vi "main_control_YJtoy_V2.vi"() -> ()   [LabVIEW 2021]
uses:
  Addons/DAQ_Pulse_Gen/DAQ_Control_2.ctl
  Addons/DAQ_Pulse_Gen/DAQ_Control_1.ctl
  Ver_2/Config_File_Paths_v2.ctl
  Ver_2/ZI_Data_v2.ctl
  Addons/DAQ_Pulse_Gen/DAQ_Control_3 .ctl
  <vilib>/Utility/file.llb/Write Delimited Spreadsheet (DBL).vi
  <vilib>/gmath/NumericalOptimization/Nonlinear Curve Fit LM formula string.vi
  <vilib>/Utility/error.llb/Error Cluster From Error Code.vi
  <vilib>/ErrorRing/Error Ring.xnode
  <vilib>/Utility/Data Type/NI_Data Type.lvlib
  <vilib>/Analysis/NI_AALPro.lvlib
  <vilib>/gmath/NI_Gmath.lvlib
panel:
  out "Initial State Numbers":i32
  out "Process name":string
  out "Initial_state_name":string
  out "tomography rotation memory (priv) 2":cluster{"Time":dbl[], dbl[]}[](array[cluster])
  out "MaxTime":dbl
  out "Process Array":cluster{"Timing 0":dbl[]}[](array[cluster])
  out "tomography rotation memory (priv)":cluster{"Time":dbl[], dbl[]}[](array[cluster])
  in  "pulses type (priv)":string[](array[string])=["None", "Y pi/2", "X pi/2"]
  in  "stop":bool
  in  "Tab Control":T1(tab)=enum."Design QPT"
  out "Config folder":string
  out "Chennel names\nare correct (?)":bool
  out "Channel map":map{string, i32}(c390)
  out "Pulses map [us]":map{string, dbl}(c390)
  out "Sampling data":T2={"Sample Numbers"=20000000, "Sample  Frequency (Hz)"=20000000}
  out "Resource Address":T3={"ZI Address"="DEV714", "VISA Keithley"="KEITHLEY"}
  in  "Save multi-process":bool
  in  "Period number":u32
  in  "Period [us]":dbl
  in  "Name of state (initial_state_)":string
  in  "Name of initial_state":u16(ring) items=["initial_state_01", "initial_state_02", "initial_state_03", "initial_state_04", "initial_state_05", "initial_state_06", "initial_state_07", "initial_state_08", "initial_state_09", "initial_state_10"]
  in  "Run tomography":bool
  in  "Run single FID":bool
  in  "Save for tomography":bool
  in  "Save single sequence":bool
  out "Pulses chart":cluster{dbl[], dbl[]}[](graph)
  in  "Reset sequence":bool
  in  "Channel":u16(ring) items=["LD pump", "LD repump", "LD probe", "pulse X", "pulse Y", "pulse Z", "Keithley ARM", "Keithley TRIG", "Accqusition TRIG", "Nonlinear coil", "None", "Tensor light shift", "pulse ZG"]
  in  "Add pulse advanced":bool
  in  "Physical channels":string[](array[string])
  in  "Add pulse":bool
  in  "Time [us]":dbl
  in  "Z pi/2":bool
  in  "Z pi":bool
  in  "Y pi/2":bool
  in  "Y pi":bool
  in  "X pi/2":bool
  in  "X pi":bool
  in  "Add pumping":bool
  in  "Pumping":T4(ring)
  in  "AOC":bool
  in  "X pi/4":bool
  in  "Save initial state":bool
  in  "Save  process":bool
  in  "Name of process (process_)":string
  in  "Name of process":u16(ring) items=["process_01", "process_02", "process_03", "process_04", "process_05", "process_06", "process_07", "process_08", "process_09", "process_10"]
  in  "Y pi/4":bool
  in  "Z pi/4":bool
  in  "Save multi Sequence":bool
  in  "Clear All processes":bool
  in  "Show Process_List":bool
  in  "Delete the Process":bool
  in  "Run QPT":bool
  in  "initial_state_show":u16(ring) items=["initial_state_01.ini", "initial_state_02.ini", "initial_state_03.ini", "initial_state_04.ini", "initial_state_05.ini", "initial_state_06.ini", "initial_state_07.ini", "initial_state_08.ini", "initial_state_09.ini", "initial_state_10.ini", "initial_state_11.ini"]
  in  "Choose init states":bool
  in  "State_update":bool
  out "State_List":string[](array[string]) caption="The Choosen States"
  in  "Delete init states":bool
  in  "Show init state":bool
  in  "Process_update":bool
  in  "Process_show":u16(ring) caption="initial_state_show" items=["process_01.ini", "process_02.ini", "process_03.ini"]
  out "Pulses chart 2":cluster{dbl[], dbl[]}[](graph)
  out "Pulses chart 3":cluster{dbl[], dbl[]}[](graph)
  in  "Save QPT":bool
  in  "Clear All states":bool
  out "Process_List":string[](array[string]) caption="The Choosen Process"
  in  "Choose the Process":bool
  in  "Multi-FID":bool
  in  "save":bool
  out "Rotation signal 3":cluster{"Time":dbl[], "Array":dbl[]}[](graph)
  out "w":dbl format="%#_3f"
  out "q":dbl format="%#_3f"
  out "g2":dbl format="%#_3f"
  out "g1":dbl format="%#_3f"
  out "C":dbl format="%#_3f"
  out "B":dbl format="%#_3f"
  out "A":dbl format="%#_3f"
  in  "Enum":T5(ring)
  in  "Fit model":bool
  out "Rotation signal":cluster{"Time":dbl[], dbl[]}(graph)
  out "Rotation spectrum":waveform(dbl)[](graph)
  out "Differential signal":cluster{"Time":dbl[], "X":dbl[]}[](graph)
  out "Intensity signal":cluster{"Time":dbl[], dbl[]}(graph)
  out "Polarimeter":dbl(knob) scale=-10.0..10.0
  in  "Run single FID 2":bool
  out "Progress":dbl(slide) scale=0.0..100.0
  in  "Number of repetition":u32=1 min=1 step=1
  in  "Signal in X or Y (?)":bool
  in  "Plot type":u16(ring) items=["None + [ None ]", "None + [ Y pi ]", "None + [ Z(pi/2)+Y(pi) ]", "Y pi/2 + [ None ]", "Y pi/2 + [ Y pi ]", "Y pi/2 + [ Z(pi/2)+Y(pi) ]", "X pi/2 + [ None ]", "X pi/2 + [ Y pi ]", "X pi/2 + [ Z(pi/2)+Y(pi) ]"]
  in  "Save raw data (?)":bool
  in  "Save CYCLOPS data (?)":bool
  out "Rotation signal":cluster{"Time":dbl[], dbl[]}(graph)
  in  "Run tomography 2":bool
  in  "Averaging":u8=1 min=1 step=1
  out "Differential signal":cluster{"Time":dbl[], "X":dbl[]}[](graph)
  out "Intensity signal":cluster{"Time":dbl[], dbl[]}(graph)
  out "Progress":dbl(slide) scale=0.0..100.0
  out "Rotation spectrum":waveform(dbl)[](graph)
  out "Rotation":cluster{"Time":dbl[], dbl[]}(graph)
  in  "Save raw data (?) 2":bool
  in  "Save CYCLOPS data (?) 2":bool
  out "Rotation spectrum 2":waveform(dbl)[](graph)
  out "Rotation signal 2":cluster{"Time":dbl[], dbl[]}(graph)
  out "Differential signal 2":cluster{"Time":dbl[], "X":dbl[]}[](graph)
  out "Intensity signal 2":cluster{"Time":dbl[], dbl[]}(graph)
  out "Single Tomography Progress":dbl(slide) scale=0.0..100.0
  out "Rotation 2":cluster{"Time":dbl[], dbl[]}(graph)
  in  "Averaging 2":u8=1 min=1 step=1
  in  "Run QPT 2":bool
  out "Current_QPT_order":i32
  out "QPT Progress":dbl(slide) scale=0.0..100.0
  # "To change that tab you need to go to block diagram"
  # "Probing will be added during saving"
  # "X"
  # "Y"
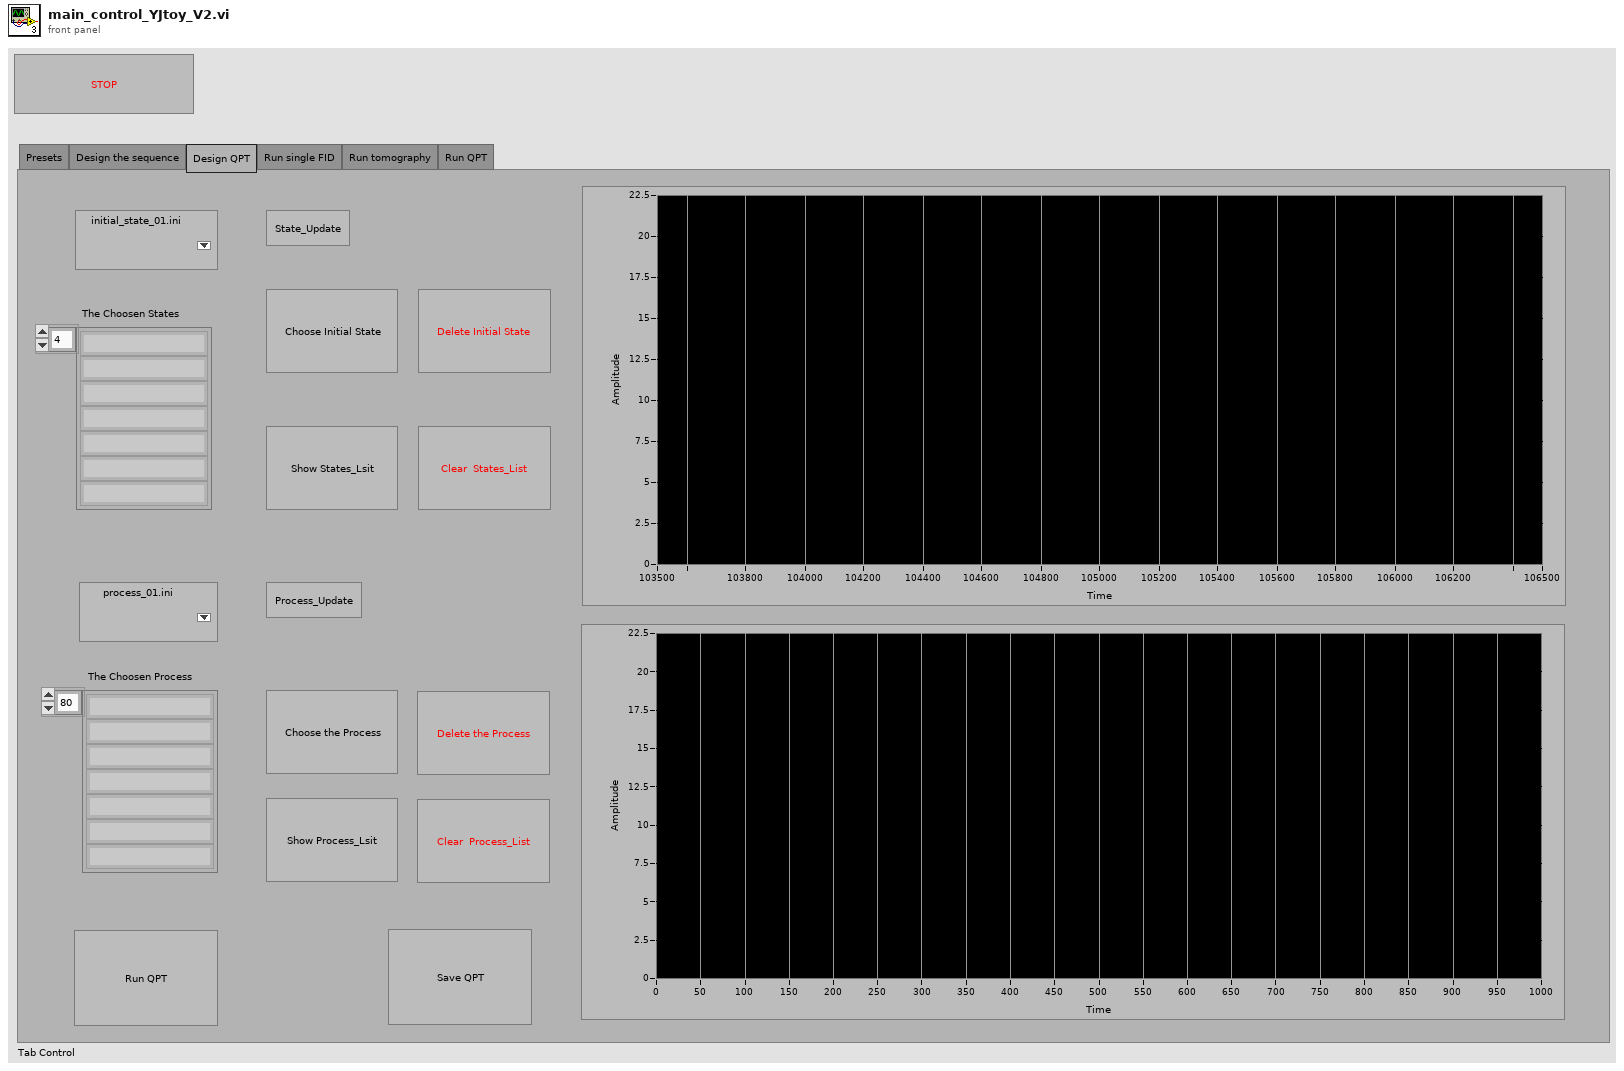
[diagram p1: front panel]
types:
  T1 = enum32{"Presets", "Design the sequence", "Design QPT", "Run single FID", "Run tomography", "Run QPT"}
  T2 = typedef "DAQ_Control_2.ctl" = cluster{"Sample Numbers":u32, "Sample  Frequency (Hz)":u32}
  T3 = cluster{"ZI Address":string, "VISA Keithley":refnum<visa-resource-name>}
  T4 = enum16{"Circular along X", "Linear in Y", "Linear in Z"}
  T5 = enum16{"Full", "A*Sin(w*t+q)*Exp(-g1*t)+C", "B*Exp(-q2*t)+C"}
  T6 = typedef "DAQ_Control_1.ctl" = cluster{"Port 2/line 6":cluster{"Timing 22":dbl[]}, "Port 2/line 5":cluster{"Timing 21":dbl[]}, "Port 2/line 4":cluster{"Timing 20":dbl[]}, "Port 2/line 3":cluster{"Timing 19":dbl[]}, "Port 2/line 2":cluster{"Timing 18":dbl[]}, "Port 2/line 1":cluster{"Timing 17":dbl[]}, "Port 2/line 0":cluster{"Timing 16":dbl[]}, "Port 1/line 7":cluster{"Timing 15":dbl[]}, "Port 1/line 6":cluster{"Timing 14":dbl[]}, "Port 1/line 5":cluster{"Timing 13":dbl[]}, "Port 1/line 4":cluster{"Timing 12":dbl[]}, "Port 1/line 3":cluster{"Timing 11":dbl[]}, "Port 1/line 2":cluster{"Timing 10":dbl[]}, "Port 1/line 1":cluster{"Timing 9":dbl[]}, "Port 1/line 0":cluster{"Timing 8":dbl[]}, "Port 0/line 7":cluster{"Timing 7\n":dbl[]}, "Port 0/line 6":cluster{"Timing 6\n":dbl[]}, "Port 0/line 5":cluster{"Timing 5\n":dbl[]}, "Port 0/line 4":cluster{"Timing 4\n":dbl[]}, "Port 0/line 3":cluster{"Timing 3\n":dbl[]}, "Port 0/line 2":cluster{"Timing 2":dbl[]}, "Port 0/line 1":cluster{"Timing 1\n":dbl[]}, "Port 0/line 0":cluster{"Timing 0":dbl[]}}
  T7 = typedef "Config_File_Paths_v2.ctl" = cluster{"ZI config file (.ini)":string, "Keithley config file (.ini)":string, "DAQ config file (.ini)":string}
  T8 = enum32{"Presets", "Design the sequence", "Design QPT", "Run single FID"}
  T9 = enum8{"Enabled", "Disabled", "Disabled and Grayed Out"}
  T10 = enum32{"Presets", "Design the sequence", "Design QPT", "Run single FID", "Run tomography"}
  T11 = cluster{"model":string, "Parameters":string[], "x":string}
  T12 = typedef "DAQ_Control_3 .ctl" = cluster{"Time Unit":enum16{"NanoSecond", "MicroSecond", "MilliSecond"}}
  T13 = typedef "ZI_Data_v2.ctl" = cluster{"R":dbl[], "Theta":dbl[], "X":dbl[], "Y":dbl[], "AuxIn0":dbl[], "AuxIn1":dbl[], "Frequency":dbl[], "DIO":dbl[], "Time":dbl[]}
  T14 = typedef "Resources_v2.ctl" = cluster{"ZI Handle":T15, "ZI ModHandle":T16, "VISA Keithley":refnum<visa-resource-name>}
  T15 = typedef "Zurich Instruments LabOne.lvlib/ziTypeHandle.ctl" = cluster{"handleValid":bool, "Conn":u64, "Path Prefix":string, "Handle":u64, "Connected":bool, "Clockbase(s)":dbl}
  T16 = typedef "Zurich Instruments LabOne.lvlib/ziTypeModHandle.ctl" = cluster{"handleValid":bool, "Conn":u64, "ModHandle":u64, "moduleID":string, "Path Prefix":string}
  T17 = typedef "Cutted_Data_v2.ctl" = cluster{"X":dbl[], "Y":dbl[], "Time":dbl[]}
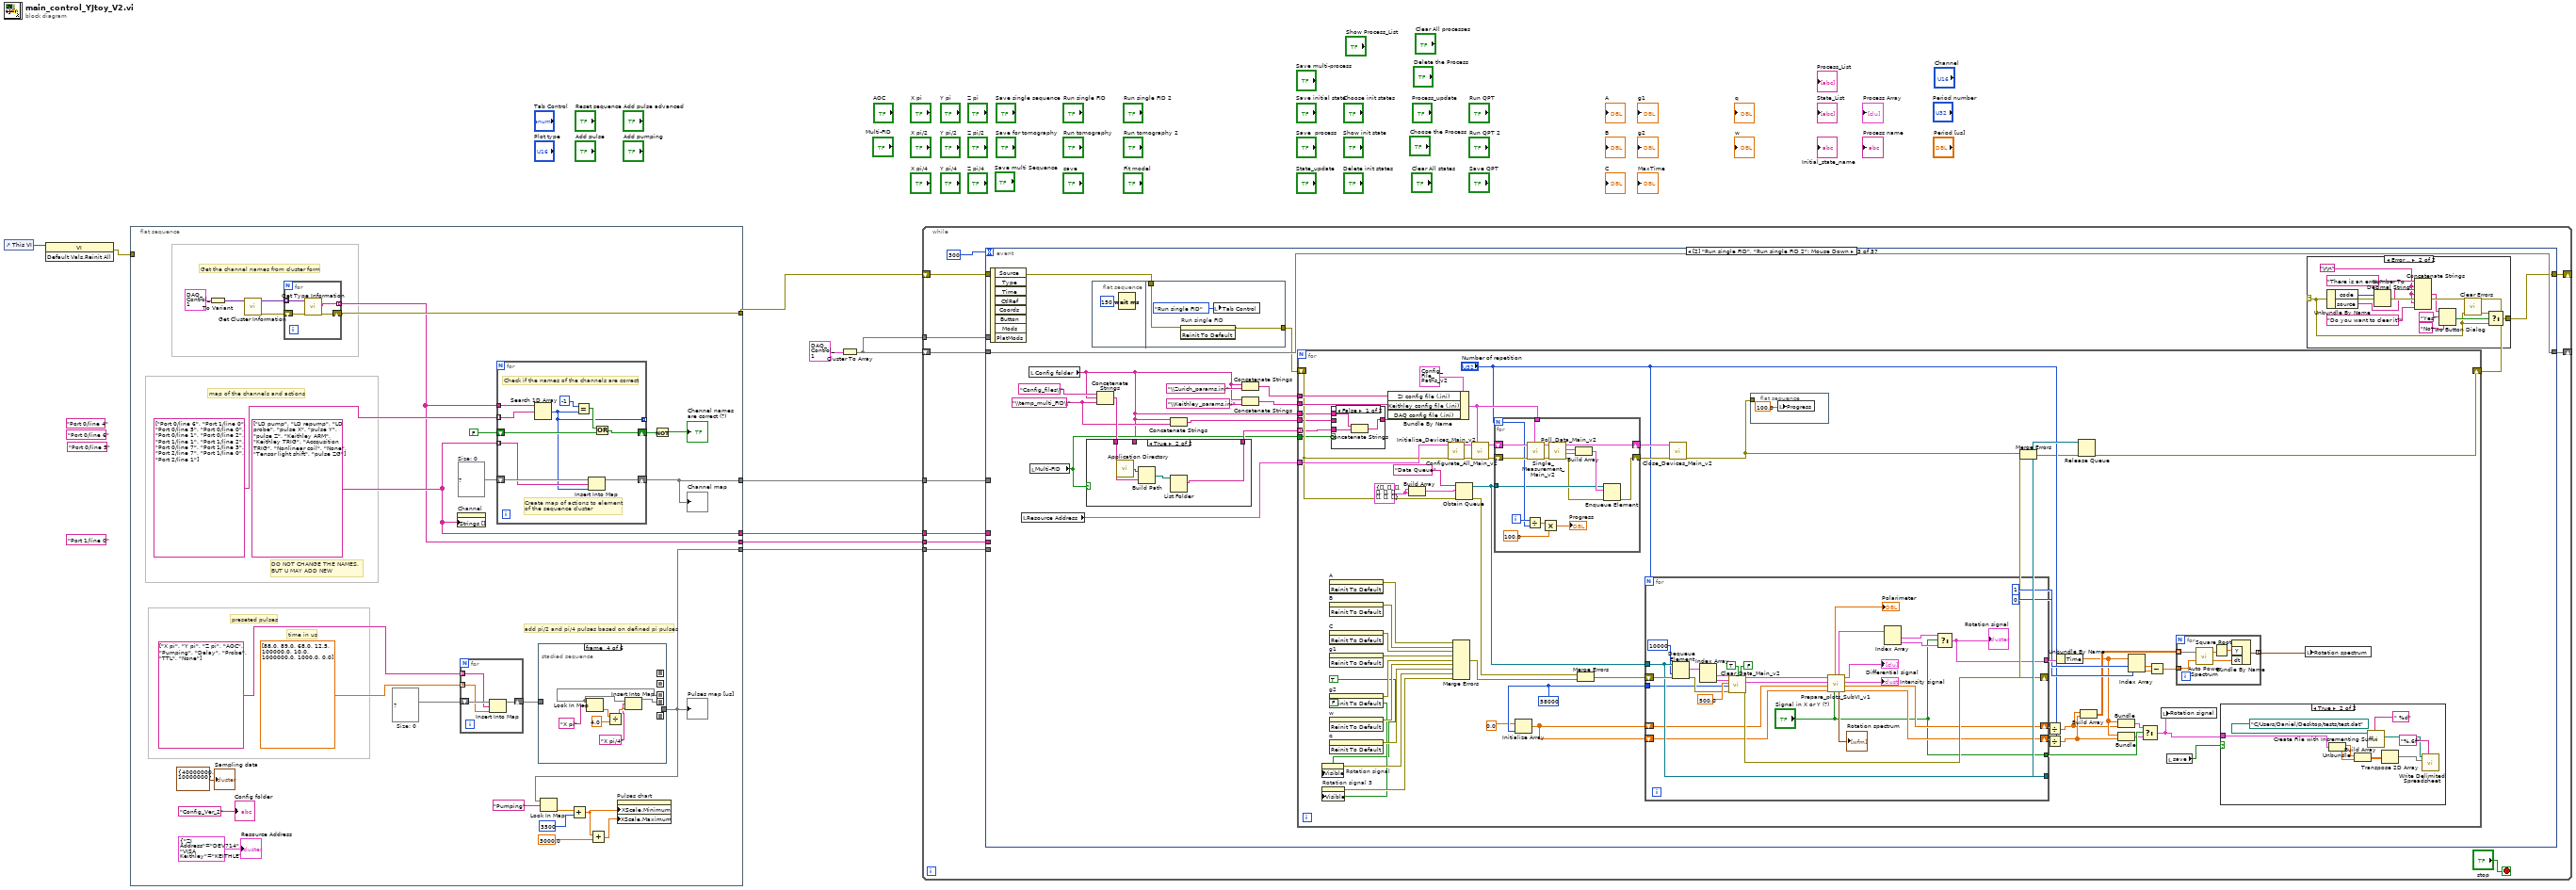
[diagram p0: block diagram]
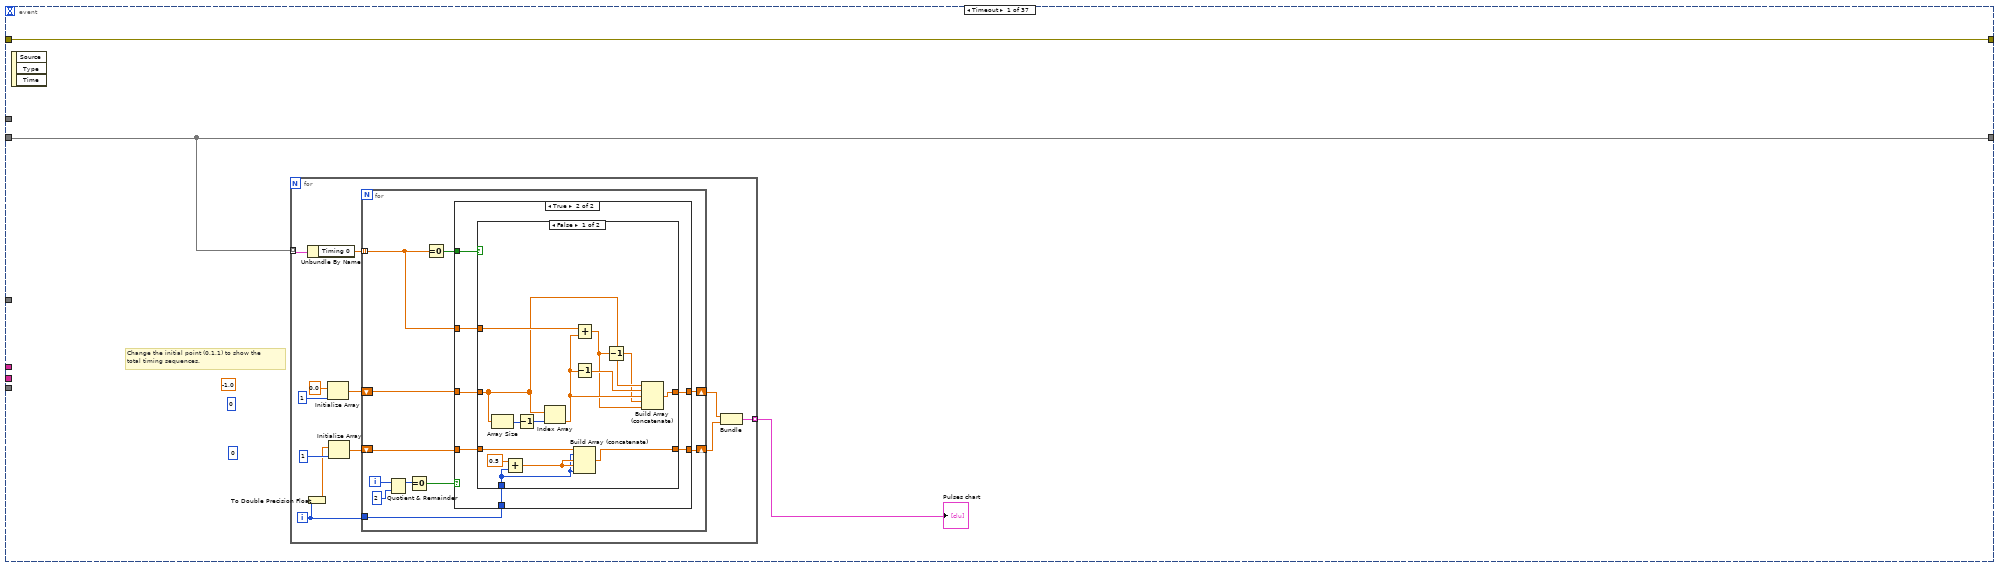
[diagram p2: hidden frame]
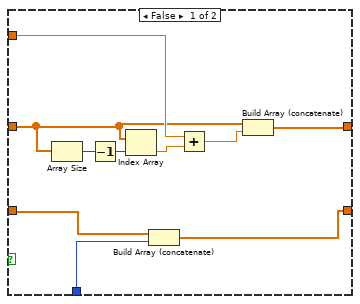
[diagram p3: hidden frame]
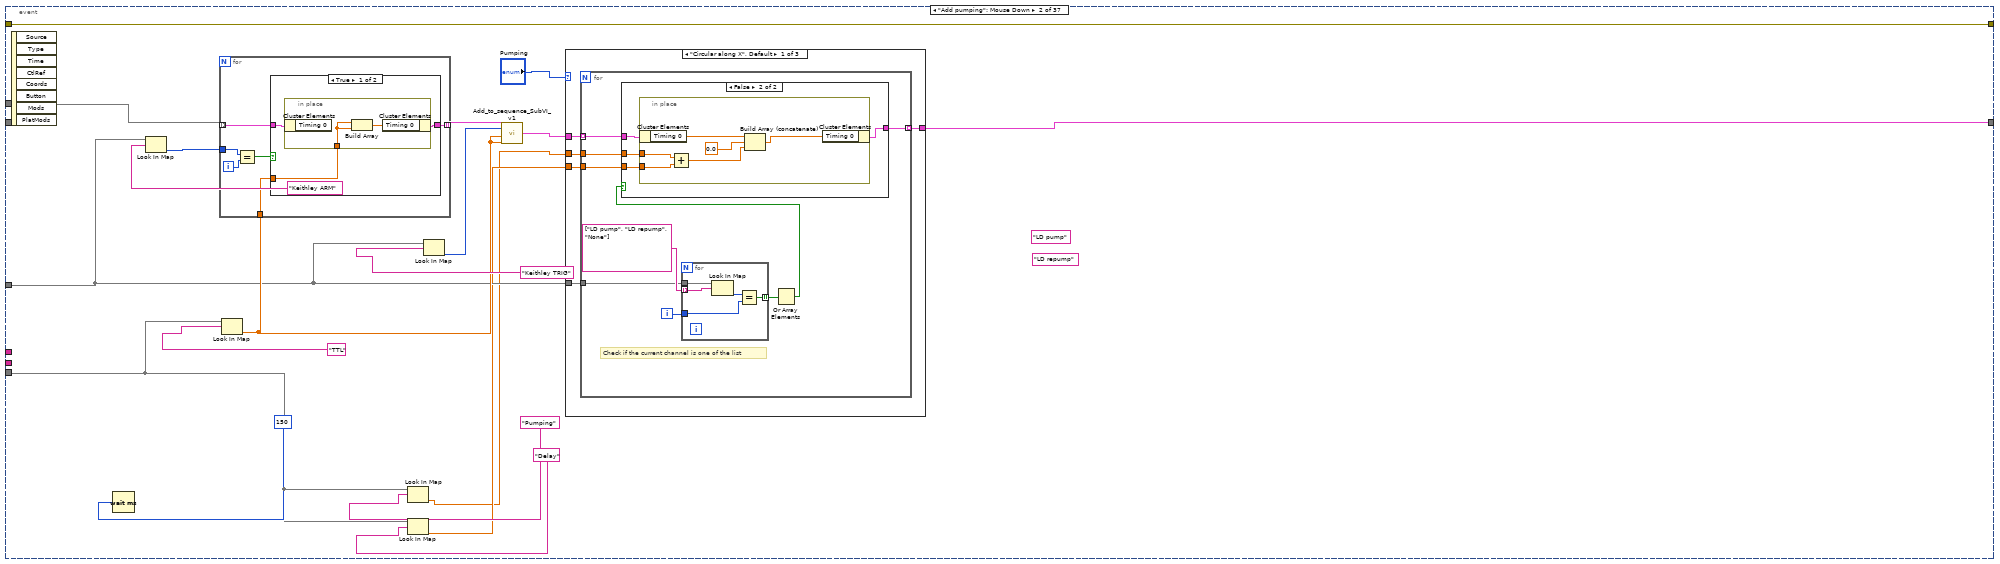
[diagram p5: hidden frame]
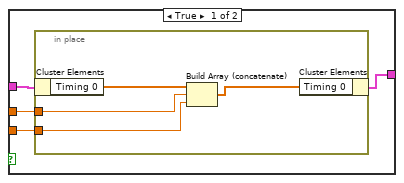
[diagram p6: hidden frame]
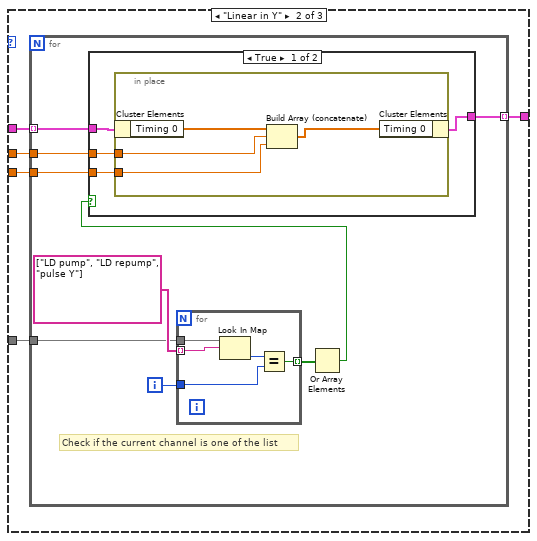
[diagram p7: hidden frame]
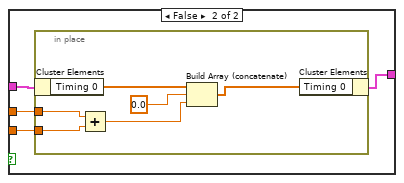
[diagram p8: hidden frame]
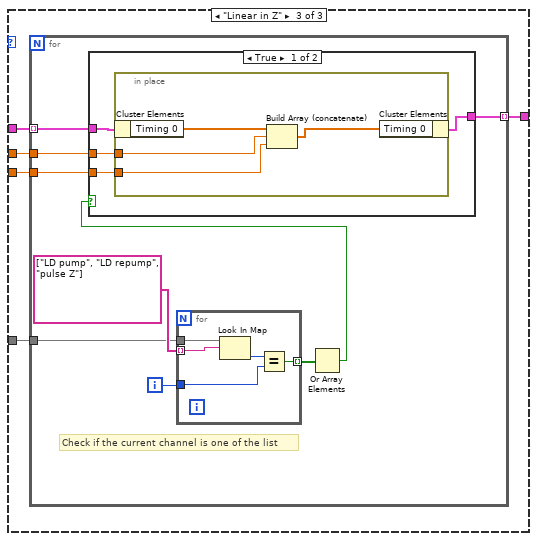
[diagram p9: hidden frame]
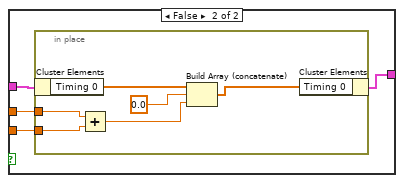
[diagram p10: hidden frame]
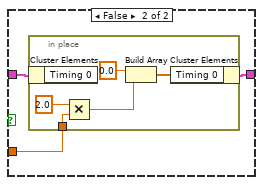
[diagram p11: hidden frame]
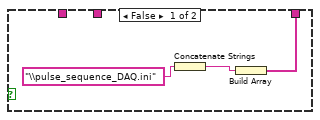
[diagram p12: hidden frame]
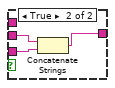
[diagram p13: hidden frame]
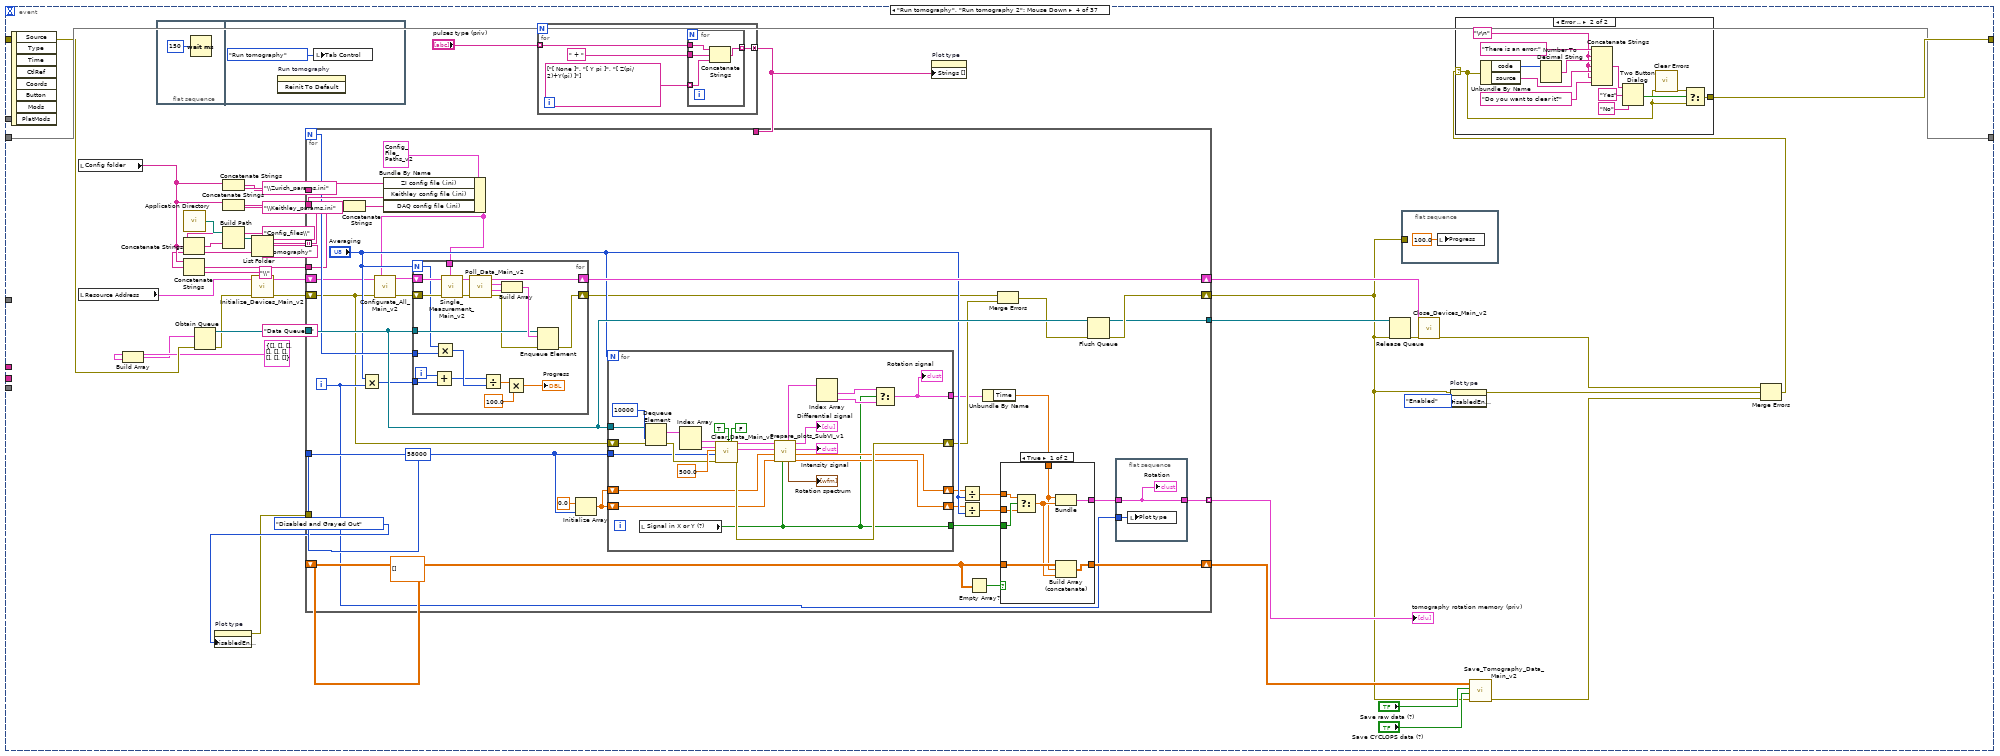
[diagram p16: hidden frame]
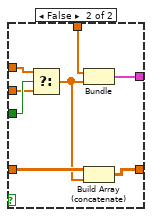
[diagram p17: hidden frame]
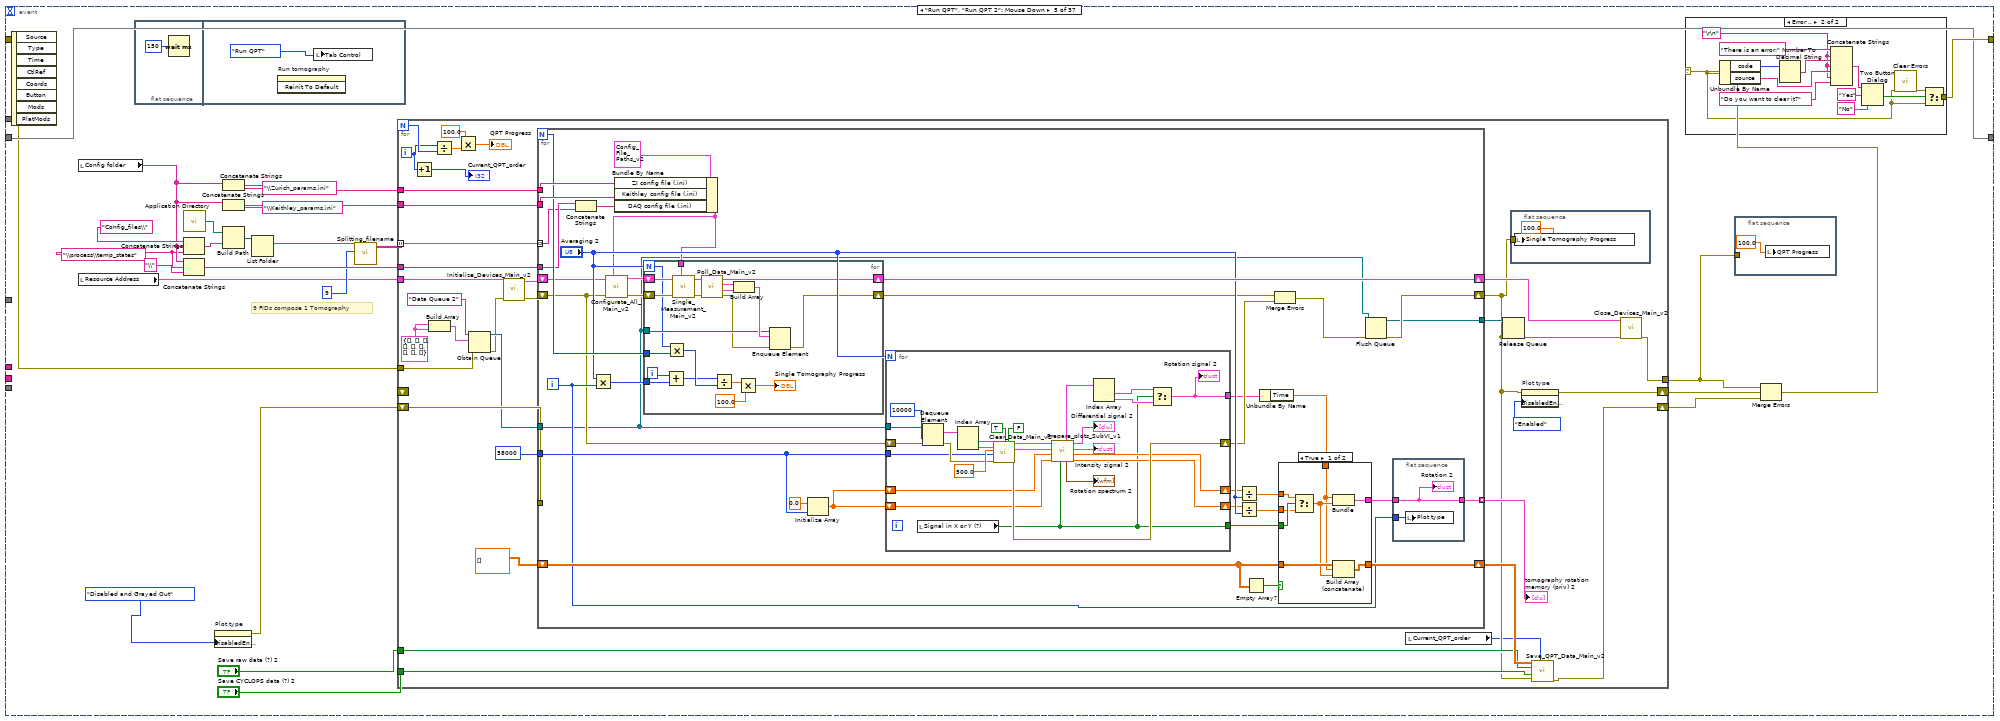
[diagram p19: hidden frame]
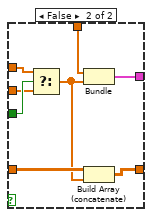
[diagram p20: hidden frame]
diagram:
  (unwired) "Port 0/line 5"
  (unwired) "Port 0/line 4"
  (unwired) "Port 1/line 0"
  (unwired) "Port 0/line 6"
  n1 = control-ref of="This VI"() -> (w2:refnum<vi>)
  n2 = invoke class="VI" method="Default Vals.Reinit All"(reference=w2) -> (error out=w1:errorcluster)  [unwired: 2 in, 2 out]
  n3 = flat-sequence {
    tunnel: [w23] -> w8
    tunnel: [w17] -> w7
    tunnel: [w22] -> w6
    tunnel: [w21] -> w5
    tunnel: [w20] -> w4
    tunnel: w1 -> [_]
    frame #0 {
      w27 = map{string, dbl} {}  # Size: 0
      w29 = map{string, i32} {}  # Size: 0
      w21 = string[] ["LD pump", "LD repump", "LD probe", "pulse X", "pulse Y", "pulse Z", "Keithley ARM", "Keithley TRIG", "Accqusition TRIG", "Nonlinear coil", "None", "Tensor light shift", "pulse ZG"]
      # "DO NOT CHANGE THE NAMES,\nBUT U MAY ADD NEW"
      # "add pi/2 and pi/4 pulses based on defined pi pulses"
      # "preseted pulses"
      # "time in us"
      # "map of the channels and actions"
      # "Get the channel names from cluster form"
      n4 = To Variant(anything=T6 {"Port 2/line 6"={"Timing 22"=[]}, "Port 2/line 5"={"Timing 21"=[]}, "Port 2/line 4"={"Timing 20"=[]}, "Port 2/line 3"={"Timing 19"=[]}, "Port 2/line 2"={"Timing 18"=[]}, "Port 2/line 1"={"Timing 17"=[]}, "Port 2/line 0"={"Timing 16"=[]}, "Port 1/line 7"={"Timing 15"=[]}, "Port 1/line 6"={"Timing 14"=[]}, "Port 1/line 5"={"Timing 13"=[]}, "Port 1/line 4"={"Timing 12"=[]}, "Port 1/line 3"={"Timing 11"=[]}, "Port 1/line 2"={"Timing 10"=[]}, "Port 1/line 1"={"Timing 9"=[]}, "Port 1/line 0"={"Timing 8"=[]}, "Port 0/line 7"={"Timing 7\n"=[]}, "Port 0/line 6"={"Timing 6\n"=[]}, "Port 0/line 5"={"Timing 5\n"=[]}, "Port 0/line 4"={"Timing 4\n"=[]}, "Port 0/line 3"={"Timing 3\n"=[]}, "Port 0/line 2"={"Timing 2"=[]}, "Port 0/line 1"={"Timing 1\n"=[]}, "Port 0/line 0"={"Timing 0"=[]}} ("Sequence")) -> (Variant=w35:variant)
      n5 = call <vilib>:"Get Cluster Information.vi"("variant"=w35) -> ("error out"=w34:errorcluster, "cluster elements"=w33:variant[])  [unwired: 9 in]
      n6 = for {
        tunnel: w33 -> [w96] mode=indexing
        shift-right: [w94] -> w22
        shift-left: w34 -> [w95]
        tunnel: [w93] -> w20 mode=indexing
        n7 = call <vilib>:"Get Type Information.vi"("error in (no error)"=w95, "variant"=w96) -> ("error out"=w94:errorcluster, "name"=w93:string)  [unwired: 5 in, 3 out]
      }
      n8 = property on="Channel" class="Ring (strict)"("Strings []"=w21) -> ()  [unwired: 2 in, 2 out]
      n9 = for {
        shift-right: [w79] -> w24
        shift-left: w27 -> [w82]
        tunnel: string[] ["X pi", "Y pi", "Z pi", "AOC", "Pumping", "Delay", "Probe", "TTL", "None"] -> [w81] mode=indexing
        tunnel: dbl[] [88.0, 89.0, 68.0, 12.5, 100000.0, 10.0, 1000000.0, 1000.0, 0.0] -> [w80] mode=indexing
        n10 = Insert Into Map(map in=w82, key=w81, value=w80) -> (map out=w79:map{string, dbl})  [unwired: 2 out]
      }
      n11 = for {
        tunnel: w20 -> [w92]
        tunnel: string[] ["Port 0/line 6", "Port 1/line 0", "Port 0/line 5", "Port 0/line 0", "Port 0/line 1", "Port 0/line 2", "Port 1/line 1", "Port 1/line 2", "Port 0/line 7", "Port 1/line 3", "Port 2/line 7", "Port 1/line 0", "Port 2/line 1"] -> [w83] mode=indexing
        shift-right: [w88] -> w31
        shift-left: FALSE -> [w89]
        tunnel: [w85] -> _ mode=indexing
        shift-right: [w84] -> w23
        shift-left: w29 -> [w87]
        tunnel: w21 -> [w86] mode=indexing
        # "Create map of actions to element\nof the sequence cluster"
        # "Check if the names of the channels are correct"
        n12 = Search 1D Array(1D array=w92, element=w83) -> (index of element=w85:i32)  [unwired: 1 in]
        n13 = Equal?(x=-1, y=w85) -> (x = y?=w90:bool)
        n14 = Insert Into Map(map in=w87, key=w86, value=w85) -> (map out=w84:map{string, i32})  [unwired: 2 out]
        n15 = Or(x=w90, y=w89) -> (x .or. y?=w88:bool)
      }
      "Channel map" <- w23
      n16 = stacked-sequence {
        seq-local: [w37 _ _ _ _ _] -> [_ w44 _ _ _ _]
        seq-local: [_ w45 _ _ _ _] -> [_ _ w52 _ _ _]
        seq-local: [_ _ w51 _ _ _] -> [_ _ _ w63 _ _]
        seq-local: [_ _ _ w59 _ _] -> [_ _ _ _ w71 _]
        seq-local: [_ _ _ _ w70 _] -> [_ _ _ _ _ w78]
        tunnel: w24 -> [w41 _ _ _ _ _]
        tunnel: [_ _ _ _ _ w77] -> w17
        frame #0 {
          n17 = Look In Map(map=w41, key="X pi") -> (value=w39:dbl)  [unwired: 1 in, 1 out]
          n18 = Divide(x=w39, y=2.0) -> (x/y=w40:dbl)
          n19 = Insert Into Map(map in=w41, key="X pi/2", value=w40) -> (map out=w37:map{string, dbl})  [unwired: 2 out]
        }
        frame #1 {
          n20 = Look In Map(map=w44, key="Y pi") -> (value=w50:dbl)  [unwired: 1 in, 1 out]
          n21 = Divide(x=w50, y=2.0) -> (x/y=w49:dbl)
          n22 = Insert Into Map(map in=w44, key="Y pi/2", value=w49) -> (map out=w45:map{string, dbl})  [unwired: 2 out]
        }
        frame #2 {
          n23 = Look In Map(map=w52, key="Z pi") -> (value=w54:dbl)  [unwired: 1 in, 1 out]
          n24 = Divide(x=w54, y=2.0) -> (x/y=w55:dbl)
          n25 = Insert Into Map(map in=w52, key="Z pi/2", value=w55) -> (map out=w51:map{string, dbl})  [unwired: 2 out]
        }
        frame #3 {
          n26 = Look In Map(map=w63, key="X pi") -> (value=w62:dbl)  [unwired: 1 in, 1 out]
          n27 = Divide(x=w62, y=4.0) -> (x/y=w60:dbl)
          n28 = Insert Into Map(map in=w63, key="X pi/4", value=w60) -> (map out=w59:map{string, dbl})  [unwired: 2 out]
        }
        frame #4 {
          n29 = Look In Map(map=w71, key="Y pi") -> (value=w68:dbl)  [unwired: 1 in, 1 out]
          n30 = Divide(x=w68, y=4.0) -> (x/y=w66:dbl)
          n31 = Insert Into Map(map in=w71, key="Y pi/4", value=w66) -> (map out=w70:map{string, dbl})  [unwired: 2 out]
        }
        frame #5 {
          n32 = Look In Map(map=w78, key="Z pi") -> (value=w75:dbl)  [unwired: 1 in, 1 out]
          n33 = Divide(x=w75, y=4.0) -> (x/y=w73:dbl)
          n34 = Insert Into Map(map in=w78, key="Z pi/4", value=w73) -> (map out=w77:map{string, dbl})  [unwired: 2 out]
        }
      }
      "Pulses map [us]" <- w17
      n35 = Look In Map(map=w17, key="Pumping") -> (value=w19:dbl)  [unwired: 1 in, 1 out]
      n36 = Add(x=w19, y=3500) -> (x+y=w16:dbl)
      n37 = Add(x=w16, y=3000.0) -> (x+y=w14:dbl)
      n38 = property on="Pulses chart" class="XYGraph (strict)"("XScale.Minimum"=w16, "XScale.Maximum"=w14) -> ()  [unwired: 2 in, 2 out]
      n39 = Not(x=w31) -> (.not. x?=→"Chennel names\nare correct (?)":bool)
      "Sampling data" <- T2 {"Sample Numbers"=40000000, "Sample  Frequency (Hz)"=10000000} ("Sampling data")
      "Config folder" <- "Config_Ver_2" ("Filename (ini)")
      "Resource Address" <- T3 {"ZI Address"="DEV714", "VISA Keithley"="KEITHLEY"} ("Resource Address")
    }
  }
  n40 = Cluster To Array(cluster=T6 {"Port 2/line 6"={"Timing 22"=[]}, "Port 2/line 5"={"Timing 21"=[]}, "Port 2/line 4"={"Timing 20"=[]}, "Port 2/line 3"={"Timing 19"=[]}, "Port 2/line 2"={"Timing 18"=[]}, "Port 2/line 1"={"Timing 17"=[]}, "Port 2/line 0"={"Timing 16"=[]}, "Port 1/line 7"={"Timing 15"=[]}, "Port 1/line 6"={"Timing 14"=[]}, "Port 1/line 5"={"Timing 13"=[]}, "Port 1/line 4"={"Timing 12"=[]}, "Port 1/line 3"={"Timing 11"=[]}, "Port 1/line 2"={"Timing 10"=[]}, "Port 1/line 1"={"Timing 9"=[]}, "Port 1/line 0"={"Timing 8"=[]}, "Port 0/line 7"={"Timing 7\n"=[]}, "Port 0/line 6"={"Timing 6\n"=[]}, "Port 0/line 5"={"Timing 5\n"=[]}, "Port 0/line 4"={"Timing 4\n"=[]}, "Port 0/line 3"={"Timing 3\n"=[]}, "Port 0/line 2"={"Timing 2"=[]}, "Port 0/line 1"={"Timing 1\n"=[]}, "Port 0/line 0"={"Timing 0"=[]}} ("Sequence")) -> (array=w3:cluster{"Timing 0":dbl[]}[])
  n41 = while {
    shift-right: [w98] -> _
    shift-left: w3 -> [w107]
    tunnel: w8 -> [w106]
    tunnel: w7 -> [w97]
    shift-right: [w102] -> _
    shift-left: w6 -> [w103]
    tunnel: w5 -> [w101]
    tunnel: w4 -> [w100]
    tunnel: w3 -> [w99]
    stop <- "stop" stop-if-true
    n42 = event shown="[2] \"Run single FID\", \"Run single FID 2\": Mouse Down" {
      selector: _ -> [_ _ _ _ _ _ _ _ _ _ _ _ _ _ _ _ _ _ _ _ _ _ _ _ _ _ _ _ _ _ _ _ _ _ _ _ _]
      dyn-events: _ -> [_ _ _ _ _ _ _ _ _ _ _ _ _ _ _ _ _ _ _ _ _ _ _ _ _ _ _ _ _ _ _ _ _ _ _ _ _]
      timeout: 300 -> [_ _ _ _ _ _ _ _ _ _ _ _ _ _ _ _ _ _ _ _ _ _ _ _ _ _ _ _ _ _ _ _ _ _ _ _ _]
      tunnel: w107 -> [w110 _ w327 w520 w675 w838 _ w1001 w1006 w1018 w1029 w1041 w1053 w1065 w1077 w1089 w1101 w1118 w1146 w1185 w1266 w1397 w1451 w1593 w1640 _ _ _ _ _ _ _ _ _ _ _ _]
      tunnel: w106 -> [_ w172 _ _ _ _ _ w985 w1013 w1025 w1036 w1048 w1060 w1072 w1084 w1096 w1108 w1123 _ w1198 w1268 w1399 w1456 _ _ w1713 _ _ _ _ _ _ _ _ _ _ _]
      tunnel: w97 -> [_ w171 _ _ _ _ _ w983 w1007 w1019 w1034 w1042 w1054 w1066 w1078 w1090 w1102 w1119 w1138 w1195 w1267 w1398 w1455 _ _ w1712 _ _ _ _ _ _ _ _ _ _ _]
      tunnel: [w110 w169 w327 w520 w675 w838 _ w978 w1005 w1017 w1028 w1040 w1052 w1064 w1076 w1088 w1100 w1117 w1135 w1185 _ _ w1451 w1593 w1640 _ _ _ _ _ _ _ _ _ _ _ w2166] -> w98
      tunnel: w103 -> [w109 w185 w326 w514 w657 w839 w881 w989 w1009 w1021 _ w1044 w1056 w1068 w1080 w1092 w1104 w1121 w1142 w1180 w1258 w1389 w1449 w1594 w1641 w1696 w1828 w1923 w2021 w2044 w2059 w2080 w2101 w2129 w2157 w2163 w2167]
      tunnel: [w109 w185 w324 w524 w678 w839 _ w989 w1009 w1021 _ w1044 w1056 w1068 w1080 w1092 w1104 w1121 w1142 w1179 w1265 w1396 w1448 w1595 w1642 w1719 w1827 w1916 w2016 w2039 w2066 w2087 w2098 w2126 w2156 w2162 w2167] -> w102
      tunnel: w101 -> [_ _ _ _ _ _ _ _ _ _ _ _ _ _ _ _ _ w1114 _ _ _ _ _ _ _ _ _ _ _ _ _ _ _ _ _ _ _]
      tunnel: w100 -> [_ _ _ _ _ _ _ _ _ _ _ _ _ _ _ _ _ _ w1144 _ _ _ _ _ _ _ _ _ _ _ _ _ _ _ _ _ _]
      tunnel: w99 -> [_ w168 _ _ _ _ _ _ _ _ _ _ _ _ _ _ _ _ _ _ _ _ _ _ _ _ _ _ _ _ _ _ _ _ _ _ w2166]
      event Timeout {
        (unwired) 0 ("dimension size")
        (unwired) 0 ("dimension size")
        (unwired) -1.0 ("element")
        # "Change the initial point (0,1,1) to show the \ntotal timing sequences."
        n43 = event-data() -> ()  [unwired: 1 in, 3 out]
        n44 = for {
          tunnel: w110 -> [w122] mode=indexing
          tunnel: [w111] -> w108 mode=indexing
          i -> [w114]
          n45 = To Double Precision Float(number=w114) -> (double precision float=w118:dbl)
          n46 = Unbundle By Name(w122) -> ("Timing 0"=w121:dbl[])
          n47 = Initialize Array(0.0 ("element"), 1 ("dimension size")) -> (w115:dbl[])
          n48 = Initialize Array(w118, 1 ("dimension size")) -> (w119:dbl[])
          n49 = for {
            tunnel: w121 -> [w124] mode=indexing
            shift-right: [w126] -> w112
            shift-left: w119 -> [w125]
            shift-right: [w128] -> w113
            shift-left: w115 -> [w127]
            tunnel: w114 -> [w123]
            i -> [w133]
            n50 = Quotient & Remainder(x=w133, y=2) -> (x-y*floor(x/y)=w131:i32)  [unwired: 1 out]
            n51 = Equal To 0?(x=w131) -> (x = 0?=w130:bool)
            n52 = Equal To 0?(x=w124) -> (x = 0?=w129:bool)
            n53 = case shown="True" w130 {
              tunnel: w129 -> [_ w150]
              tunnel: [w134 w149] -> w128
              tunnel: w127 -> [w136 w148]
              tunnel: [w141 w147] -> w126
              tunnel: w125 -> [w142 w146]
              tunnel: w124 -> [w137 w145]
              tunnel: w123 -> [w143 w144]
              frame False {
                n54 = Array Size(array=w136) -> (size(s)=w140:i32)
                n55 = Decrement(x=w140) -> (x-1=w139:i32)
                n56 = Index Array(array=w136, index=w139) -> (element=w138:dbl)
                n57 = Build Array (concatenate)(w142, w143) -> (w141:dbl[])
                n58 = Add(x=w137, y=w138) -> (x+y=w135:dbl)
                n59 = Build Array (concatenate)(w136, w135) -> (w134:dbl[])
              }
              frame True {
                n60 = case shown="False" w150 {
                  tunnel: [w161 w166] -> w149
                  tunnel: w148 -> [w155 w166]
                  tunnel: [w157 w165] -> w147
                  tunnel: w146 -> [w164 w165]
                  tunnel: w145 -> [w162 _]
                  tunnel: w144 -> [w158 _]
                  frame False {
                    n61 = Array Size(array=w155) -> (size(s)=w163:i32)
                    n62 = Add(x=0.5, y=w158) -> (x+y=w159:dbl)
                    n63 = Decrement(x=w163) -> (x-1=w156:i32)
                    n64 = Index Array(array=w155, index=w156) -> (element=w153:dbl)
                    n65 = Add(x=w162, y=w153) -> (x+y=w152:dbl)
                    n66 = Decrement(x=w153) -> (x-1=w154:dbl)
                    n67 = Build Array (concatenate)(w164, w158, w159, w159, w158) -> (w157:dbl[])
                    n68 = Decrement(x=w152) -> (x-1=w151:dbl)
                    n69 = Build Array (concatenate)(w155, w154, w153, w151, w152) -> (w161:dbl[])
                  }
                  frame True {
                  }
                }
              }
            }
          }
          n70 = Bundle(w113, w112) -> (w111:cluster{dbl[], dbl[]})  [unwired: 1 in]
        }
        "Pulses chart" <- w108
      }
      event "Add pumping": Mouse Down {
        (unwired) "LD pump" ("key")
        (unwired) "LD repump" ("key")
        n71 = event-data() -> ()  [unwired: 1 in, 8 out]
        n72 = Wait (ms)(milliseconds to wait=u32 150) -> ()  [unwired: 1 out]
        n73 = Look In Map(map=w172, key="Keithley ARM") -> (value=w182:i32)  [unwired: 1 in, 1 out]
        n74 = Look In Map(map=w171, key="TTL") -> (value=w177:dbl)  [unwired: 1 in, 1 out]
        n75 = for {
          tunnel: w168 -> [w299] mode=indexing
          tunnel: w182 -> [w301]
          tunnel: w177 -> [w298]
          tunnel: [w297] -> w180 mode=indexing
          i -> [w302]
          n76 = Equal?(x=w301, y=w302) -> (x = y?=w300:bool)
          n77 = case shown="True" w300 {
            tunnel: w299 -> [w305 w310]
            tunnel: w298 -> [w304 w309]
            tunnel: [w303 w308] -> w297
            frame True {
              n78 = in-place {
                in-place-border: w304 -> [w307]
                n79 = in-place-cluster #1(w305) -> ()  [unwired: 1 out]
                n80 = Build Array(w307, w307) -> (w306:dbl[])
                n81 = in-place-cluster #1("Timing 0"=w306) -> (w303:cluster{"Timing 0":dbl[]})
              }
            }
            frame False {
              n82 = in-place {
                in-place-border: w309 -> [w313]
                n83 = in-place-cluster #2(w310) -> ()  [unwired: 1 out]
                n84 = Multiply(x=2.0, y=w313) -> (x*y=w311:dbl)
                n85 = Build Array(0.0 ("element"), w311) -> (w315:dbl[])
                n86 = in-place-cluster #2("Timing 0"=w315) -> (w308:cluster{"Timing 0":dbl[]})
              }
            }
          }
        }
        n87 = Look In Map(map=w171, key="Pumping") -> (value=w167:dbl)  [unwired: 1 in, 1 out]
        n88 = Look In Map(map=w171, key="Delay") -> (value=w170:dbl)  [unwired: 1 in, 1 out]
        n89 = Look In Map(map=w172, key="Keithley TRIG") -> (value=w178:i32)  [unwired: 1 in, 1 out]
        n90 = call "Add_to_sequence_SubVI_v1.vi"("Delay [us]"=w177, "Pulse length [us]"=w177, "Channel number"=w178, "Array sequence in"=w180) -> ("Array sequence out"=w175:cluster{"Timing 0":dbl[]}[])
        n91 = case shown="\"Circular along X\", Default" "Pumping" {
          tunnel: w175 -> [w190 w227 w264]
          tunnel: w172 -> [w189 w226 w263]
          tunnel: w167 -> [w188 w225 w262]
          tunnel: w170 -> [w187 w224 w261]
          tunnel: [w186 w223 w260] -> w169
          frame "Circular along X", Default {
            n92 = for {
              tunnel: w190 -> [w194] mode=indexing
              tunnel: w189 -> [w196]
              tunnel: w188 -> [w193]
              tunnel: w187 -> [w192]
              tunnel: [w191] -> w186 mode=indexing
              i -> [w197]
              # "Check if the current channel is one of the list"
              n93 = for {
                tunnel: w196 -> [w221]
                tunnel: w197 -> [w220]
                tunnel: [w219] -> w199 mode=indexing
                tunnel: string[] ["LD pump", "LD repump", "None"] -> [w218] mode=indexing
                n94 = Look In Map(map=w221, key=w218) -> (value=w222:i32)  [unwired: 1 in, 1 out]
                n95 = Equal?(x=w222, y=w220) -> (x = y?=w219:bool)
              }
              n96 = Or Array Elements(Boolean array=w199) -> (logical OR=w195:bool)
              n97 = case shown="False" w195 {
                tunnel: w194 -> [w203 w211]
                tunnel: w193 -> [w202 w210]
                tunnel: w192 -> [w201 w209]
                tunnel: [w200 w208] -> w191
                frame True {
                  n98 = in-place {
                    in-place-border: w202 -> [w206]
                    in-place-border: w201 -> [w205]
                    n99 = in-place-cluster #3(w203) -> ("Timing 0"=w207:dbl[])
                    n100 = Build Array (concatenate)(w207, w206, w205) -> (w204:dbl[])
                    n101 = in-place-cluster #3("Timing 0"=w204) -> (w200:cluster{"Timing 0":dbl[]})
                  }
                }
                frame False {
                  n102 = in-place {
                    in-place-border: w210 -> [w215]
                    in-place-border: w209 -> [w214]
                    n103 = in-place-cluster #4(w211) -> ("Timing 0"=w217:dbl[])
                    n104 = Add(x=w215, y=w214) -> (x+y=w213:dbl)
                    n105 = Build Array (concatenate)(w217, 0.0 ("element"), w213) -> (w216:dbl[])
                    n106 = in-place-cluster #4("Timing 0"=w216) -> (w208:cluster{"Timing 0":dbl[]})
                  }
                }
              }
            }
          }
          frame "Linear in Y" {
            n107 = for {
              tunnel: w227 -> [w231] mode=indexing
              tunnel: w226 -> [w233]
              tunnel: w225 -> [w230]
              tunnel: w224 -> [w229]
              tunnel: [w228] -> w223 mode=indexing
              i -> [w234]
              # "Check if the current channel is one of the list"
              n108 = for {
                tunnel: w233 -> [w258]
                tunnel: w234 -> [w257]
                tunnel: [w256] -> w236 mode=indexing
                tunnel: string[] ["LD pump", "LD repump", "pulse Y"] -> [w255] mode=indexing
                n109 = Look In Map(map=w258, key=w255) -> (value=w259:i32)  [unwired: 1 in, 1 out]
                n110 = Equal?(x=w259, y=w257) -> (x = y?=w256:bool)
              }
              n111 = Or Array Elements(Boolean array=w236) -> (logical OR=w232:bool)
              n112 = case shown="True" w232 {
                tunnel: w231 -> [w240 w248]
                tunnel: w230 -> [w239 w247]
                tunnel: w229 -> [w238 w246]
                tunnel: [w237 w245] -> w228
                frame True {
                  n113 = in-place {
                    in-place-border: w239 -> [w243]
                    in-place-border: w238 -> [w242]
                    n114 = in-place-cluster #5(w240) -> ("Timing 0"=w244:dbl[])
                    n115 = Build Array (concatenate)(w244, w243, w242) -> (w241:dbl[])
                    n116 = in-place-cluster #5("Timing 0"=w241) -> (w237:cluster{"Timing 0":dbl[]})
                  }
                }
                frame False {
                  n117 = in-place {
                    in-place-border: w247 -> [w252]
                    in-place-border: w246 -> [w251]
                    n118 = in-place-cluster #6(w248) -> ("Timing 0"=w254:dbl[])
                    n119 = Add(x=w252, y=w251) -> (x+y=w250:dbl)
                    n120 = Build Array (concatenate)(w254, 0.0 ("element"), w250) -> (w253:dbl[])
                    n121 = in-place-cluster #6("Timing 0"=w253) -> (w245:cluster{"Timing 0":dbl[]})
                  }
                }
              }
            }
          }
          frame "Linear in Z" {
            n122 = for {
              tunnel: w264 -> [w268] mode=indexing
              tunnel: w263 -> [w270]
              tunnel: w262 -> [w267]
              tunnel: w261 -> [w266]
              tunnel: [w265] -> w260 mode=indexing
              i -> [w271]
              # "Check if the current channel is one of the list"
              n123 = for {
                tunnel: w270 -> [w295]
                tunnel: w271 -> [w294]
                tunnel: [w293] -> w273 mode=indexing
                tunnel: string[] ["LD pump", "LD repump", "pulse Z"] -> [w292] mode=indexing
                n124 = Look In Map(map=w295, key=w292) -> (value=w296:i32)  [unwired: 1 in, 1 out]
                n125 = Equal?(x=w296, y=w294) -> (x = y?=w293:bool)
              }
              n126 = Or Array Elements(Boolean array=w273) -> (logical OR=w269:bool)
              n127 = case shown="True" w269 {
                tunnel: w268 -> [w277 w285]
                tunnel: w267 -> [w276 w284]
                tunnel: w266 -> [w275 w283]
                tunnel: [w274 w282] -> w265
                frame True {
                  n128 = in-place {
                    in-place-border: w276 -> [w280]
                    in-place-border: w275 -> [w279]
                    n129 = in-place-cluster #7(w277) -> ("Timing 0"=w281:dbl[])
                    n130 = Build Array (concatenate)(w281, w280, w279) -> (w278:dbl[])
                    n131 = in-place-cluster #7("Timing 0"=w278) -> (w274:cluster{"Timing 0":dbl[]})
                  }
                }
                frame False {
                  n132 = in-place {
                    in-place-border: w284 -> [w289]
                    in-place-border: w283 -> [w288]
                    n133 = in-place-cluster #8(w285) -> ("Timing 0"=w291:dbl[])
                    n134 = Add(x=w289, y=w288) -> (x+y=w287:dbl)
                    n135 = Build Array (concatenate)(w291, 0.0 ("element"), w287) -> (w290:dbl[])
                    n136 = in-place-cluster #8("Timing 0"=w290) -> (w282:cluster{"Timing 0":dbl[]})
                  }
                }
              }
            }
          }
        }
      }
      event "Run single FID", "Run single FID 2": Mouse Down {
        w319 = "\\temp_multi_FID\\" ("string")
        n137 = event-data() -> ()  [unwired: 1 in, 8 out]
        n138 = local read "Resource Address"() -> (w332:T3)
        n139 = local read "Config folder"() -> (w316:string)
        n140 = local read "Multi-FID"() -> (w317:bool)
        n141 = flat-sequence {
          tunnel: w326 -> [w484]
          tunnel: [w483] -> w325
          frame #0 {
            n142 = Wait (ms)(milliseconds to wait=u32 150) -> ()  [unwired: 1 out]
          }
          frame #1 {
            n143 = invoke on="Run single FID" class="Bool (strict)" method="Reinit To Default"(error in=w484) -> (error out=w483:errorcluster)  [unwired: 2 in, 2 out]
            n144 = local write "Tab Control"(T8."Run single FID" ("Tab Control")) -> ()
          }
        }
        n145 = Concatenate Strings("Config_files\\" ("string"), w316, w319) -> (w320:string)
        n146 = case shown="True" w317 {
          tunnel: w320 -> [_ w337]
          tunnel: [w333 w336] -> w322
          tunnel: w316 -> [_ _]
          frame False {
            n147 = Concatenate Strings("\\pulse_sequence_DAQ.ini" ("string")) -> (w334:string)
            n148 = Build Array(w334) -> (w333:string[])
          }
          frame True {
            n149 = call <vilib>:"Application Directory.vi"() -> ("Application Directory"=w338:path)
            n150 = Build Path(base path=w338, name or relative path=w337) -> (appended path=w339:path)
            n151 = List Folder(path=w339) -> (filenames=w336:string[])  [unwired: 3 in, 3 out]
          }
        }
        n152 = Concatenate Strings(w316, w319) -> (w318:string)
        n153 = Concatenate Strings(w316, "\\Zurich_params.ini" ("string")) -> (w328:string)
        n154 = Concatenate Strings(w316, "\\Keithley_params.ini" ("string")) -> (w329:string)
        n155 = for {
          tunnel: w332 -> [w401]
          tunnel: w329 -> [w397]
          tunnel: w328 -> [w396]
          shift-right: [w359] -> w323
          shift-left: w325 -> [w389]
          tunnel: w322 -> [w344] mode=indexing
          tunnel: w318 -> [w342]
          tunnel: w317 -> [w341]
          tunnel: w316 -> [w340]
          w363 = T13 {"R"=[], "Theta"=[], "X"=[], "Y"=[], "AuxIn0"=[], "AuxIn1"=[], "Frequency"=[], "DIO"=[], "Time"=[]} ("ZI Data")
          w386 = u16 58000 ("Fixed Number Of Points")
          n156 = property on="Rotation signal" class="XYGraph (strict)"("Visible"=TRUE) -> (error out=w355:errorcluster)  [unwired: 2 in, 1 out]
          n157 = property on="Rotation signal 3" class="XYGraph (strict)"("Visible"=FALSE) -> (error out=w356:errorcluster)  [unwired: 2 in, 1 out]
          n158 = invoke on="A" class="DigNum (strict)" method="Reinit To Default"() -> (error out=w351:errorcluster)  [unwired: 3 in, 2 out]
          n159 = invoke on="B" class="DigNum (strict)" method="Reinit To Default"() -> (error out=w350:errorcluster)  [unwired: 3 in, 2 out]
          n160 = invoke on="C" class="DigNum (strict)" method="Reinit To Default"() -> (error out=w349:errorcluster)  [unwired: 3 in, 2 out]
          n161 = invoke on="g1" class="DigNum (strict)" method="Reinit To Default"() -> (error out=w348:errorcluster)  [unwired: 3 in, 2 out]
          n162 = invoke on="g2" class="DigNum (strict)" method="Reinit To Default"() -> (error out=w352:errorcluster)  [unwired: 3 in, 2 out]
          n163 = invoke on="w" class="DigNum (strict)" method="Reinit To Default"() -> (error out=w353:errorcluster)  [unwired: 3 in, 2 out]
          n164 = invoke on="q" class="DigNum (strict)" method="Reinit To Default"() -> (error out=w354:errorcluster)  [unwired: 3 in, 2 out]
          n165 = case shown="False" w341 {
            tunnel: w344 -> [w404 w407]
            tunnel: [w402 w406] -> w343
            tunnel: w342 -> [_ w405]
            tunnel: w340 -> [w403 _]
            frame False {
              n166 = Concatenate Strings(w403, w404) -> (w402:string)
            }
            frame True {
              n167 = Concatenate Strings(w405, w407) -> (w406:string)
            }
          }
          n168 = Bundle By Name(cluster=T7 {"ZI config file (.ini)"="Config_Ver_2\\Zurich_params.ini", "Keithley config file (.ini)"="Config_Ver_2\\Keithley_params.ini", "DAQ config file (.ini)"="Config_Ver_2\\pulse_sequence_DAQ.ini"} ("Config files paths"), "ZI config file (.ini)"=w396, "Keithley config file (.ini)"=w397, "DAQ config file (.ini)"=w343) -> (w393:T7)
          n169 = Build Array(w363, w363) -> (w362:T13[])
          n170 = call "Initialize_Devices_Main_v2.vi"("error in"=w389, "Resource Address"=w401) -> ("error out"=w399:errorcluster, "Resources"=w400:T14)  [unwired: 8 in]
          n171 = Merge Errors(w351, w350, w349, w348, w352, w353, w354, w355, w356) -> (w345:errorcluster)
          n172 = Obtain Queue(name (unnamed)="Data Queue", element data type=w362, error in (no error)=w389) -> (queue out=w388:refnum<queue>, error out=w365:errorcluster)  [unwired: 2 in, 1 out]
          n173 = call "Configurate_All_Main_v2.vi"("Resources in"=w400, "Config files paths"=w393, "error in"=w399) -> ("Resources out"=w395:T14, "error out"=w394:errorcluster)  [unwired: 6 in, 5 out]
          n174 = for {
            N: "Number of repetition" -> [w460]
            tunnel: w393 -> [w465]
            shift-right: [w464] -> w392
            shift-left: w395 -> [w467]
            shift-right: [w452] -> w391
            shift-left: w394 -> [w466]
            tunnel: w388 -> [w455]
            i -> [w461]
            n175 = Divide(x=w461, y=w460) -> (x/y=w458:dbl)
            n176 = call "Single_Measurement_Main_v2.vi"("Config files paths"=w465, "error in"=w466, "Resources in"=w467) -> ("error out"=w462:errorcluster, "Resources out"=w463:T14)  [unwired: 6 in, 1 out]
            n177 = Multiply(x=w458, y=100.0) -> (x*y=→"Progress":dbl)
            n178 = call "Poll_Data_Main_v2.vi"("error in"=w462, "Resources in"=w463) -> ("error out"=w453:errorcluster, "ZI Data 3"=w454:T13, "ZI Data 0"=w451:T13, "Resources out"=w464:T14)  [unwired: 6 in]
            n179 = Build Array(w451, w454) -> (w456:T13[])
            n180 = Enqueue Element(queue=w455, element=w456, error in (no error)=w453) -> (error out=w452:errorcluster)  [unwired: 1 in, 2 out]
          }
          n181 = Initialize Array(0.0 ("element"), w386) -> (w384:dbl[])
          n182 = Merge Errors(w365, w345) -> (w364:errorcluster)
          n183 = for {
            N: "Number of repetition" -> [_]
            tunnel: w388 -> [w444]
            shift-right: [w441] -> w361
            shift-left: w364 -> [w446]
            tunnel: [w444] -> w387
            shift-right: [w434] -> w369
            shift-left: w384 -> [w437]
            tunnel: w386 -> [w440]
            shift-right: [w435] -> w370
            shift-left: w384 -> [w436]
            tunnel: [w423] -> w383
            tunnel: ["Signal in X or Y (?)"] -> w382
            n184 = Dequeue Element(queue=w444, timeout in ms (-1)=10000, error in (no error)=w446) -> (element=w445:T13[], error out=w442:errorcluster)  [unwired: 2 out]
            n185 = Index Array(array=w445) -> (element #1=w425:T13, element #2=w443:T13)  [unwired: 2 in]
            n186 = call "Clear_Data_Main_v2.vi"("ZI Data 0"=w425, "ZI Data 3"=w443, "Time Of Collected Data (ms)"=500.0, 3:"Fixed Number Of Points"=w440, "error in"=w442, 10:"Fixed Number Of Points"=TRUE ("Fixed Number Of Points"), "Check Phase Mismatch"=FALSE) -> ("Cutted Data 0"=w439:T17, "Cutted Data 3"=w438:T17, "error out"=w441:errorcluster)  [unwired: 7 in, 3 out]
            n187 = call "Prepare_plots_SubVI_v1.vi"("Signal in X or Y (?)"="Signal in X or Y (?)", "Y rot avg in"=w436, "X rot avg in"=w437, "Cutted Data 3"=w438, "Cutted Data 0"=w439) -> ("Y rot avg out"=w435:dbl[], "X rot avg out"=w434:dbl[], "Monitor"=→"Intensity signal":cluster{"Time":dbl[], dbl[]}, "RF out"=→"Differential signal":cluster{"Time":dbl[], "Y":dbl[]}[], "Rotation spectrum"=→"Rotation spectrum":waveform(dbl)[], "Rotation"=w430:cluster{"Time":dbl[], dbl[]}[], "Polarimeter"=→"Polarimeter":dbl)
            n188 = Index Array(array=w430) -> (element #1=w429:cluster{"Time":dbl[], dbl[]}, element #2=w428:cluster{"Time":dbl[], dbl[]})  [unwired: 2 in]
            n189 = Select(t=w429, s="Signal in X or Y (?)", f=w428) -> (s? t:f=w423:cluster{"Time":dbl[], dbl[]})
            "Rotation signal" <- w423
          }
          n190 = call "Close_Devices_Main_v2.vi"("error in"=w391, "Resources"=w392) -> ("error out"=w371:errorcluster)  [unwired: 9 in]
          n191 = flat-sequence {
            tunnel: w371 -> [_]
            frame #0 {
              n192 = local write "Progress"(100.0 ("Progress")) -> ()
            }
          }
          n193 = Merge Errors(w371, w361) -> (w360:errorcluster)
          n194 = Divide(x=w369, y="Number of repetition") -> (x/y=w367:dbl[])
          n195 = Divide(x=w370, y="Number of repetition") -> (x/y=w368:dbl[])
          n196 = Unbundle By Name(w383) -> ("Time"=w374:dbl[])
          n197 = Release Queue(queue=w387, error in (no error)=w360) -> (error out=w359:errorcluster)  [unwired: 1 in, 2 out]
          n198 = Build Array(w367, w368) -> (w375:dbl[][])
          n199 = Bundle("Time"=w374, w367) -> (w380:cluster{"Time":dbl[], dbl[]})  [unwired: 1 in]
          n200 = Bundle("Time"=w374, w368) -> (w381:cluster{"Time":dbl[], dbl[]})  [unwired: 1 in]
          n201 = Index Array(array=w374, index #1=1 ("index"), index #2=0 ("index")) -> (element #1=w378:dbl, element #2=w379:dbl)
          n202 = Select(t=w380, s=w382, f=w381) -> (s? t:f=w357:cluster{"Time":dbl[], dbl[]})
          n203 = Subtract(x=w378, y=w379) -> (x-y=w373:dbl)
          n204 = local write "Rotation signal"(w357) -> ()
          n205 = local read "save"() -> (w358:bool)
          n206 = for {
            tunnel: w375 -> [w422] mode=indexing
            tunnel: [w420] -> w372 mode=indexing
            tunnel: w373 -> [w417]
            n207 = call <vilib>:"Auto Power Spectrum.vi"("dt"=w417, "Signal (V)"=w422) -> ("df"=w421:dbl, "Power Spectrum (V^2 rms)"=w419:dbl[])
            n208 = Square Root(x=w419) -> (sqrt(x)=w418:dbl[])
            n209 = Bundle By Name("Y"=w418, "dt"=w421) -> (w420:waveform(dbl))  [unwired: 1 in]
          }
          n210 = case shown="True" w358 {
            tunnel: w357 -> [_ w416]
            frame False {
            }
            frame True {
              n211 = Unbundle(w416) -> ("Time"=w415:dbl[], w414:dbl[])
              n212 = Build Array(w415, w414) -> (w413:dbl[][])
              n213 = call <vilib>:"Create File with Incrementing Suffix.vi"("format string (\" (%d)\")"=" %d" ("format string (\" (%d)\")"), "file path"=path "C:/Users/Daniel/Desktop/tests/test.dat") -> ("actual path"=w410:path)  [unwired: 7 in, 2 out]
              n214 = Transpose 2D Array(2D array=w413) -> (transposed array=w412:dbl[][])
              n215 = call-poly <vilib>:"Write Delimited Spreadsheet.vi"("file path (dialog if empty)"=w410, "format (%.3f)"="%.6f", "2D data"=w412) -> ()  [unwired: 11 in, 2 out]
            }
          }
          n216 = local write "Rotation spectrum"(w372) -> ()
        }
        n217 = case shown="Error .." w323 {
          selector: w323 -> [w468 w469]
          tunnel: [w468 w472] -> w324
          frame No Error {
          }
          frame Error {
            w477 = "\r\n"
            n218 = Unbundle By Name(w469) -> ("code"=w480:i32, "source"=w478:string)
            n219 = Number To Decimal String(number=w480) -> (decimal integer string=w479:string)  [unwired: 1 in]
            n220 = Concatenate Strings("There is an error:" ("string"), w477, w479, w477, w478, w477, "Do you want to clear it?" ("string")) -> (w473:string)
            n221 = Two Button Dialog(message=w473, 1:"No" ("F button name (\"Cancel\")"), 2:"Yes" ("T button name (\"OK\")")) -> (T button?=w471:bool)
            n222 = call <vilib>:"Clear Errors.vi"("error in (no error)"=w469) -> ("error out"=w470:errorcluster)  [unwired: 5 in, 1 out]
            n223 = Select(t=w470, s=w471, f=w469) -> (s? t:f=w472:errorcluster)
          }
        }
      }
      event "Run tomography", "Run tomography 2": Mouse Down {
        w494 = T13 {"R"=[], "Theta"=[], "X"=[], "Y"=[], "AuxIn0"=[], "AuxIn1"=[], "Frequency"=[], "DIO"=[], "Time"=[]} ("ZI Data")
        w489 = "\\tomography" ("string")
        n224 = event-data() -> ()  [unwired: 1 in, 8 out]
        n225 = local read "Config folder"() -> (w490:string)
        n226 = local read "Resource Address"() -> (w519:T3)
        n227 = Build Array(w494, w494) -> (w493:T13[])
        n228 = flat-sequence {
          frame #0 {
            n229 = Wait (ms)(milliseconds to wait=u32 150) -> ()  [unwired: 1 out]
          }
          frame #1 {
            n230 = invoke on="Run tomography" class="Bool (strict)" method="Reinit To Default"() -> ()  [unwired: 3 in, 3 out]
            n231 = local write "Tab Control"(T10."Run tomography" ("Tab Control")) -> ()
          }
        }
        n232 = Concatenate Strings("Config_files\\" ("string"), w490, w489) -> (w492:string)
        n233 = Concatenate Strings(w490, w489, "\\" ("string")) -> (w488:string)
        n234 = call <vilib>:"Application Directory.vi"() -> ("Application Directory"=w522:path)
        n235 = Obtain Queue(name (unnamed)="Data Queue 2", element data type=w493, error in (no error)=w514) -> (queue out=w516:refnum<queue>, error out=w513:errorcluster)  [unwired: 2 in, 1 out]
        n236 = property on="Plot type" class="Ring (strict)"("DisabledEnum"=T9."Disabled and Grayed Out" ("Disabled")) -> (error out=w500:errorcluster)  [unwired: 2 in, 1 out]
        n237 = Concatenate Strings(w490, "\\Zurich_params.ini" ("string")) -> (w525:string)
        n238 = Concatenate Strings(w490, "\\Keithley_params.ini" ("string")) -> (w526:string)
        n239 = Build Path(base path=w522, name or relative path=w492) -> (appended path=w523:path)
        n240 = List Folder(path=w523) -> (filenames=w521:string[])  [unwired: 3 in, 3 out]
        n241 = call "Initialize_Devices_Main_v2.vi"("error in"=w513, "Resource Address"=w519) -> ("error out"=w517:errorcluster, "Resources"=w518:T14)  [unwired: 8 in]
        n242 = for {
          tunnel: "pulses type (priv)" -> [w532] mode=indexing
          tunnel: [w530] -> w503 mode=concatenating
          n243 = for {
            tunnel: " + " ("string") -> [w537]
            tunnel: w532 -> [w536]
            tunnel: string[] ["[ None ]", "[ Y pi ]", "[ Z(pi/2)+Y(pi) ]"] -> [w535] mode=indexing
            tunnel: [w534] -> w530 mode=indexing
            n244 = Concatenate Strings(w536, w537, w535) -> (w534:string)
          }
        }
        n245 = for {
          N -> [w566]
          tunnel: w526 -> [w574]
          tunnel: w525 -> [w573]
          tunnel: w521 -> [w538] mode=indexing
          shift-right: [w569] -> w486
          shift-left: w517 -> [w544]
          tunnel: w516 -> [w570]
          shift-right: [w571] -> w512
          shift-left: w518 -> [w543]
          tunnel: u16 58000 ("Fixed Number Of Points") -> [w567]
          tunnel: [w568] -> w510
          shift-right: [w562] -> w507
          shift-left: dbl[][] [] -> [w563]
          tunnel: w503 -> [_]
          tunnel: [w559] -> w502 mode=indexing
          tunnel: w500 -> [_]
          tunnel: w488 -> [w540]
          i -> [w560]
          n246 = Concatenate Strings(w540, w538) -> (w539:string)
          n247 = Multiply(x="Averaging", y=w560) -> (x*y=w565:i32)
          n248 = Bundle By Name(cluster=T7 {"ZI config file (.ini)"="Config_Ver_2\\Zurich_params.ini", "Keithley config file (.ini)"="Config_Ver_2\\Keithley_params.ini", "DAQ config file (.ini)"="Config_Ver_2\\pulse_sequence_DAQ.ini"} ("Config files paths"), "ZI config file (.ini)"=w573, "Keithley config file (.ini)"=w574, "DAQ config file (.ini)"=w539) -> (w541:T7)
          n249 = call "Configurate_All_Main_v2.vi"("Resources in"=w543, "Config files paths"=w541, "error in"=w544) -> ("Resources out"=w542:T14, "error out"=w545:errorcluster)  [unwired: 6 in, 5 out]
          n250 = for {
            N: "Averaging" -> [w623]
            shift-right: [w635] -> w571
            shift-left: w542 -> [w637]
            shift-right: [w626] -> w557
            shift-left: w545 -> [w636]
            tunnel: w570 -> [w628]
            tunnel: w541 -> [w625]
            tunnel: w566 -> [w624]
            tunnel: w565 -> [w620]
            i -> [w621]
            n251 = Add(x=w621, y=w620) -> (x+y=w619:i32)
            n252 = Multiply(x=w623, y=w624) -> (x*y=w622:i32)
            n253 = call "Single_Measurement_Main_v2.vi"("Config files paths"=w625, "error in"=w636, "Resources in"=w637) -> ("error out"=w633:errorcluster, "Resources out"=w634:T14)  [unwired: 6 in, 1 out]
            n254 = call "Poll_Data_Main_v2.vi"("error in"=w633, "Resources in"=w634) -> ("error out"=w627:errorcluster, "ZI Data 3"=w630:T13, "ZI Data 0"=w617:T13, "Resources out"=w635:T14)  [unwired: 6 in]
            n255 = Divide(x=w619, y=w622) -> (x/y=w631:dbl)
            n256 = Build Array(w617, w630) -> (w629:T13[])
            n257 = Multiply(x=w631, y=100.0) -> (x*y=→"Progress":dbl)
            n258 = Enqueue Element(queue=w628, element=w629, error in (no error)=w627) -> (error out=w626:errorcluster)  [unwired: 1 in, 2 out]
          }
          n259 = Initialize Array(0.0 ("element"), w567) -> (w554:dbl[])
          n260 = for {
            N: "Averaging" -> [_]
            shift-right: [w608] -> w558
            shift-left: w544 -> [w613]
            shift-right: [w602] -> w552
            shift-left: w554 -> [w605]
            shift-right: [w603] -> w553
            shift-left: w554 -> [w604]
            tunnel: [w595] -> w548
            tunnel: w570 -> [w594]
            tunnel: w567 -> [w593]
            tunnel: [w592] -> w550
            n261 = local read "Signal in X or Y (?)"() -> (w595:bool)
            n262 = Dequeue Element(queue=w594, timeout in ms (-1)=10000, error in (no error)=w613) -> (element=w612:T13[], error out=w609:errorcluster)  [unwired: 2 out]
            n263 = Index Array(array=w612) -> (element #1=w610:T13, element #2=w611:T13)  [unwired: 2 in]
            n264 = call "Clear_Data_Main_v2.vi"("ZI Data 0"=w610, "ZI Data 3"=w611, "Time Of Collected Data (ms)"=500.0, 3:"Fixed Number Of Points"=w593, "error in"=w609, 10:"Fixed Number Of Points"=TRUE ("Fixed Number Of Points"), "Check Phase Mismatch"=FALSE) -> ("Cutted Data 0"=w607:T17, "Cutted Data 3"=w606:T17, "error out"=w608:errorcluster)  [unwired: 7 in, 3 out]
            n265 = call "Prepare_plots_SubVI_v1.vi"("Signal in X or Y (?)"=w595, "Y rot avg in"=w604, "X rot avg in"=w605, "Cutted Data 3"=w606, "Cutted Data 0"=w607) -> ("Y rot avg out"=w603:dbl[], "X rot avg out"=w602:dbl[], "Monitor"=→"Intensity signal":cluster{"Time":dbl[], dbl[]}, "RF out"=→"Differential signal":cluster{"Time":dbl[], "Y":dbl[]}[], "Rotation spectrum"=→"Rotation spectrum":waveform(dbl)[], "Rotation"=w599:cluster{"Time":dbl[], dbl[]}[])  [unwired: 1 out]
            n266 = Index Array(array=w599) -> (element #1=w598:cluster{"Time":dbl[], dbl[]}, element #2=w597:cluster{"Time":dbl[], dbl[]})  [unwired: 2 in]
            n267 = Select(t=w598, s=w595, f=w597) -> (s? t:f=w592:cluster{"Time":dbl[], dbl[]})
            "Rotation signal" <- w592
          }
          n268 = Divide(x=w552, y="Averaging") -> (x/y=w546:dbl[])
          n269 = Divide(x=w553, y="Averaging") -> (x/y=w547:dbl[])
          n270 = Empty Array?(array=w563) -> (empty?=w551:bool)
          n271 = Unbundle By Name(w550) -> ("Time"=w549:dbl[])
          n272 = Merge Errors(w557, w558) -> (w556:errorcluster)
          n273 = case shown="True" w551 {
            tunnel: w549 -> [w576 w583]
            tunnel: w563 -> [w582 w590]
            tunnel: [w581 w589] -> w562
            tunnel: w548 -> [w580 w588]
            tunnel: w547 -> [w579 w587]
            tunnel: w546 -> [w578 w586]
            tunnel: [w575 w585] -> w561
            frame True {
              n274 = Select(t=w578, s=w580, f=w579) -> (s? t:f=w577:dbl[])
              n275 = Bundle("Time"=w576, w577) -> (w575:cluster{"Time":dbl[], dbl[]})  [unwired: 1 in]
              n276 = Build Array (concatenate)(w582, w576, w577) -> (w581:dbl[][])
            }
            frame False {
              n277 = Select(t=w586, s=w588, f=w587) -> (s? t:f=w584:dbl[])
              n278 = Bundle("Time"=w583, w584) -> (w585:cluster{"Time":dbl[], dbl[]})  [unwired: 1 in]
              n279 = Build Array (concatenate)(w590, w584) -> (w589:dbl[][])
            }
          }
          n280 = Flush Queue(queue=w570, error in (no error)=w556) -> (queue out=w568:refnum<queue>, error out=w569:errorcluster)  [unwired: 1 out]
          n281 = flat-sequence {
            tunnel: w561 -> [w638]
            tunnel: w560 -> [w639]
            tunnel: [w638] -> w559
            frame #0 {
              n282 = local write "Plot type"(w639) -> ()
              "Rotation" <- w638
            }
          }
        }
        "tomography rotation memory (priv)" <- w502
        n283 = property on="Plot type" class="Ring (strict)"("Strings []"=w503) -> ()  [unwired: 2 in, 2 out]
        n284 = Release Queue(queue=w510, error in (no error)=w486) -> (error out=w509:errorcluster)  [unwired: 1 in, 2 out]
        n285 = flat-sequence {
          tunnel: w486 -> [_]
          frame #0 {
            n286 = local write "Progress"(100.0 ("Progress")) -> ()
          }
        }
        n287 = call "Close_Devices_Main_v2.vi"("error in"=w509, "Resources"=w512) -> ("error out"=w498:errorcluster)  [unwired: 9 in]
        n288 = property on="Plot type" class="Ring (strict)"(error in=w486, "DisabledEnum"=T9."Enabled" ("Disabled")) -> (error out=w497:errorcluster)  [unwired: 1 in, 1 out]
        n289 = call "Save_Tomography_Data_Main_v2.vi"("error in"=w486, "Save CYCLOPS data (?)"="Save CYCLOPS data (?)", "Save raw data (?)"="Save raw data (?)", "Data Raw"=w507) -> ("error out"=w496:errorcluster)  [unwired: 6 in, 1 out]
        n290 = Merge Errors(w498, w497, w496) -> (w495:errorcluster)
        n291 = case shown="Error .." w495 {
          selector: w495 -> [w640 w641]
          tunnel: [w640 w644] -> w524
          frame No Error {
          }
          frame Error {
            w649 = "\r\n"
            n292 = Unbundle By Name(w641) -> ("code"=w652:i32, "source"=w650:string)
            n293 = Number To Decimal String(number=w652) -> (decimal integer string=w651:string)  [unwired: 1 in]
            n294 = Concatenate Strings("There is an error:" ("string"), w649, w651, w649, w650, w649, "Do you want to clear it?" ("string")) -> (w645:string)
            n295 = Two Button Dialog(message=w645, 1:"No" ("F button name (\"Cancel\")"), 2:"Yes" ("T button name (\"OK\")")) -> (T button?=w643:bool)
            n296 = call <vilib>:"Clear Errors.vi"("error in (no error)"=w641) -> ("error out"=w642:errorcluster)  [unwired: 5 in, 1 out]
            n297 = Select(t=w642, s=w643, f=w641) -> (s? t:f=w644:errorcluster)
          }
        }
      }
      event "Run QPT", "Run QPT 2": Mouse Down {
        w665 = "\\process\\temp_states" ("string")
        # "9 FIDs compose 1 Tomography"
        n298 = event-data() -> ()  [unwired: 1 in, 8 out]
        n299 = local read "Config folder"() -> (w666:string)
        n300 = local read "Resource Address"() -> (w658:T3)
        n301 = flat-sequence {
          frame #0 {
            n302 = Wait (ms)(milliseconds to wait=u32 150) -> ()  [unwired: 1 out]
          }
          frame #1 {
            n303 = invoke on="Run tomography" class="Bool (strict)" method="Reinit To Default"() -> ()  [unwired: 3 in, 3 out]
            n304 = local write "Tab Control"(T1."Run QPT" ("Tab Control")) -> ()
          }
        }
        n305 = Concatenate Strings("Config_files\\" ("string"), w666, w665) -> (w668:string)
        n306 = Concatenate Strings(w666, w665, "\\" ("string")) -> (w664:string)
        n307 = call <vilib>:"Application Directory.vi"() -> ("Application Directory"=w676:path)
        n308 = property on="Plot type" class="Ring (strict)"("DisabledEnum"=T9."Disabled and Grayed Out" ("Disabled")) -> (error out=w662:errorcluster)  [unwired: 2 in, 1 out]
        n309 = Concatenate Strings(w666, "\\Zurich_params.ini" ("string")) -> (w679:string)
        n310 = Concatenate Strings(w666, "\\Keithley_params.ini" ("string")) -> (w680:string)
        n311 = Build Path(base path=w676, name or relative path=w668) -> (appended path=w677:path)
        n312 = List Folder(path=w677) -> (filenames=w661:string[])  [unwired: 3 in, 3 out]
        n313 = call "Splitting_filename.vi"("Splitting number"=u32 9, "Total filenames"=w661) -> ("Splitted filenames"=w660:string[][])  [unwired: 9 in]
        n314 = for {
          N -> [w707]
          tunnel: w680 -> [w718]
          tunnel: w679 -> [w717]
          tunnel: "Save CYCLOPS data (?) 2" -> [w687]
          tunnel: "Save raw data (?) 2" -> [w688]
          tunnel: w664 -> [w714]
          tunnel: w660 -> [w713] mode=indexing
          shift-right: [w715] -> w671
          shift-left: _ -> [_]
          shift-right: [w685] -> w670
          shift-left: w662 -> [w712]
          tunnel: w658 -> [w703]
          tunnel: w657 -> [w700]
          tunnel: [w692] -> w656
          i -> [w690]
          w697 = T13 {"R"=[], "Theta"=[], "X"=[], "Y"=[], "AuxIn0"=[], "AuxIn1"=[], "Frequency"=[], "DIO"=[], "Time"=[]} ("ZI Data")
          n315 = Increment(x=w690) -> (x+1=→"Current_QPT_order":i32)
          n316 = Build Array(w697, w697) -> (w696:T13[])
          n317 = Divide(x=w690, y=w707) -> (x/y=w706:dbl)
          n318 = Multiply(x=100.0, y=w706) -> (x*y=→"QPT Progress":dbl)
          n319 = Obtain Queue(name (unnamed)="Data Queue 2", element data type=w696, error in (no error)=w700) -> (queue out=w699:refnum<queue>, error out=w698:errorcluster)  [unwired: 2 in, 1 out]
          n320 = call "Initialize_Devices_Main_v2.vi"("error in"=w698, "Resource Address"=w703) -> ("error out"=w702:errorcluster, "Resources"=w701:T14)  [unwired: 8 in]
          n321 = for {
            N -> [w749]
            tunnel: w718 -> [w756]
            tunnel: w717 -> [w755]
            tunnel: w713 -> [w721] mode=indexing
            shift-right: [w752] -> w686
            shift-left: w702 -> [w727]
            shift-right: [w753] -> w693
            shift-left: w701 -> [w726]
            tunnel: u16 58000 ("Fixed Number Of Points") -> [w750]
            tunnel: [w751] -> w711
            shift-right: [w745] -> w689
            shift-left: dbl[][] [] -> [w746]
            tunnel: [w742] -> w708 mode=indexing
            tunnel: w714 -> [w723]
            tunnel: w712 -> [_]
            tunnel: w699 -> [w720]
            i -> [w743]
            n322 = Concatenate Strings(w723, w721) -> (w722:string)
            n323 = Multiply(x="Averaging 2", y=w743) -> (x*y=w748:i32)
            n324 = Bundle By Name(cluster=T7 {"ZI config file (.ini)"="Config_Ver_2\\Zurich_params.ini", "Keithley config file (.ini)"="Config_Ver_2\\Keithley_params.ini", "DAQ config file (.ini)"="Config_Ver_2\\pulse_sequence_DAQ.ini"} ("Config files paths"), "ZI config file (.ini)"=w755, "Keithley config file (.ini)"=w756, "DAQ config file (.ini)"=w722) -> (w724:T7)
            n325 = call "Configurate_All_Main_v2.vi"("Resources in"=w726, "Config files paths"=w724, "error in"=w727) -> ("Resources out"=w725:T14, "error out"=w728:errorcluster)  [unwired: 6 in, 5 out]
            n326 = for {
              N: "Averaging 2" -> [w805]
              shift-right: [w817] -> w753
              shift-left: w725 -> [w819]
              shift-right: [w808] -> w740
              shift-left: w728 -> [w818]
              tunnel: w720 -> [w810]
              tunnel: w724 -> [w807]
              tunnel: w749 -> [w806]
              tunnel: w748 -> [w802]
              i -> [w803]
              n327 = Add(x=w803, y=w802) -> (x+y=w801:i32)
              n328 = Multiply(x=w805, y=w806) -> (x*y=w804:i32)
              n329 = call "Single_Measurement_Main_v2.vi"("Config files paths"=w807, "error in"=w818, "Resources in"=w819) -> ("error out"=w815:errorcluster, "Resources out"=w816:T14)  [unwired: 6 in, 1 out]
              n330 = call "Poll_Data_Main_v2.vi"("error in"=w815, "Resources in"=w816) -> ("error out"=w809:errorcluster, "ZI Data 3"=w812:T13, "ZI Data 0"=w799:T13, "Resources out"=w817:T14)  [unwired: 6 in]
              n331 = Divide(x=w801, y=w804) -> (x/y=w813:dbl)
              n332 = Build Array(w799, w812) -> (w811:T13[])
              n333 = Multiply(x=w813, y=100.0) -> (x*y=→"Single Tomography Progress":dbl)
              n334 = Enqueue Element(queue=w810, element=w811, error in (no error)=w809) -> (error out=w808:errorcluster)  [unwired: 1 in, 2 out]
            }
            n335 = Initialize Array(0.0 ("element"), w750) -> (w737:dbl[])
            n336 = for {
              N: "Averaging 2" -> [_]
              shift-right: [w790] -> w741
              shift-left: w727 -> [w795]
              shift-right: [w784] -> w735
              shift-left: w737 -> [w787]
              shift-right: [w785] -> w736
              shift-left: w737 -> [w786]
              tunnel: [w777] -> w731
              tunnel: w720 -> [w776]
              tunnel: w750 -> [w775]
              tunnel: [w774] -> w733
              n337 = local read "Signal in X or Y (?)"() -> (w777:bool)
              n338 = Dequeue Element(queue=w776, timeout in ms (-1)=10000, error in (no error)=w795) -> (element=w794:T13[], error out=w791:errorcluster)  [unwired: 2 out]
              n339 = Index Array(array=w794) -> (element #1=w792:T13, element #2=w793:T13)  [unwired: 2 in]
              n340 = call "Clear_Data_Main_v2.vi"("ZI Data 0"=w792, "ZI Data 3"=w793, "Time Of Collected Data (ms)"=500.0, 3:"Fixed Number Of Points"=w775, "error in"=w791, 10:"Fixed Number Of Points"=TRUE ("Fixed Number Of Points"), "Check Phase Mismatch"=FALSE) -> ("Cutted Data 0"=w789:T17, "Cutted Data 3"=w788:T17, "error out"=w790:errorcluster)  [unwired: 7 in, 3 out]
              n341 = call "Prepare_plots_SubVI_v1.vi"("Signal in X or Y (?)"=w777, "Y rot avg in"=w786, "X rot avg in"=w787, "Cutted Data 3"=w788, "Cutted Data 0"=w789) -> ("Y rot avg out"=w785:dbl[], "X rot avg out"=w784:dbl[], "Monitor"=→"Intensity signal 2":cluster{"Time":dbl[], dbl[]}, "RF out"=→"Differential signal 2":cluster{"Time":dbl[], "Y":dbl[]}[], "Rotation spectrum"=→"Rotation spectrum 2":waveform(dbl)[], "Rotation"=w781:cluster{"Time":dbl[], dbl[]}[])  [unwired: 1 out]
              n342 = Index Array(array=w781) -> (element #1=w780:cluster{"Time":dbl[], dbl[]}, element #2=w779:cluster{"Time":dbl[], dbl[]})  [unwired: 2 in]
              n343 = Select(t=w780, s=w777, f=w779) -> (s? t:f=w774:cluster{"Time":dbl[], dbl[]})
              "Rotation signal 2" <- w774
            }
            n344 = Divide(x=w735, y="Averaging 2") -> (x/y=w729:dbl[])
            n345 = Divide(x=w736, y="Averaging 2") -> (x/y=w730:dbl[])
            n346 = Empty Array?(array=w746) -> (empty?=w734:bool)
            n347 = Unbundle By Name(w733) -> ("Time"=w732:dbl[])
            n348 = Merge Errors(w740, w741) -> (w739:errorcluster)
            n349 = case shown="True" w734 {
              tunnel: w732 -> [w758 w765]
              tunnel: w746 -> [w764 w772]
              tunnel: [w763 w771] -> w745
              tunnel: w731 -> [w762 w770]
              tunnel: w730 -> [w761 w769]
              tunnel: w729 -> [w760 w768]
              tunnel: [w757 w767] -> w744
              frame True {
                n350 = Select(t=w760, s=w762, f=w761) -> (s? t:f=w759:dbl[])
                n351 = Bundle("Time"=w758, w759) -> (w757:cluster{"Time":dbl[], dbl[]})  [unwired: 1 in]
                n352 = Build Array (concatenate)(w764, w758, w759) -> (w763:dbl[][])
              }
              frame False {
                n353 = Select(t=w768, s=w770, f=w769) -> (s? t:f=w766:dbl[])
                n354 = Bundle("Time"=w765, w766) -> (w767:cluster{"Time":dbl[], dbl[]})  [unwired: 1 in]
                n355 = Build Array (concatenate)(w772, w766) -> (w771:dbl[][])
              }
            }
            n356 = Flush Queue(queue=w720, error in (no error)=w739) -> (queue out=w751:refnum<queue>, error out=w752:errorcluster)  [unwired: 1 out]
            n357 = flat-sequence {
              tunnel: w744 -> [w820]
              tunnel: w743 -> [w821]
              tunnel: [w820] -> w742
              frame #0 {
                n358 = local write "Plot type"(w821) -> ()
                "Rotation 2" <- w820
              }
            }
          }
          "tomography rotation memory (priv) 2" <- w708
          n359 = local read "Current_QPT_order"() -> (w684:i32)
          n360 = Release Queue(queue=w711, error in (no error)=w686) -> (error out=w694:errorcluster)  [unwired: 1 in, 2 out]
          n361 = flat-sequence {
            tunnel: w686 -> [_]
            frame #0 {
              n362 = local write "Single Tomography Progress"(100.0 ("Progress")) -> ()
            }
          }
          n363 = property on="Plot type" class="Ring (strict)"(error in=w686, "DisabledEnum"=T9."Enabled" ("Disabled")) -> (error out=w715:errorcluster)  [unwired: 1 in, 1 out]
          n364 = call "Save_QPT_Data_Main_v2.vi"("Numeric"=w684, "error in"=w686, "Save CYCLOPS data (?)"=w687, "Save raw data (?)"=w688, "Data Raw"=w689) -> ("error out"=w685:errorcluster)  [unwired: 5 in, 1 out]
          n365 = call "Close_Devices_Main_v2.vi"("error in"=w694, "Resources"=w693) -> ("error out"=w692:errorcluster)  [unwired: 9 in]
        }
        n366 = flat-sequence {
          tunnel: w656 -> [_]
          frame #0 {
            n367 = local write "QPT Progress"(100.0 ("x")) -> ()
          }
        }
        n368 = Merge Errors(w656, w671, w670) -> (w669:errorcluster)
        n369 = case shown="Error .." w669 {
          selector: w669 -> [w822 w823]
          tunnel: [w822 w826] -> w678
          frame No Error {
          }
          frame Error {
            w831 = "\r\n"
            n370 = Unbundle By Name(w823) -> ("code"=w834:i32, "source"=w832:string)
            n371 = Number To Decimal String(number=w834) -> (decimal integer string=w833:string)  [unwired: 1 in]
            n372 = Concatenate Strings("There is an error:" ("string"), w831, w833, w831, w832, w831, "Do you want to clear it?" ("string")) -> (w827:string)
            n373 = Two Button Dialog(message=w827, 1:"No" ("F button name (\"Cancel\")"), 2:"Yes" ("T button name (\"OK\")")) -> (T button?=w825:bool)
            n374 = call <vilib>:"Clear Errors.vi"("error in (no error)"=w823) -> ("error out"=w824:errorcluster)  [unwired: 5 in, 1 out]
            n375 = Select(t=w824, s=w825, f=w823) -> (s? t:f=w826:errorcluster)
          }
        }
      }
      event "Plot type": Value Change {
        n376 = event-data() -> ()  [unwired: 1 in, 6 out]
        n377 = local read "tomography rotation memory (priv)"() -> (w840:cluster{"Time":dbl[], dbl[]}[])
        n378 = local read "Plot type"() -> (w841:u16)
        n379 = Index Array(array=w840, index=w841) -> (element=w842:cluster{"Time":dbl[], dbl[]})
        n380 = local write "Rotation"(w842) -> ()
      }
      event "Fit model": Mouse Down {
        w848 = 2.0 ("x")
        w866 = 5 ("y")
        w873 = 1 ("index")
        # "q"
        # "w"
        # "g"
        # "C"
        # "B"
        # "A"
        # "initial values:"
        n381 = event-data() -> ()  [unwired: 1 in, 8 out]
        n382 = local read "Rotation signal"() -> (w867:cluster{"Time":dbl[], dbl[]})
        n383 = Decrement(x=w873) -> (x-1=w875:i32)
        n384 = Unbundle(w867) -> ("Time"=w874:dbl[], w871:dbl[])
        n385 = property on="Rotation signal" class="XYGraph (strict)"(error in=w881, "Visible"=FALSE) -> (error out=w879:errorcluster)  [unwired: 1 in, 1 out]
        n386 = property on="Rotation signal 3" class="XYGraph (strict)"(error in=w881, "Visible"=TRUE) -> (error out=w880:errorcluster)  [unwired: 1 in, 1 out]
        n387 = local read "Polarimeter"() -> (w856:dbl)
        n388 = Array Size(array=w871) -> (size(s)=w872:i32)
        n389 = Index Array(array=w874, index #1=w873, index #2=w875) -> (element #1=w876:dbl, element #2=w877:dbl)
        n390 = Multiply(x=1100.0, y=6.283185307179586) -> (x*y=w852:dbl)
        n391 = Subtract(x=w876, y=w877) -> (x-y=w865:dbl)
        n392 = Quotient & Remainder(x=w872, y=w866) -> (floor(x/y)=w870:i32)  [unwired: 1 out]
        n393 = Merge Errors(w879, w880) -> (w878:errorcluster)
        n394 = Reshape Array(w871, w870, w866) -> (w869:dbl[][])
        n395 = Multiply(x=w865, y=w866) -> (x*y=w863:dbl)
        n396 = Index Array(array=w869, index (col)=0 ("disabled index (col)")) -> (element=w845:dbl[])  [unwired: 1 in]
        n397 = Array Subset(array=w845, index=0, length=100) -> (w859:dbl[])
        n398 = Array Max & Min(array=w859) -> (max value=w858:dbl, min value=w857:dbl)  [unwired: 2 out]
        n399 = Subtract(x=w858, y=w857) -> (x-y=w849:dbl)
        n400 = Add(x=w858, y=w857) -> (x+y=w850:dbl)
        n401 = Divide(x=w850, y=w848) -> (x/y=w847:dbl)
        n402 = Divide(x=w849, y=w848) -> (x/y=w846:dbl)
        n403 = Array Size(array=w845) -> (size(s)=w864:i32)
        n404 = for {
          N: w864 -> [_]
          tunnel: w863 -> [w889]
          tunnel: [w888] -> w862 mode=indexing
          i -> [w890]
          n405 = Multiply(x=w889, y=w890) -> (x*y=w888:dbl)
        }
        n406 = Multiply(x=w845, y=1000) -> (x*y=w843:dbl[])
        n407 = case shown="\"Full\"" "Enum" {
          tunnel: [w922 w948 w975] -> w884
          tunnel: [w911 w938 w967] -> w882
          tunnel: w878 -> [w911 w938 w967]
          tunnel: w867 -> [w921 w947 w974]
          tunnel: w862 -> [w914 w941 w970]
          tunnel: w847 -> [w920 _ w953]
          tunnel: w856 -> [w919 w946 w952]
          tunnel: 20.0 -> [w918 w945 w951]
          tunnel: w852 -> [_ w932 w950]
          tunnel: 0.0 -> [_ w933 w949]
          tunnel: w846 -> [_ w934 w954]
          tunnel: w843 -> [w915 w942 w971]
          frame "B*Exp(-q2*t)+C" {
            w923 = nan
            n408 = Build Array(w920, w919, w918) -> (w912:dbl[])
            n409 = call-poly <vilib>:"Nonlinear Curve Fit.vi"("Y"=w915, "initial parameters"=w912, "X"=w914, "model description"=T11 {"model"="b*exp(-g2*t)+c", "Parameters"=["b", "c", "g2"], "x"="t"}, "error in (no error)"=w911) -> ("best nonlinear fit"=w913:dbl[], "best fit parameters"=w909:dbl[])  [unwired: 6 in, 3 out]
            n410 = Divide(x=w913, y=1000) -> (x/y=w917:dbl[])
            n411 = Index Array(array=w909) -> (element #1=w908:dbl, element #2=w907:dbl, element #3=w906:dbl)  [unwired: 3 in]
            n412 = Bundle(w914, w917) -> (w905:cluster{dbl[], dbl[]})  [unwired: 1 in]
            n413 = Build Array(w921, w905) -> (w922:cluster{"Time":dbl[], dbl[]}[])
            n414 = local write "A"(w923) -> ()
            n415 = local write "C"(w907) -> ()
            n416 = local write "g2"(w906) -> ()
            n417 = local write "q"(w923) -> ()
            n418 = local write "w"(w923) -> ()
            n419 = local write "g1"(w923) -> ()
            n420 = local write "B"(w908) -> ()
          }
          frame "A*Sin(w*t+q)*Exp(-g1*t)+C" {
            w931 = nan
            n421 = Build Array(w934, w946, w945, w933, w932) -> (w939:dbl[])
            n422 = call-poly <vilib>:"Nonlinear Curve Fit.vi"("Y"=w942, "initial parameters"=w939, "X"=w941, "model description"=T11 {"model"="a*sin(w*t+q)*exp(-g1*t)+c", "Parameters"=["a", "c", "g1", "q", "w"], "x"="t"}, "error in (no error)"=w938) -> ("best nonlinear fit"=w940:dbl[], "best fit parameters"=w936:dbl[])  [unwired: 6 in, 3 out]
            n423 = Divide(x=w940, y=1000) -> (x/y=w944:dbl[])
            n424 = Index Array(array=w936) -> (element #1=w930:dbl, element #2=w929:dbl, element #3=w928:dbl, element #4=w926:dbl, element #5=w927:dbl)  [unwired: 5 in]
            n425 = Bundle(w941, w944) -> (w935:cluster{dbl[], dbl[]})  [unwired: 1 in]
            n426 = Quotient & Remainder(x=w926, y=6.283185307179586) -> (x-y*floor(x/y)=w924:dbl)  [unwired: 1 out]
            n427 = Build Array(w947, w935) -> (w948:cluster{"Time":dbl[], dbl[]}[])
            n428 = local write "g1"(w928) -> ()
            n429 = local write "w"(w927) -> ()
            n430 = local write "A"(w930) -> ()
            n431 = local write "C"(w929) -> ()
            n432 = local write "q"(w924) -> ()
            n433 = local write "B"(w931) -> ()
            n434 = local write "g2"(w931) -> ()
          }
          frame "Full" {
            n435 = Build Array(w954, w953, w952, w951, w951, w950, w949) -> (w968:dbl[])
            n436 = call-poly <vilib>:"Nonlinear Curve Fit.vi"("Y"=w971, "initial parameters"=w968, "X"=w970, "model description"=T11 {"model"="a*sin(w*t+q)*exp(-g1*t)+b*exp(-g2*t)+c", "Parameters"=["a", "b", "c", "g1", "g2", "w", "q"], "x"="t"}, "error in (no error)"=w967) -> ("best nonlinear fit"=w969:dbl[], "best fit parameters"=w958:dbl[])  [unwired: 6 in, 3 out]
            n437 = Divide(x=w969, y=1000) -> (x/y=w973:dbl[])
            n438 = Index Array(array=w958) -> (element #1=w964:dbl, element #2=w960:dbl, element #3=w961:dbl, element #4=w962:dbl, element #5=w963:dbl, element #6=w959:dbl, element #7=w955:dbl)  [unwired: 7 in]
            n439 = Bundle(w970, w973) -> (w965:cluster{dbl[], dbl[]})  [unwired: 1 in]
            n440 = local write "w"(w959) -> ()
            n441 = local write "A"(w964) -> ()
            n442 = local write "B"(w960) -> ()
            n443 = local write "C"(w961) -> ()
            n444 = local write "g1"(w962) -> ()
            n445 = local write "g2"(w963) -> ()
            n446 = Quotient & Remainder(x=w955, y=6.283185307179586) -> (x-y*floor(x/y)=w956:dbl)  [unwired: 1 out]
            n447 = Build Array(w974, w965) -> (w975:cluster{"Time":dbl[], dbl[]}[])
            n448 = local write "q"(w956) -> ()
          }
        }
        n449 = Reverse 1D Array(array=w884) -> (reversed array=→"Rotation signal 3":cluster{"Time":dbl[], dbl[]}[])
        n450 = case shown="Error .." w882 {
          selector: w882 -> [w891 w892]
          tunnel: [w891 w895] -> _
          frame No Error {
          }
          frame Error {
            w900 = "\r\n"
            n451 = Unbundle By Name(w892) -> ("code"=w903:i32, "source"=w901:string)
            n452 = Number To Decimal String(number=w903) -> (decimal integer string=w902:string)  [unwired: 1 in]
            n453 = Concatenate Strings("There is an error:" ("string"), w900, w902, w900, w901, w900, "Do you want to clear it?" ("string")) -> (w896:string)
            n454 = Two Button Dialog(message=w896, 1:"No" ("F button name (\"Cancel\")"), 2:"Yes" ("T button name (\"OK\")")) -> (T button?=w894:bool)
            n455 = call <vilib>:"Clear Errors.vi"("error in (no error)"=w892) -> ("error out"=w893:errorcluster)  [unwired: 5 in, 1 out]
            n456 = Select(t=w893, s=w894, f=w892) -> (s? t:f=w895:errorcluster)
          }
        }
      }
      event "AOC": Mouse Down {
        n457 = event-data() -> ()  [unwired: 1 in, 8 out]
        n458 = Look In Map(map=w985, key="pulse Y") -> (value=w1000:i32)  [unwired: 1 in, 1 out]
        n459 = Look In Map(map=w983, key="Y pi/2") -> (value=w998:dbl)  [unwired: 1 in, 1 out]
        n460 = Look In Map(map=w983, key="Delay") -> (value=w997:dbl)  [unwired: 1 in, 1 out]
        n461 = Look In Map(map=w985, key="pulse Z") -> (value=w994:i32)  [unwired: 1 in, 1 out]
        n462 = Look In Map(map=w983, key="Z pi/4") -> (value=w991:dbl)  [unwired: 1 in, 1 out]
        n463 = Look In Map(map=w983, key="Delay") -> (value=w992:dbl)  [unwired: 1 in, 1 out]
        n464 = call "Add_to_sequence_SubVI_v1.vi"("Delay [us]"=w997, "Pulse length [us]"=w998, "Channel number"=w1000, "Array sequence in"=w1001) -> ("Array sequence out"=w996:cluster{"Timing 0":dbl[]}[])
        n465 = call "Add_to_sequence_SubVI_v1.vi"("Delay [us]"=w992, "Pulse length [us]"=w991, "Channel number"=w994, "Array sequence in"=w996) -> ("Array sequence out"=w986:cluster{"Timing 0":dbl[]}[])
        n466 = Wait (ms)(milliseconds to wait=u32 150) -> ()  [unwired: 1 out]
        n467 = Look In Map(map=w985, key="pulse Y") -> (value=w981:i32)  [unwired: 1 in, 1 out]
        n468 = Look In Map(map=w983, key="Y pi/2") -> (value=w980:dbl)  [unwired: 1 in, 1 out]
        n469 = Look In Map(map=w983, key="Delay") -> (value=w979:dbl)  [unwired: 1 in, 1 out]
        n470 = call "Add_to_sequence_SubVI_v1.vi"("Delay [us]"=w979, "Pulse length [us]"=w980, "Channel number"=w981, "Array sequence in"=w986) -> ("Array sequence out"=w978:cluster{"Timing 0":dbl[]}[])
      }
      event "X pi": Mouse Down {
        n471 = event-data() -> ()  [unwired: 1 in, 8 out]
        n472 = Look In Map(map=w1007, key="X pi") -> (value=w1003:dbl)  [unwired: 1 in, 1 out]
        n473 = Look In Map(map=w1007, key="Delay") -> (value=w1002:dbl)  [unwired: 1 in, 1 out]
        n474 = Look In Map(map=w1013, key="pulse X") -> (value=w1004:i32)  [unwired: 1 in, 1 out]
        n475 = Wait (ms)(milliseconds to wait=u32 150) -> ()  [unwired: 1 out]
        n476 = call "Add_to_sequence_SubVI_v1.vi"("Delay [us]"=w1002, "Pulse length [us]"=w1003, "Channel number"=w1004, "Array sequence in"=w1006) -> ("Array sequence out"=w1005:cluster{"Timing 0":dbl[]}[])
      }
      event "X pi/2": Mouse Down {
        n477 = event-data() -> ()  [unwired: 1 in, 8 out]
        n478 = Look In Map(map=w1019, key="X pi/2") -> (value=w1015:dbl)  [unwired: 1 in, 1 out]
        n479 = Look In Map(map=w1019, key="Delay") -> (value=w1014:dbl)  [unwired: 1 in, 1 out]
        n480 = Look In Map(map=w1025, key="pulse X") -> (value=w1016:i32)  [unwired: 1 in, 1 out]
        n481 = Wait (ms)(milliseconds to wait=u32 150) -> ()  [unwired: 1 out]
        n482 = call "Add_to_sequence_SubVI_v1.vi"("Delay [us]"=w1014, "Pulse length [us]"=w1015, "Channel number"=w1016, "Array sequence in"=w1018) -> ("Array sequence out"=w1017:cluster{"Timing 0":dbl[]}[])
      }
      event "X pi/4": Mouse Down {
        n483 = event-data() -> ()  [unwired: 1 in, 8 out]
        n484 = Look In Map(map=w1036, key="pulse X") -> (value=w1032:i32)  [unwired: 1 in, 1 out]
        n485 = Look In Map(map=w1034, key="X pi/4") -> (value=w1031:dbl)  [unwired: 1 in, 1 out]
        n486 = Look In Map(map=w1034, key="Delay") -> (value=w1030:dbl)  [unwired: 1 in, 1 out]
        n487 = Wait (ms)(milliseconds to wait=u32 150) -> ()  [unwired: 1 out]
        n488 = call "Add_to_sequence_SubVI_v1.vi"("Delay [us]"=w1030, "Pulse length [us]"=w1031, "Channel number"=w1032, "Array sequence in"=w1029) -> ("Array sequence out"=w1028:cluster{"Timing 0":dbl[]}[])
      }
      event "Y pi": Mouse Down {
        n489 = event-data() -> ()  [unwired: 1 in, 8 out]
        n490 = Look In Map(map=w1042, key="Y pi") -> (value=w1038:dbl)  [unwired: 1 in, 1 out]
        n491 = Look In Map(map=w1042, key="Delay") -> (value=w1037:dbl)  [unwired: 1 in, 1 out]
        n492 = Look In Map(map=w1048, key="pulse Y") -> (value=w1039:i32)  [unwired: 1 in, 1 out]
        n493 = Wait (ms)(milliseconds to wait=u32 150) -> ()  [unwired: 1 out]
        n494 = call "Add_to_sequence_SubVI_v1.vi"("Delay [us]"=w1037, "Pulse length [us]"=w1038, "Channel number"=w1039, "Array sequence in"=w1041) -> ("Array sequence out"=w1040:cluster{"Timing 0":dbl[]}[])
      }
      event "Y pi/2": Mouse Down {
        n495 = event-data() -> ()  [unwired: 1 in, 8 out]
        n496 = Look In Map(map=w1054, key="Y pi/2") -> (value=w1050:dbl)  [unwired: 1 in, 1 out]
        n497 = Look In Map(map=w1054, key="Delay") -> (value=w1049:dbl)  [unwired: 1 in, 1 out]
        n498 = Look In Map(map=w1060, key="pulse Y") -> (value=w1051:i32)  [unwired: 1 in, 1 out]
        n499 = Wait (ms)(milliseconds to wait=u32 150) -> ()  [unwired: 1 out]
        n500 = call "Add_to_sequence_SubVI_v1.vi"("Delay [us]"=w1049, "Pulse length [us]"=w1050, "Channel number"=w1051, "Array sequence in"=w1053) -> ("Array sequence out"=w1052:cluster{"Timing 0":dbl[]}[])
      }
      event "Y pi/4": Mouse Down {
        n501 = event-data() -> ()  [unwired: 1 in, 8 out]
        n502 = Look In Map(map=w1066, key="Y pi/4") -> (value=w1062:dbl)  [unwired: 1 in, 1 out]
        n503 = Look In Map(map=w1066, key="Delay") -> (value=w1061:dbl)  [unwired: 1 in, 1 out]
        n504 = Look In Map(map=w1072, key="pulse Y") -> (value=w1063:i32)  [unwired: 1 in, 1 out]
        n505 = Wait (ms)(milliseconds to wait=u32 150) -> ()  [unwired: 1 out]
        n506 = call "Add_to_sequence_SubVI_v1.vi"("Delay [us]"=w1061, "Pulse length [us]"=w1062, "Channel number"=w1063, "Array sequence in"=w1065) -> ("Array sequence out"=w1064:cluster{"Timing 0":dbl[]}[])
      }
      event "Z pi": Mouse Down {
        n507 = event-data() -> ()  [unwired: 1 in, 8 out]
        n508 = Look In Map(map=w1078, key="Z pi") -> (value=w1074:dbl)  [unwired: 1 in, 1 out]
        n509 = Look In Map(map=w1078, key="Delay") -> (value=w1073:dbl)  [unwired: 1 in, 1 out]
        n510 = Look In Map(map=w1084, key="pulse Z") -> (value=w1075:i32)  [unwired: 1 in, 1 out]
        n511 = Wait (ms)(milliseconds to wait=u32 150) -> ()  [unwired: 1 out]
        n512 = call "Add_to_sequence_SubVI_v1.vi"("Delay [us]"=w1073, "Pulse length [us]"=w1074, "Channel number"=w1075, "Array sequence in"=w1077) -> ("Array sequence out"=w1076:cluster{"Timing 0":dbl[]}[])
      }
      event "Z pi/2": Mouse Down {
        n513 = event-data() -> ()  [unwired: 1 in, 8 out]
        n514 = Look In Map(map=w1090, key="Z pi/2") -> (value=w1086:dbl)  [unwired: 1 in, 1 out]
        n515 = Look In Map(map=w1090, key="Delay") -> (value=w1085:dbl)  [unwired: 1 in, 1 out]
        n516 = Look In Map(map=w1096, key="pulse Z") -> (value=w1087:i32)  [unwired: 1 in, 1 out]
        n517 = Wait (ms)(milliseconds to wait=u32 150) -> ()  [unwired: 1 out]
        n518 = call "Add_to_sequence_SubVI_v1.vi"("Delay [us]"=w1085, "Pulse length [us]"=w1086, "Channel number"=w1087, "Array sequence in"=w1089) -> ("Array sequence out"=w1088:cluster{"Timing 0":dbl[]}[])
      }
      event "Z pi/4": Mouse Down {
        n519 = event-data() -> ()  [unwired: 1 in, 8 out]
        n520 = Look In Map(map=w1102, key="Z pi/4") -> (value=w1098:dbl)  [unwired: 1 in, 1 out]
        n521 = Look In Map(map=w1102, key="Delay") -> (value=w1097:dbl)  [unwired: 1 in, 1 out]
        n522 = Look In Map(map=w1108, key="pulse Z") -> (value=w1099:i32)  [unwired: 1 in, 1 out]
        n523 = Wait (ms)(milliseconds to wait=u32 150) -> ()  [unwired: 1 out]
        n524 = call "Add_to_sequence_SubVI_v1.vi"("Delay [us]"=w1097, "Pulse length [us]"=w1098, "Channel number"=w1099, "Array sequence in"=w1101) -> ("Array sequence out"=w1100:cluster{"Timing 0":dbl[]}[])
      }
      event "Add pulse": Mouse Down {
        # "If it is nonlinear coil, it should be waited for much more time.\nBecause the pulse shape of the nonlinear coil is not good. It still affects the atom  after the pulse pauses"
        # "The nonlinear coil value"
        n525 = event-data() -> ()  [unwired: 1 in, 8 out]
        n526 = local read "Channel"() -> (w1109:u16)
        n527 = property on="Channel" class="Ring (strict)"() -> ("Value"=w1111:u16)  [unwired: 2 in, 2 out]
        n528 = Equal?(x=w1111, y=u16 9) -> (x = y?=w1113:bool)
        n529 = Index Array(array=w1114, index=w1109) -> (element=w1122:string)
        n530 = Look In Map(map=w1123, key=w1122) -> (value=w1112:i32)  [unwired: 1 in, 1 out]
        n531 = case shown="True" w1113 {
          tunnel: w1119 -> [w1125 w1131]
          tunnel: [w1124 w1128] -> w1116
          frame False {
            n532 = Look In Map(map=w1125, key="Delay") -> (value=w1124:dbl)  [unwired: 1 in, 1 out]
          }
          frame True {
            n533 = Look In Map(map=w1131, key="Delay") -> (value=w1129:dbl)  [unwired: 1 in, 1 out]
            n534 = Add(x=50.0, y=w1129) -> (x+y=w1128:dbl)
          }
        }
        n535 = Wait (ms)(milliseconds to wait=u32 150) -> ()  [unwired: 1 out]
        n536 = call "Add_to_sequence_SubVI_v1.vi"("Delay [us]"=w1116, "Pulse length [us]"="Time [us]", "Channel number"=w1112, "Array sequence in"=w1118) -> ("Array sequence out"=w1117:cluster{"Timing 0":dbl[]}[])
      }
      event "Add pulse advanced": Mouse Down {
        # "Search for choosen channels"
        n537 = event-data() -> ()  [unwired: 1 in, 8 out]
        n538 = for {
          tunnel: "Physical channels" -> [w1151] mode=indexing
          tunnel: w1144 -> [w1152]
          tunnel: [w1150] -> w1143 mode=indexing
          tunnel: [w1148] -> w1140 mode=indexing
          n539 = Search 1D Array(1D array=w1152, element=w1151) -> (index of element=w1150:i32)  [unwired: 1 in]
          n540 = Equal?(x=w1150, y=-1) -> (x = y?=w1148:bool)
        }
        n541 = Or Array Elements(Boolean array=w1140) -> (logical OR=w1139:bool)
        n542 = case shown="True" w1139 {
          frame False {
          }
          frame True {
            n543 = One Button Dialog(message="Some port names are not correct!!!\nPulse sequance may not be correct!") -> ()  [unwired: 1 in, 1 out]
          }
        }
        n544 = for {
          tunnel: w1146 -> [w1154] mode=indexing
          tunnel: w1143 -> [w1158]
          tunnel: [w1153] -> w1136 mode=indexing
          i -> [w1157]
          n545 = for {
            tunnel: w1158 -> [w1174] mode=indexing
            tunnel: w1157 -> [w1175]
            tunnel: [w1173] -> w1156 mode=indexing
            n546 = Equal?(x=w1174, y=w1175) -> (x = y?=w1173:bool)
          }
          n547 = Or Array Elements(Boolean array=w1156) -> (logical OR=w1155:bool)
          n548 = case shown="True" w1155 {
            tunnel: w1154 -> [w1161 w1168]
            tunnel: [w1159 w1166] -> w1153
            frame True {
              n549 = local read "Time [us]"() -> (w1160:dbl)
              n550 = in-place {
                in-place-border: w1160 -> [w1164]
                n551 = in-place-cluster #9(w1161) -> ("Timing 0"=w1165:dbl[])
                n552 = Build Array (concatenate)(w1165, w1164, 0.0 ("element")) -> (w1162:dbl[])
                n553 = in-place-cluster #9("Timing 0"=w1162) -> (w1159:cluster{"Timing 0":dbl[]})
              }
            }
            frame False {
              n554 = local read "Time [us]"() -> (w1167:dbl)
              n555 = in-place {
                in-place-border: w1167 -> [w1170]
                n556 = in-place-cluster #10(w1168) -> ("Timing 0"=w1172:dbl[])
                n557 = Build Array (concatenate)(w1172, 0.0 ("element"), w1170) -> (w1171:dbl[])
                n558 = in-place-cluster #10("Timing 0"=w1171) -> (w1166:cluster{"Timing 0":dbl[]})
              }
            }
          }
        }
        n559 = Look In Map(map=w1138, key="Delay") -> (value=w1132:dbl)  [unwired: 1 in, 1 out]
        n560 = Wait (ms)(milliseconds to wait=u32 150) -> ()  [unwired: 1 out]
        n561 = call "Add_to_sequence_SubVI_v1.vi"("Delay [us]"=w1132, "Pulse length [us]"=0.0, "Channel number"=-1, "Array sequence in"=w1136) -> ("Array sequence out"=w1135:cluster{"Timing 0":dbl[]}[])
      }
      event "Save single sequence": Mouse Down {
        n562 = event-data() -> ()  [unwired: 1 in, 8 out]
        n563 = Look In Map(map=w1198, key="Accqusition TRIG") -> (value=w1188:i32)  [unwired: 1 in, 1 out]
        n564 = Look In Map(map=w1195, key="TTL") -> (value=w1187:dbl)  [unwired: 1 in, 1 out]
        n565 = Look In Map(map=w1195, key="Delay") -> (value=w1186:dbl)  [unwired: 1 in, 1 out]
        n566 = Look In Map(map=w1195, key="Probe") -> (value=w1190:dbl)  [unwired: 1 in, 1 out]
        n567 = for {
          tunnel: w1185 -> [w1207] mode=indexing
          tunnel: w1187 -> [w1206]
          tunnel: [w1205] -> w1189 mode=indexing
          tunnel: w1188 -> [w1204]
          i -> [w1203]
          n568 = Equal?(x=w1204, y=w1203) -> (x = y?=w1208:bool)
          n569 = case shown="True" w1208 {
            tunnel: w1207 -> [w1209 w1212]
            tunnel: w1206 -> [_ w1211]
            tunnel: [w1209 w1210] -> w1205
            frame False {
            }
            frame True {
              n570 = in-place {
                in-place-border: w1211 -> [w1213]
                n571 = in-place-cluster #11(w1212) -> ("Timing 0"=w1214:dbl[])
                n572 = Build Array (concatenate)(w1214, w1213) -> (w1215:dbl[])
                n573 = in-place-cluster #11("Timing 0"=w1215) -> (w1210:cluster{"Timing 0":dbl[]})
              }
            }
          }
        }
        n574 = Look In Map(map=w1198, key="Keithley TRIG") -> (value=w1193:i32)  [unwired: 1 in, 1 out]
        n575 = for {
          tunnel: w1189 -> [w1236] mode=indexing
          tunnel: w1193 -> [w1238]
          tunnel: w1187 -> [w1235]
          tunnel: w1186 -> [w1234]
          tunnel: [w1233] -> w1191 mode=indexing
          i -> [w1239]
          n576 = Equal?(x=w1239, y=w1238) -> (x = y?=w1237:bool)
          n577 = case shown="True" w1237 {
            tunnel: w1236 -> [w1240 w1244]
            tunnel: w1235 -> [_ w1243]
            tunnel: w1234 -> [_ w1242]
            tunnel: [w1240 w1241] -> w1233
            frame False {
            }
            frame True {
              n578 = in-place {
                in-place-border: w1243 -> [w1248]
                in-place-border: w1242 -> [w1247]
                n579 = in-place-cluster #12(w1244) -> ("Timing 0"=w1250:dbl[])
                n580 = Multiply(x=2.0, y=w1247) -> (x*y=w1245:dbl)
                n581 = Build Array (concatenate)(w1250, 0.0, w1245, w1248) -> (w1251:dbl[])
                n582 = in-place-cluster #12("Timing 0"=w1251) -> (w1241:cluster{"Timing 0":dbl[]})
              }
            }
          }
        }
        n583 = Look In Map(map=w1198, key="LD probe") -> (value=w1192:i32)  [unwired: 1 in, 1 out]
        n584 = flat-sequence {
          frame #0 {
            n585 = Wait (ms)(milliseconds to wait=u32 150) -> ()  [unwired: 1 out]
          }
          frame #1 {
            n586 = invoke on="Save single sequence" class="Bool (strict)" method="Reinit To Default"() -> ()  [unwired: 3 in, 3 out]
          }
        }
        n587 = for {
          tunnel: w1192 -> [w1221]
          tunnel: w1191 -> [w1219] mode=indexing
          tunnel: w1190 -> [w1218]
          tunnel: [w1217] -> w1184 mode=indexing
          tunnel: w1186 -> [w1216]
          i -> [w1222]
          n588 = Equal?(x=w1222, y=w1221) -> (x = y?=w1220:bool)
          n589 = case shown="True" w1220 {
            tunnel: w1219 -> [w1223 w1227]
            tunnel: [w1223 w1226] -> w1217
            tunnel: w1218 -> [_ w1225]
            tunnel: w1216 -> [_ w1224]
            frame False {
            }
            frame True {
              n590 = in-place {
                in-place-border: w1225 -> [w1228]
                in-place-border: w1224 -> [w1229]
                n591 = in-place-cluster #13(w1227) -> ("Timing 0"=w1231:dbl[])
                n592 = Build Array (concatenate)(w1231, 0.0, w1229, w1228) -> (w1232:dbl[])
                n593 = in-place-cluster #13("Timing 0"=w1232) -> (w1226:cluster{"Timing 0":dbl[]})
              }
            }
          }
        }
        n594 = call "Array_to_cluster_sequence_SubVI_v1.vi"("Array"=w1184) -> ("Sequence"=w1183:T6)
        n595 = local read "Sampling data"() -> (w1181:T2)
        n596 = local read "Config folder"() -> (w1178:string)
        n597 = Concatenate Strings(w1178, "\\pulse_sequence_DAQ.ini" ("string")) -> (w1176:string)
        n598 = call "Set_Pulse_Seq_DAQ.vi"("Time Unit"=T12 {"Time Unit"=enum."MicroSecond"}, "error in"=w1180, "Sampling data"=w1181, "Sequence"=w1183, "Filename (ini)"=w1176) -> ("error out"=w1179:errorcluster)  [unwired: 6 in]
      }
      event "Save multi Sequence": Mouse Down {
        n599 = event-data() -> ()  [unwired: 1 in, 8 out]
        n600 = local read "Config folder"() -> (w1255:string)
        n601 = call <vilib>:"Application Directory.vi"() -> ("Application Directory"=w1264:path)
        n602 = Concatenate Strings(w1255, "\\temp_multi_FID\\" ("string")) -> (w1254:string)
        n603 = Concatenate Strings("Config_Files\\" ("string"), w1254) -> (w1261:string)
        n604 = String To Path(string=w1261) -> (path=w1263:path)
        n605 = Build Path(base path=w1264, name or relative path=w1263) -> (appended path=w1262:path)
        n606 = call <userlib>:"List Directory__ogtk.vi"("directory path"=w1262) -> ("file names"=w1260:string[])  [unwired: 3 in, 3 out]
        n607 = for {
          tunnel: w1260 -> [w1270] mode=indexing
          shift-right: [w1271] -> w1259
          shift-left: w1258 -> [w1272]
          tunnel: w1254 -> [w1269]
          n608 = Concatenate Strings(w1269, w1270) -> (w1273:string)
          n609 = call "Delete_file.vi"("error in"=w1272, "Filename (ini)"=w1273) -> ("error out"=w1271:errorcluster)  [unwired: 9 in]
        }
        n610 = local read "Period number"() -> (w1253:u32)
        n611 = local read "Period [us]"() -> (w1252:dbl)
        n612 = for {
          N: w1253 -> [_]
          tunnel: w1268 -> [w1281]
          tunnel: w1267 -> [w1278]
          tunnel: w1266 -> [w1287]
          tunnel: w1252 -> [w1303]
          tunnel: w1259 -> [w1295]
          tunnel: [w1293] -> w1265
          i -> [w1289]
          # "Write the full number in the name to store the data\n 1-->001\n10-->010\n100-->100"
          n613 = Multiply(x=w1303, y=w1289) -> (x*y=w1285:dbl)
          n614 = Look In Map(map=w1278, key="Delay") -> (value=w1284:dbl)  [unwired: 1 in, 1 out]
          n615 = Look In Map(map=w1281, key="Nonlinear coil") -> (value=w1286:i32)  [unwired: 1 in, 1 out]
          n616 = Look In Map(map=w1278, key="Delay") -> (value=w1275:dbl)  [unwired: 1 in, 1 out]
          n617 = Look In Map(map=w1278, key="Probe") -> (value=w1307:dbl)  [unwired: 1 in, 1 out]
          n618 = Look In Map(map=w1278, key="TTL") -> (value=w1304:dbl)  [unwired: 1 in, 1 out]
          n619 = Look In Map(map=w1281, key="pulse X") -> (value=w1279:i32)  [unwired: 1 in, 1 out]
          n620 = call "Add_to_sequence_SubVI_Directly.vi"("Delay [us]"=w1284, "Pulse length [us]"=w1285, "Channel number"=w1286, "Array sequence in"=w1287) -> ("Array sequence out"=w1283:cluster{"Timing 0":dbl[]}[])
          n621 = Look In Map(map=w1278, key="X pi/4") -> (value=w1276:dbl)  [unwired: 1 in, 1 out]
          n622 = call "Add_to_sequence_SubVI_v1.vi"("Delay [us]"=w1275, "Pulse length [us]"=w1276, "Channel number"=w1279, "Array sequence in"=w1283) -> ("Array sequence out"=w1282:cluster{"Timing 0":dbl[]}[])
          n623 = Look In Map(map=w1281, key="Accqusition TRIG") -> (value=w1305:i32)  [unwired: 1 in, 1 out]
          n624 = for {
            tunnel: w1282 -> [w1337] mode=indexing
            tunnel: w1304 -> [w1336]
            tunnel: [w1335] -> w1306 mode=indexing
            tunnel: w1305 -> [w1334]
            i -> [w1333]
            n625 = Equal?(x=w1334, y=w1333) -> (x = y?=w1338:bool)
            n626 = case shown="True" w1338 {
              tunnel: w1337 -> [w1339 w1342]
              tunnel: w1336 -> [_ w1341]
              tunnel: [w1339 w1340] -> w1335
              frame False {
              }
              frame True {
                n627 = in-place {
                  in-place-border: w1341 -> [w1343]
                  n628 = in-place-cluster #14(w1342) -> ("Timing 0"=w1344:dbl[])
                  n629 = Build Array (concatenate)(w1344, w1343) -> (w1345:dbl[])
                  n630 = in-place-cluster #14("Timing 0"=w1345) -> (w1340:cluster{"Timing 0":dbl[]})
                }
              }
            }
          }
          n631 = Look In Map(map=w1281, key="LD probe") -> (value=w1309:i32)  [unwired: 1 in, 1 out]
          n632 = Look In Map(map=w1281, key="Keithley TRIG") -> (value=w1310:i32)  [unwired: 1 in, 1 out]
          n633 = for {
            tunnel: w1306 -> [w1366] mode=indexing
            tunnel: w1310 -> [w1368]
            tunnel: w1304 -> [w1365]
            tunnel: w1275 -> [w1364]
            tunnel: [w1363] -> w1308 mode=indexing
            i -> [w1369]
            n634 = Equal?(x=w1369, y=w1368) -> (x = y?=w1367:bool)
            n635 = case shown="True" w1367 {
              tunnel: w1366 -> [w1370 w1374]
              tunnel: w1365 -> [_ w1373]
              tunnel: w1364 -> [_ w1372]
              tunnel: [w1370 w1371] -> w1363
              frame False {
              }
              frame True {
                n636 = in-place {
                  in-place-border: w1373 -> [w1378]
                  in-place-border: w1372 -> [w1377]
                  n637 = in-place-cluster #15(w1374) -> ("Timing 0"=w1380:dbl[])
                  n638 = Multiply(x=2.0, y=w1377) -> (x*y=w1375:dbl)
                  n639 = Build Array (concatenate)(w1380, 0.0, w1375, w1378) -> (w1381:dbl[])
                  n640 = in-place-cluster #15("Timing 0"=w1381) -> (w1371:cluster{"Timing 0":dbl[]})
                }
              }
            }
          }
          n641 = for {
            tunnel: w1309 -> [w1351]
            tunnel: w1308 -> [w1349] mode=indexing
            tunnel: w1307 -> [w1348]
            tunnel: [w1347] -> w1301 mode=indexing
            tunnel: w1275 -> [w1346]
            i -> [w1352]
            n642 = Equal?(x=w1352, y=w1351) -> (x = y?=w1350:bool)
            n643 = case shown="True" w1350 {
              tunnel: w1349 -> [w1353 w1357]
              tunnel: [w1353 w1356] -> w1347
              tunnel: w1348 -> [_ w1355]
              tunnel: w1346 -> [_ w1354]
              frame False {
              }
              frame True {
                n644 = in-place {
                  in-place-border: w1355 -> [w1358]
                  in-place-border: w1354 -> [w1359]
                  n645 = in-place-cluster #16(w1357) -> ("Timing 0"=w1361:dbl[])
                  n646 = Build Array (concatenate)(w1361, 0.0, w1359, w1358) -> (w1362:dbl[])
                  n647 = in-place-cluster #16("Timing 0"=w1362) -> (w1356:cluster{"Timing 0":dbl[]})
                }
              }
            }
          }
          n648 = Less?(x=w1289, y=10) -> (x < y?=w1290:bool)
          n649 = case shown="False" w1290 {
            tunnel: [w1317 w1328] -> w1288
            tunnel: w1289 -> [w1318 w1331]
            frame False {
              n650 = Less?(x=w1318, y=100) -> (x < y?=w1319:bool)
              n651 = case shown="False" w1319 {
                tunnel: w1318 -> [w1322 w1326]
                tunnel: [w1321 w1323] -> w1317
                frame False {
                  (unwired) i16 1 ("width (-)")
                  n652 = Number To Decimal String(number=w1322) -> (decimal integer string=w1321:string)  [unwired: 1 in]
                }
                frame True {
                  n653 = Number To Decimal String(number=w1326, width (-)=i16 1) -> (decimal integer string=w1325:string)
                  n654 = Concatenate Strings("0" ("string"), w1325) -> (w1323:string)
                }
              }
            }
            frame True {
              n655 = Number To Decimal String(number=w1331, width (-)=i16 1) -> (decimal integer string=w1330:string)
              n656 = Concatenate Strings("00" ("string"), w1330) -> (w1328:string)
            }
          }
          n657 = call "Array_to_cluster_sequence_SubVI_v1.vi"("Array"=w1301) -> ("Sequence"=w1294:T6)
          n658 = local read "Sampling data"() -> (w1298:T2)
          n659 = local read "Config folder"() -> (w1299:string)
          n660 = Concatenate Strings(w1299, "\\temp_multi_FID\\Single_FID_" ("string"), w1288, ".ini" ("string")) -> (w1300:string)
          n661 = call "Set_Pulse_Seq_DAQ.vi"("Time Unit"=T12 {"Time Unit"=enum."MicroSecond"}, "error in"=w1295, "Sampling data"=w1298, "Sequence"=w1294, "Filename (ini)"=w1300) -> ("error out"=w1293:errorcluster)  [unwired: 6 in]
        }
        n662 = flat-sequence {
          frame #0 {
            n663 = Wait (ms)(milliseconds to wait=u32 150) -> ()  [unwired: 1 out]
          }
          frame #1 {
            n664 = invoke on="Save single sequence" class="Bool (strict)" method="Reinit To Default"() -> ()  [unwired: 3 in, 3 out]
          }
        }
      }
      event "Save multi-process": Mouse Down {
        # "Clear All processes files"
        n665 = event-data() -> ()  [unwired: 1 in, 8 out]
        n666 = local read "Config folder"() -> (w1386:string)
        n667 = call <vilib>:"Application Directory.vi"() -> ("Application Directory"=w1395:path)
        n668 = Concatenate Strings(w1386, "\\process\\processes_sets\\" ("string")) -> (w1385:string)
        n669 = Concatenate Strings("Config_Files\\" ("string"), w1385) -> (w1392:string)
        n670 = String To Path(string=w1392) -> (path=w1394:path)
        n671 = Build Path(base path=w1395, name or relative path=w1394) -> (appended path=w1393:path)
        n672 = call <userlib>:"List Directory__ogtk.vi"("directory path"=w1393) -> ("file names"=w1391:string[])  [unwired: 3 in, 3 out]
        n673 = for {
          tunnel: w1391 -> [w1401] mode=indexing
          shift-right: [w1402] -> w1390
          shift-left: w1389 -> [w1403]
          tunnel: w1385 -> [w1400]
          n674 = Concatenate Strings(w1400, w1401) -> (w1404:string)
          n675 = call "Delete_file.vi"("error in"=w1403, "Filename (ini)"=w1404) -> ("error out"=w1402:errorcluster)  [unwired: 9 in]
        }
        n676 = local read "Period number"() -> (w1384:u32)
        n677 = local read "Period [us]"() -> (w1383:dbl)
        n678 = for {
          N: w1384 -> [_]
          tunnel: w1399 -> [w1410]
          tunnel: w1398 -> [w1409]
          tunnel: w1397 -> [w1414]
          tunnel: w1383 -> [w1429]
          tunnel: w1390 -> [w1422]
          tunnel: [w1420] -> w1396
          i -> [w1416]
          # "Write the full number in the name to store the data\n 1-->001\n10-->010\n100-->100"
          n679 = property on="Channel" class="Ring (strict)"() -> ("Strings []"=w1405:string[])  [unwired: 2 in, 2 out]
          n680 = property on="Channel" class="Ring (strict)"() -> ("Value"=w1406:u16)  [unwired: 2 in, 2 out]
          n681 = Index Array(array=w1405, index=w1406) -> (element=w1407:string)
          n682 = Multiply(x=w1429, y=w1416) -> (x*y=w1412:dbl)
          n683 = Look In Map(map=w1410, key=w1407) -> (value=w1413:i32)  [unwired: 1 in, 1 out]
          n684 = Look In Map(map=w1409, key="Delay") -> (value=w1411:dbl)  [unwired: 1 in, 1 out]
          n685 = call "Add_to_sequence_SubVI_Directly.vi"("Delay [us]"=w1411, "Pulse length [us]"=w1412, "Channel number"=w1413, "Array sequence in"=w1414) -> ("Array sequence out"=w1408:cluster{"Timing 0":dbl[]}[])
          n686 = Less?(x=w1416, y=10) -> (x < y?=w1417:bool)
          n687 = case shown="False" w1417 {
            tunnel: [w1430 w1441] -> w1415
            tunnel: w1416 -> [w1431 w1444]
            frame False {
              n688 = Less?(x=w1431, y=100) -> (x < y?=w1432:bool)
              n689 = case shown="False" w1432 {
                tunnel: w1431 -> [w1435 w1439]
                tunnel: [w1434 w1436] -> w1430
                frame False {
                  (unwired) i16 1 ("width (-)")
                  n690 = Number To Decimal String(number=w1435) -> (decimal integer string=w1434:string)  [unwired: 1 in]
                }
                frame True {
                  n691 = Number To Decimal String(number=w1439, width (-)=i16 1) -> (decimal integer string=w1438:string)
                  n692 = Concatenate Strings("0" ("string"), w1438) -> (w1436:string)
                }
              }
            }
            frame True {
              n693 = Number To Decimal String(number=w1444, width (-)=i16 1) -> (decimal integer string=w1443:string)
              n694 = Concatenate Strings("00" ("string"), w1443) -> (w1441:string)
            }
          }
          n695 = call "Array_to_cluster_sequence_SubVI_v1.vi"("Array"=w1408) -> ("Sequence"=w1421:T6)
          n696 = local read "Sampling data"() -> (w1425:T2)
          n697 = local read "Config folder"() -> (w1426:string)
          n698 = Concatenate Strings(w1426, "\\process\\processes_sets\\Processes_" ("string"), w1415, ".ini" ("string")) -> (w1427:string)
          n699 = call "Set_Pulse_Seq_DAQ.vi"("Time Unit"=T12 {"Time Unit"=enum."MicroSecond"}, "error in"=w1422, "Sampling data"=w1425, "Sequence"=w1421, "Filename (ini)"=w1427) -> ("error out"=w1420:errorcluster)  [unwired: 6 in]
        }
        n700 = flat-sequence {
          frame #0 {
            n701 = Wait (ms)(milliseconds to wait=u32 150) -> ()  [unwired: 1 out]
          }
          frame #1 {
            n702 = invoke on="Save single sequence" class="Bool (strict)" method="Reinit To Default"() -> ()  [unwired: 3 in, 3 out]
          }
        }
      }
      event "Save for tomography": Mouse Down {
        w1453 = string[][] [["None", "None"], ["Y pi", "None"], ["Z pi/2", "Y pi"]]
        w1447 = string[] ["None", "Y pi/2", "X pi/2"]
        # "Additional delay to ensure that\nall measurement start at the\nsame moment"
        # "CYCLOPS"
        # "Control pulses"
        n703 = event-data() -> ()  [unwired: 1 in, 8 out]
        n704 = local write "pulses type (priv)"(w1447) -> ()
        n705 = for {
          tunnel: w1455 -> [w1583]
          tunnel: w1447 -> [w1582] mode=indexing
          tunnel: [w1581] -> w1462 mode=indexing
          # "Check longest control pulse"
          n706 = Look In Map(map=w1583, key=w1582) -> (value=w1581:dbl)  [unwired: 1 in, 1 out]
        }
        n707 = Look In Map(map=w1455, key="Delay") -> (value=w1460:dbl)  [unwired: 1 in, 1 out]
        n708 = for {
          tunnel: w1455 -> [w1589]
          tunnel: w1453 -> [w1588] mode=indexing
          tunnel: w1460 -> [w1585]
          tunnel: [w1584] -> w1461 mode=indexing
          # "Check longest CYCLOPS sequence"
          n709 = for {
            tunnel: w1589 -> [w1592]
            tunnel: [w1591] -> w1587 mode=indexing
            tunnel: w1588 -> [w1590] mode=indexing
            n710 = Look In Map(map=w1592, key=w1590) -> (value=w1591:dbl)  [unwired: 1 in, 1 out]
          }
          n711 = Add Array Elements(numeric array=w1587) -> (sum=w1586:dbl)
          n712 = Add(x=w1586, y=w1585) -> (x+y=w1584:dbl)
        }
        n713 = for {
          tunnel: w1462 -> [w1579] mode=indexing
          tunnel: w1461 -> [w1580]
          tunnel: w1460 -> [w1577]
          tunnel: [w1578] -> w1458 mode=indexing
          n714 = Compound Arithmetic op=unknown(w1580, w1577, w1579, w1577) -> (w1578:dbl[])
        }
        n715 = Array Max & Min(array=w1458) -> (max value=w1459:dbl)  [unwired: 3 out]
        n716 = Subtract(x=w1459, y=w1458) -> (x-y=w1452:dbl[][])
        n717 = for {
          tunnel: string[] ["None", "pulse Y", "pulse X"] -> [w1489] mode=indexing
          tunnel: w1447 -> [w1490] mode=indexing
          tunnel: w1451 -> [w1491]
          tunnel: w1456 -> [w1480]
          tunnel: w1455 -> [w1481]
          tunnel: string[][] [["None", "None"], ["pulse Y", "None"], ["pulse Z", "pulse Y"]] -> [w1484]
          tunnel: w1453 -> [w1483]
          tunnel: [w1479] -> w1450 mode=concatenating
          tunnel: w1452 -> [w1478] mode=indexing
          # "Iterate over control pulses"
          n718 = Look In Map(map=w1480, key=w1489) -> (value=w1487:i32)  [unwired: 1 in, 1 out]
          n719 = Look In Map(map=w1481, key=w1490) -> (value=w1486:dbl)  [unwired: 1 in, 1 out]
          n720 = Look In Map(map=w1481, key="Delay") -> (value=w1482:dbl)  [unwired: 1 in, 1 out]
          n721 = call "Add_to_sequence_SubVI_v1.vi"("Delay [us]"=w1482, "Pulse length [us]"=w1486, "Channel number"=w1487, "Array sequence in"=w1491) -> ("Array sequence out"=w1485:cluster{"Timing 0":dbl[]}[])
          n722 = for {
            tunnel: w1485 -> [w1518]
            tunnel: w1484 -> [w1515] mode=indexing
            tunnel: w1483 -> [w1516] mode=indexing
            tunnel: w1482 -> [w1517]
            tunnel: w1481 -> [w1500]
            tunnel: w1480 -> [w1496]
            tunnel: [w1499] -> w1479 mode=indexing
            tunnel: w1478 -> [w1494] mode=indexing
            # "Add equalization of the time interval"
            # "Iterate over CYCLOPS in 2 for loops because CYCLOPS consists of a few pulses"
            n723 = for {
              shift-right: [w1569] -> w1498
              shift-left: w1518 -> [w1572]
              tunnel: w1517 -> [w1568]
              tunnel: w1516 -> [w1575] mode=indexing
              tunnel: w1515 -> [w1576] mode=indexing
              tunnel: w1500 -> [w1574]
              tunnel: w1496 -> [w1573]
              tunnel: [w1568] -> w1493
              n724 = Look In Map(map=w1573, key=w1576) -> (value=w1571:i32)  [unwired: 1 in, 1 out]
              n725 = Look In Map(map=w1574, key=w1575) -> (value=w1570:dbl)  [unwired: 1 in, 1 out]
              n726 = call "Add_to_sequence_SubVI_v1.vi"("Delay [us]"=w1568, "Pulse length [us]"=w1570, "Channel number"=w1571, "Array sequence in"=w1572) -> ("Array sequence out"=w1569:cluster{"Timing 0":dbl[]}[])
            }
            n727 = Look In Map(map=w1496, key="None") -> (value=w1495:i32)  [unwired: 1 in, 1 out]
            n728 = call "Add_to_sequence_SubVI_v1.vi"("Delay [us]"=w1493, "Pulse length [us]"=w1494, "Channel number"=w1495, "Array sequence in"=w1498) -> ("Array sequence out"=w1492:cluster{"Timing 0":dbl[]}[])
            n729 = Look In Map(map=w1500, key="Probe") -> (value=w1510:dbl)  [unwired: 1 in, 1 out]
            n730 = Look In Map(map=w1500, key="Delay") -> (value=w1514:dbl)  [unwired: 1 in, 1 out]
            n731 = Look In Map(map=w1496, key="Accqusition TRIG") -> (value=w1512:i32)  [unwired: 1 in, 1 out]
            n732 = Look In Map(map=w1500, key="TTL") -> (value=w1513:dbl)  [unwired: 1 in, 1 out]
            n733 = for {
              tunnel: w1492 -> [w1523] mode=indexing
              tunnel: w1513 -> [w1522]
              tunnel: [w1521] -> w1511 mode=indexing
              tunnel: w1512 -> [w1520]
              i -> [w1519]
              n734 = Equal?(x=w1520, y=w1519) -> (x = y?=w1524:bool)
              n735 = case shown="True" w1524 {
                tunnel: w1523 -> [w1525 w1528]
                tunnel: w1522 -> [_ w1527]
                tunnel: [w1525 w1526] -> w1521
                frame False {
                }
                frame True {
                  n736 = in-place {
                    in-place-border: w1527 -> [w1529]
                    n737 = in-place-cluster #17(w1528) -> ("Timing 0"=w1530:dbl[])
                    n738 = Build Array (concatenate)(w1530, w1529) -> (w1531:dbl[])
                    n739 = in-place-cluster #17("Timing 0"=w1531) -> (w1526:cluster{"Timing 0":dbl[]})
                  }
                }
              }
            }
            n740 = Look In Map(map=w1496, key="Keithley TRIG") -> (value=w1507:i32)  [unwired: 1 in, 1 out]
            n741 = for {
              tunnel: w1511 -> [w1552] mode=indexing
              tunnel: w1507 -> [w1554]
              tunnel: w1513 -> [w1551]
              tunnel: w1514 -> [w1550]
              tunnel: [w1549] -> w1509 mode=indexing
              i -> [w1555]
              n742 = Equal?(x=w1555, y=w1554) -> (x = y?=w1553:bool)
              n743 = case shown="True" w1553 {
                tunnel: w1552 -> [w1556 w1560]
                tunnel: w1551 -> [_ w1559]
                tunnel: w1550 -> [_ w1558]
                tunnel: [w1556 w1557] -> w1549
                frame False {
                }
                frame True {
                  n744 = in-place {
                    in-place-border: w1559 -> [w1564]
                    in-place-border: w1558 -> [w1563]
                    n745 = in-place-cluster #18(w1560) -> ("Timing 0"=w1566:dbl[])
                    n746 = Multiply(x=2.0, y=w1563) -> (x*y=w1561:dbl)
                    n747 = Build Array (concatenate)(w1566, 0.0, w1561, w1564) -> (w1567:dbl[])
                    n748 = in-place-cluster #18("Timing 0"=w1567) -> (w1557:cluster{"Timing 0":dbl[]})
                  }
                }
              }
            }
            n749 = Look In Map(map=w1496, key="LD probe") -> (value=w1508:i32)  [unwired: 1 in, 1 out]
            n750 = for {
              tunnel: w1508 -> [w1537]
              tunnel: w1509 -> [w1535] mode=indexing
              tunnel: w1510 -> [w1534]
              tunnel: [w1533] -> w1499 mode=indexing
              tunnel: w1514 -> [w1532]
              i -> [w1538]
              n751 = Equal?(x=w1538, y=w1537) -> (x = y?=w1536:bool)
              n752 = case shown="True" w1536 {
                tunnel: w1535 -> [w1539 w1543]
                tunnel: [w1539 w1542] -> w1533
                tunnel: w1534 -> [_ w1541]
                tunnel: w1532 -> [_ w1540]
                frame False {
                }
                frame True {
                  n753 = in-place {
                    in-place-border: w1541 -> [w1544]
                    in-place-border: w1540 -> [w1545]
                    n754 = in-place-cluster #19(w1543) -> ("Timing 0"=w1547:dbl[])
                    n755 = Build Array (concatenate)(w1547, 0.0, w1545, w1544) -> (w1548:dbl[])
                    n756 = in-place-cluster #19("Timing 0"=w1548) -> (w1542:cluster{"Timing 0":dbl[]})
                  }
                }
              }
            }
          }
        }
        n757 = flat-sequence {
          frame #0 {
            n758 = Wait (ms)(milliseconds to wait=u32 150) -> ()  [unwired: 1 out]
          }
          frame #1 {
            n759 = invoke on="Save for tomography" class="Bool (strict)" method="Reinit To Default"() -> ()  [unwired: 3 in, 3 out]
          }
        }
        n760 = for {
          tunnel: w1450 -> [w1477] mode=indexing
          shift-right: [w1465] -> w1448
          shift-left: w1449 -> [w1475]
          i -> [w1470]
          n761 = local read "Config folder"() -> (w1472:string)
          n762 = Number To Decimal String(number=w1470, width (-)=i16 1) -> (decimal integer string=w1468:string)
          n763 = call "Array_to_cluster_sequence_SubVI_v1.vi"("Array"=w1477) -> ("Sequence"=w1476:T6)
          n764 = local read "Sampling data"() -> (w1474:T2)
          n765 = Concatenate Strings(w1472, "\\tomography\\pulse_seq_DAQ_" ("string"), w1468, ".ini" ("string")) -> (w1466:string)
          n766 = call "Set_Pulse_Seq_DAQ.vi"("Time Unit"=T12 {"Time Unit"=enum."MicroSecond"}, "error in"=w1475, "Sampling data"=w1474, "Sequence"=w1476, "Filename (ini)"=w1466) -> ("error out"=w1465:errorcluster)  [unwired: 6 in]
        }
      }
      event "Save initial state": Mouse Down {
        n767 = event-data() -> ()  [unwired: 1 in, 8 out]
        n768 = String Length(string="Name of state (initial_state_)") -> (length=w1598:i32)
        n769 = Greater Than 0?(x=w1598) -> (x > 0?=w1597:bool)
        n770 = case shown="False" w1597 {
          tunnel: "Name of state (initial_state_)" -> [_ w1619]
          tunnel: [w1606 w1612] -> w1595
          tunnel: w1594 -> [w1605 w1613]
          tunnel: w1593 -> [w1604 w1614]
          frame False {
            # "Select a Name from the Ring to Save the initial_state in the State_library"
            n771 = property on="Name of initial_state" class="Ring (strict)"() -> ("Strings []"=w1611:string[])  [unwired: 2 in, 2 out]
            n772 = Index Array(array=w1611, index="Name of initial_state") -> (element=w1608:string)
            n773 = call "Array_to_cluster_sequence_SubVI_v1.vi"("Array"=w1604) -> ("Sequence"=w1603:T6)
            n774 = local read "Config folder"() -> (w1599:string)
            n775 = local read "Sampling data"() -> (w1602:T2)
            n776 = Concatenate Strings(w1599, "\\state_library\\" ("string"), w1608, ".ini" ("string")) -> (w1601:string)
            n777 = call "Set_Pulse_Seq_DAQ.vi"("Time Unit"=T12 {"Time Unit"=enum."MicroSecond"}, "error in"=w1605, "Sampling data"=w1602, "Sequence"=w1603, "Filename (ini)"=w1601) -> ("error out"=w1606:errorcluster)  [unwired: 6 in]
          }
          frame True {
            w1616 = "initial_state_" ("true string")
            n778 = Match True/False String(2:"" ("false string"), 3:w1616, 4:w1619) -> (0:w1617:bool, 1:w1615:string)
            n779 = case shown="True" w1617 {
              tunnel: w1616 -> [_ w1639]
              tunnel: w1615 -> [_ w1638]
              tunnel: w1614 -> [_ w1637]
              tunnel: w1613 -> [w1620 w1630]
              tunnel: [w1620 w1629] -> w1612
              frame False {
                n780 = xnode "Error Ring"() -> ("error out"=w1621:errorcluster)
                n781 = call <vilib>:"Simple Error Handler.vi"("error in (no error)"=w1621) -> ()  [unwired: 4 in, 5 out]
              }
              frame True {
                # "input the name by yourself, but name pattern should be like initial_satae_"
                n782 = Concatenate Strings(w1639, w1638) -> (w1633:string)
                n783 = call "Array_to_cluster_sequence_SubVI_v1.vi"("Array"=w1637) -> ("Sequence"=w1636:T6)
                n784 = local read "Config folder"() -> (w1627:string)
                n785 = local read "Sampling data"() -> (w1631:T2)
                n786 = Concatenate Strings(w1627, "\\state_library\\" ("string"), w1633, ".ini" ("string")) -> (w1632:string)
                n787 = call "Set_Pulse_Seq_DAQ.vi"("Time Unit"=T12 {"Time Unit"=enum."MicroSecond"}, "error in"=w1630, "Sampling data"=w1631, "Sequence"=w1636, "Filename (ini)"=w1632) -> ("error out"=w1629:errorcluster)  [unwired: 6 in]
              }
            }
          }
        }
      }
      event "Save  process": Mouse Down {
        n788 = event-data() -> ()  [unwired: 1 in, 8 out]
        n789 = String Length(string="Name of process (process_)") -> (length=w1645:i32)
        n790 = Greater Than 0?(x=w1645) -> (x > 0?=w1644:bool)
        n791 = case shown="True" w1644 {
          tunnel: "Name of process (process_)" -> [_ w1666]
          tunnel: [w1653 w1659] -> w1642
          tunnel: w1641 -> [w1652 w1660]
          tunnel: w1640 -> [w1651 w1661]
          frame False {
            # "Select a Name from the Ring to Save the process in the processes"
            n792 = property on="Name of process" class="Ring (strict)"() -> ("Strings []"=w1658:string[])  [unwired: 2 in, 2 out]
            n793 = Index Array(array=w1658, index="Name of process") -> (element=w1655:string)
            n794 = call "Array_to_cluster_sequence_SubVI_v1.vi"("Array"=w1651) -> ("Sequence"=w1650:T6)
            n795 = local read "Config folder"() -> (w1646:string)
            n796 = local read "Sampling data"() -> (w1649:T2)
            n797 = Concatenate Strings(w1646, "\\process_library\\" ("string"), w1655, ".ini" ("string")) -> (w1648:string)
            n798 = call "Set_Pulse_Seq_DAQ.vi"("Time Unit"=T12 {"Time Unit"=enum."MicroSecond"}, "error in"=w1652, "Sampling data"=w1649, "Sequence"=w1650, "Filename (ini)"=w1648) -> ("error out"=w1653:errorcluster)  [unwired: 6 in]
          }
          frame True {
            w1663 = "process_" ("true string")
            n799 = Match True/False String(2:"" ("false string"), 3:w1663, 4:w1666) -> (0:w1664:bool, 1:w1662:string)
            n800 = case shown="True" w1664 {
              tunnel: w1663 -> [_ w1686]
              tunnel: w1662 -> [_ w1685]
              tunnel: w1661 -> [_ w1684]
              tunnel: w1660 -> [w1667 w1677]
              tunnel: [w1667 w1676] -> w1659
              frame False {
                n801 = xnode "Error Ring"() -> ("error out"=w1668:errorcluster)
                n802 = call <vilib>:"Simple Error Handler.vi"("error in (no error)"=w1668) -> ()  [unwired: 4 in, 5 out]
              }
              frame True {
                # "input the name by yourself, but name pattern should be like process_"
                n803 = Concatenate Strings(w1686, w1685) -> (w1680:string)
                n804 = call "Array_to_cluster_sequence_SubVI_v1.vi"("Array"=w1684) -> ("Sequence"=w1683:T6)
                n805 = local read "Config folder"() -> (w1674:string)
                n806 = local read "Sampling data"() -> (w1678:T2)
                n807 = Concatenate Strings(w1674, "\\process_library\\" ("string"), w1680, ".ini" ("string")) -> (w1679:string)
                n808 = call "Set_Pulse_Seq_DAQ.vi"("Time Unit"=T12 {"Time Unit"=enum."MicroSecond"}, "error in"=w1677, "Sampling data"=w1678, "Sequence"=w1683, "Filename (ini)"=w1679) -> ("error out"=w1676:errorcluster)  [unwired: 6 in]
              }
            }
          }
        }
      }
      event "Save QPT": Mouse Down {
        w1709 = "\\process\\init_states_sets\\" ("string")
        # "1. Clear all files in the temp_states"
        n809 = event-data() -> ()  [unwired: 1 in, 8 out]
        n810 = local read "Config folder"() -> (w1693:string)
        n811 = Concatenate Strings(w1693, "\\process\\temp_states\\" ("string")) -> (w1698:string)
        n812 = Concatenate Strings(w1693, "\\process\\processes_sets\\" ("string")) -> (w1692:string)
        n813 = Concatenate Strings("Config_Files\\" ("string"), w1698) -> (w1702:string)
        n814 = call "Read_filename.vi"("error in"=w1696, "Filename (ini)"=w1692) -> ("error out"=w1691:errorcluster, "Strings []"=w1694:string[])  [unwired: 8 in]
        n815 = call <vilib>:"Application Directory.vi"() -> ("Application Directory"=w1705:path)
        n816 = String To Path(string=w1702) -> (path=w1704:path)
        n817 = Build Path(base path=w1705, name or relative path=w1704) -> (appended path=w1703:path)
        n818 = Array Size(array=w1694) -> (size(s)=w1695:i32)
        n819 = Concatenate Strings(w1693, w1709) -> (w1711:string)
        n820 = call <userlib>:"List Directory__ogtk.vi"("directory path"=w1703) -> ("file names"=w1700:string[])  [unwired: 3 in, 3 out]
        n821 = for {
          tunnel: w1700 -> [w1785] mode=indexing
          shift-right: [w1786] -> w1699
          shift-left: w1696 -> [w1787]
          tunnel: w1698 -> [w1784]
          n822 = Concatenate Strings(w1784, w1785) -> (w1788:string)
          n823 = call "Delete_file.vi"("error in"=w1787, "Filename (ini)"=w1788) -> ("error out"=w1786:errorcluster)  [unwired: 9 in]
        }
        n824 = call "Read_filename.vi"("error in"=w1699, "Filename (ini)"=w1711) -> ("error out"=w1707:errorcluster, "Strings []"=w1708:string[])  [unwired: 8 in]
        n825 = for {
          N: w1695 -> [_]
          tunnel: w1694 -> [w1782] mode=indexing
          tunnel: w1692 -> [w1783]
          shift-right: [w1779] -> w1688
          shift-left: w1691 -> [w1780]
          tunnel: [w1777] -> w1687 mode=indexing
          n826 = Concatenate Strings(w1783, w1782) -> (w1781:string)
          n827 = call "Get_Pulse_Seq_DAQ.vi"("error in"=w1780, "Filename (ini)"=w1781) -> ("error out"=w1779:errorcluster, "data"=w1778:T6)  [unwired: 8 in]
          n828 = call "Squence_to_Array_SubVI.vi"("Sequence"=w1778) -> ("Array"=w1777:cluster{"Timing 0":dbl[]}[])  [unwired: 10 in]
        }
        n829 = Array Size(array=w1708) -> (size(s)=w1710:i32)
        "Initial State Numbers" <- w1710
        n830 = Initialize Array(0.0 ("element"), w1710) -> (w1717:dbl[])
        n831 = for {
          N: w1710 -> [_]
          shift-right: [w1815] -> w1690
          shift-left: w1707 -> [w1817]
          shift-right: [w1807] -> w1715
          shift-left: w1717 -> [w1809]
          tunnel: [w1804] -> w1716 mode=indexing
          tunnel: w1693 -> [w1802]
          tunnel: w1709 -> [w1801]
          tunnel: w1708 -> [w1800] mode=indexing
          i -> [w1808]
          # "3.Look for the longest Time Sequence from the initial_State"
          # "2.Read the initial_state data from the files"
          n832 = Concatenate Strings(w1802, w1801, w1800) -> (w1816:string)
          n833 = call "Get_Pulse_Seq_DAQ.vi"("error in"=w1817, "Filename (ini)"=w1816) -> ("error out"=w1815:errorcluster, "data"=w1814:T6)  [unwired: 8 in]
          n834 = call "Squence_to_Array_SubVI.vi"("Sequence"=w1814) -> ("Array"=w1804:cluster{"Timing 0":dbl[]}[])  [unwired: 10 in]
          n835 = Index Array(array=w1804, index=0) -> (element=w1811:cluster{"Timing 0":dbl[]})
          n836 = Unbundle(w1811) -> ("Timing 0"=w1812:dbl[])
          n837 = for {
            tunnel: w1812 -> [w1819] mode=indexing
            shift-right: [w1818] -> w1805
            shift-left: 0 -> [w1820]
            n838 = Add(x=w1819, y=w1820) -> (x+y=w1818:dbl)
          }
          n839 = local read "MaxTime"() -> (w1806:dbl)
          n840 = Max & Min(x=w1806, y=w1805) -> (max(x,y)=w1810:dbl)  [unwired: 1 out]
          n841 = Replace Array Subset(array=w1809, new element=w1805, index=w1808) -> (w1807:dbl[])
          n842 = local write "MaxTime"(w1810) -> ()
        }
        n843 = for {
          tunnel: w1716 -> [w1799] mode=indexing
          tunnel: w1715 -> [w1789] mode=indexing
          tunnel: [w1797] -> w1714 mode=indexing
          tunnel: w1713 -> [w1796]
          tunnel: w1712 -> [w1793]
          # "4. Add the delay time according to the longest Time sequence"
          n844 = local read "MaxTime"() -> (w1790:dbl)
          n845 = Subtract(x=w1790, y=w1789) -> (x-y=w1798:dbl)
          n846 = Look In Map(map=w1796, key="None") -> (value=w1794:i32)  [unwired: 1 in, 1 out]
          n847 = Look In Map(map=w1793, key="Delay") -> (value=w1791:dbl)  [unwired: 1 in, 1 out]
          n848 = call "Add_to_sequence_SubVI_v1.vi"("Delay [us]"=w1791, "Pulse length [us]"=w1798, "Channel number"=w1794, "Array sequence in"=w1799) -> ("Array sequence out"=w1797:cluster{"Timing 0":dbl[]}[])
        }
        n849 = Merge Errors(w1690, w1688) -> (w1689:errorcluster)
        n850 = for {
          tunnel: w1714 -> [w1725]
          tunnel: w1713 -> [w1724]
          tunnel: w1712 -> [w1723]
          shift-right: [w1726] -> w1719
          shift-left: w1689 -> [w1722]
          tunnel: w1687 -> [w1721] mode=indexing
          i -> [w1720]
          n851 = for {
            shift-right: [w1744] -> w1726
            shift-left: w1722 -> [w1739]
            tunnel: w1725 -> [w1738] mode=indexing
            tunnel: w1724 -> [w1735]
            tunnel: w1723 -> [w1736]
            tunnel: w1721 -> [w1734]
            tunnel: w1720 -> [w1733]
            i -> [w1737]
            # "5. Detect the initial_state"
            # "6. Add the Process data to detect the output_state"
            n852 = call "Add_Time_Seq.vi"("Process Array"=w1734, "Initial State Array"=w1738) -> ("Total Array"=w1740:cluster{"Timing 0":dbl[]}[])  [unwired: 9 in]
            n853 = property on="Initial State Numbers" class="DigNum (strict)"() -> ("Value"=w1727:i32)  [unwired: 2 in, 2 out]
            n854 = call "Create_Time_Seq.vi"("pulses"=w1736, "Channels and actions"=w1735, "Array sequence in"=w1738) -> ("Array out"=w1742:cluster{"Timing 0":dbl[]}[][])  [unwired: 8 in]
            n855 = Multiply(x=9, y=2) -> (x*y=w1729:i32)
            n856 = Multiply(x=w1729, y=w1727) -> (x*y=w1732:i32)
            n857 = call "Create_Time_Seq.vi"("pulses"=w1736, "Channels and actions"=w1735, "Array sequence in"=w1740) -> ("Array out"=w1741:cluster{"Timing 0":dbl[]}[][])  [unwired: 8 in]
            n858 = Multiply(x=w1732, y=w1733) -> (x*y=w1731:i32)
            n859 = Insert Into Array(array=w1742, new element=w1741) -> (w1743:cluster{"Timing 0":dbl[]}[][])  [unwired: 2 in]
            n860 = for {
              tunnel: w1743 -> [w1762] mode=indexing
              shift-right: [w1755] -> w1744
              shift-left: w1739 -> [w1756]
              tunnel: w1737 -> [w1753]
              tunnel: w1731 -> [w1746]
              tunnel: w1729 -> [w1748]
              i -> [w1745]
              # "Write the full number in the name to store the data\n 1-->00001     10-->00010      100-->00100\n1000 ---> 01000   10000  -->  10000"
              n861 = local read "Config folder"() -> (w1752:string)
              n862 = Multiply(x=w1748, y=w1753) -> (x*y=w1747:i32)
              n863 = Compound Arithmetic op=ADD(w1745, w1747, w1746) -> (w1749:i32)
              n864 = Equal To 0?(x=w1749) -> (x = 0?=w1751:bool)
              n865 = case shown="False" w1751 {
                tunnel: [w1763 "00000"] -> w1750
                tunnel: w1749 -> [w1767 _]
                frame False {
                  n866 = Logarithm Base 10(1:w1767) -> (0:w1772:dbl)
                  n867 = Number To Decimal String(number=w1767, width (-)=i16 1) -> (decimal integer string=w1765:string)
                  n868 = Round Toward -Infinity(1:w1772) -> (0:w1771:dbl)
                  n869 = Subtract(x=4.0, y=w1771) -> (x-y=w1769:dbl)
                  n870 = for {
                    N: w1769 -> [_]
                    shift-right: [w1773] -> w1764
                    shift-left: "" -> [w1775]
                    n871 = Concatenate Strings(w1775, "0" ("string")) -> (w1773:string)
                  }
                  n872 = Concatenate Strings(w1764, w1765) -> (w1763:string)
                }
                frame True {
                }
              }
              n873 = call "Array_to_cluster_sequence_SubVI_v1.vi"("Array"=w1762) -> ("Sequence"=w1759:T6)
              n874 = local read "Sampling data"() -> (w1754:T2)
              n875 = Concatenate Strings(w1752, "\\process\\temp_states\\QPT_" ("string"), w1750, ".ini" ("string")) -> (w1758:string)
              n876 = call "Set_Pulse_Seq_DAQ.vi"("Time Unit"=T12 {"Time Unit"=enum."MicroSecond"}, "error in"=w1756, "Sampling data"=w1754, "Sequence"=w1759, "Filename (ini)"=w1758) -> ("error out"=w1755:errorcluster)  [unwired: 6 in]
            }
          }
        }
      }
      event "State_update": Mouse Down; "initial_state_show": Value Change {
        w1821 = "Config_Ver_2\\state_library\\"
        n877 = event-data() -> ()  [unwired: 1 in, 4 out]
        n878 = flat-sequence {
          tunnel: w1828 -> [w1836]
          tunnel: [w1835] -> w1830
          tunnel: w1821 -> [w1834]
          tunnel: [w1831] -> w1824
          tunnel: "Config_Files\\" ("string") -> [w1832]
          tunnel: w1821 -> [w1831]
          tunnel: w1830 -> [w1844]
          tunnel: "initial_state_show" -> [w1843]
          tunnel: [w1844] -> w1826
          tunnel: [w1842] -> w1825
          tunnel: w1824 -> [w1842]
          tunnel: [w1841] -> w1823
          tunnel: [w1847] -> w1827
          tunnel: w1826 -> [w1848]
          tunnel: w1825 -> [w1852]
          tunnel: w1823 -> [w1849]
          frame #0 {
            # "Open the state_library to the show the files"
            n879 = Concatenate Strings(w1832, w1834) -> (w1833:string)
            n880 = String To Path(string=w1833) -> (path=w1839:path)
            n881 = call <vilib>:"Application Directory.vi"() -> ("Application Directory"=w1840:path)
            n882 = Build Path(base path=w1840, name or relative path=w1839) -> (appended path=w1838:path)
            n883 = call <userlib>:"List Directory__ogtk.vi"("error in (no error)"=w1836, "directory path"=w1838) -> ("error out"=w1835:errorcluster, "file names"=w1837:string[])  [unwired: 2 in, 2 out]
            n884 = property on="initial_state_show" class="Ring (strict)"("Strings []"=w1837) -> ()  [unwired: 2 in, 2 out]
          }
          frame #1 {
            # "Check the initial_states in the Library"
            n885 = property on="initial_state_show" class="Ring (strict)"() -> ("Strings []"=w1845:string[])  [unwired: 2 in, 2 out]
            n886 = Index Array(array=w1845, index=w1843) -> (element=w1841:string)
            n887 = local write "Initial_state_name"(w1841) -> ()
          }
          frame #2 {
            # "Show the Pulse_Sequence"
            n888 = String Length(string=w1849) -> (length=w1851:i32)
            n889 = Concatenate Strings(w1852, w1849) -> (w1846:string)
            n890 = Greater Than 0?(x=w1851) -> (x > 0?=w1850:bool)
            n891 = case shown="True" w1850 {
              tunnel: w1846 -> [_ w1859]
              tunnel: w1848 -> [w1853 w1856]
              tunnel: [w1853 w1855] -> w1847
              frame False {
              }
              frame True {
                n892 = call "Get_Pulse_Seq_DAQ.vi"("error in"=w1856, "Filename (ini)"=w1859) -> ("error out"=w1855:errorcluster, "data"=w1858:T6)  [unwired: 8 in]
                n893 = Cluster To Array(cluster=w1858) -> (array=w1857:cluster{"Timing 0":dbl[]}[])
                n894 = for {
                  tunnel: w1857 -> [w1871] mode=indexing
                  tunnel: [w1860] -> w1854 mode=indexing
                  i -> [w1863]
                  n895 = To Double Precision Float(number=w1863) -> (double precision float=w1867:dbl)
                  n896 = Unbundle By Name(w1871) -> ("Timing 0"=w1870:dbl[])
                  n897 = Initialize Array(0.0 ("element"), 1 ("dimension size")) -> (w1864:dbl[])
                  n898 = Initialize Array(w1867, 1 ("dimension size")) -> (w1868:dbl[])
                  n899 = for {
                    tunnel: w1870 -> [w1873] mode=indexing
                    shift-right: [w1875] -> w1861
                    shift-left: w1868 -> [w1874]
                    shift-right: [w1877] -> w1862
                    shift-left: w1864 -> [w1876]
                    tunnel: w1863 -> [w1872]
                    i -> [w1882]
                    n900 = Quotient & Remainder(x=w1882, y=2) -> (x-y*floor(x/y)=w1880:i32)  [unwired: 1 out]
                    n901 = Equal To 0?(x=w1880) -> (x = 0?=w1879:bool)
                    n902 = Equal To 0?(x=w1873) -> (x = 0?=w1878:bool)
                    n903 = case shown="True" w1879 {
                      tunnel: w1878 -> [_ w1899]
                      tunnel: [w1883 w1898] -> w1877
                      tunnel: w1876 -> [w1885 w1897]
                      tunnel: [w1890 w1896] -> w1875
                      tunnel: w1874 -> [w1891 w1895]
                      tunnel: w1873 -> [w1886 w1894]
                      tunnel: w1872 -> [w1892 w1893]
                      frame False {
                        n904 = Array Size(array=w1885) -> (size(s)=w1889:i32)
                        n905 = Decrement(x=w1889) -> (x-1=w1888:i32)
                        n906 = Index Array(array=w1885, index=w1888) -> (element=w1887:dbl)
                        n907 = Build Array (concatenate)(w1891, w1892) -> (w1890:dbl[])
                        n908 = Add(x=w1886, y=w1887) -> (x+y=w1884:dbl)
                        n909 = Build Array (concatenate)(w1885, w1884) -> (w1883:dbl[])
                      }
                      frame True {
                        n910 = case shown="False" w1899 {
                          tunnel: [w1910 w1915] -> w1898
                          tunnel: w1897 -> [w1904 w1915]
                          tunnel: [w1906 w1914] -> w1896
                          tunnel: w1895 -> [w1913 w1914]
                          tunnel: w1894 -> [w1911 _]
                          tunnel: w1893 -> [w1907 _]
                          frame False {
                            n911 = Array Size(array=w1904) -> (size(s)=w1912:i32)
                            n912 = Add(x=0.5, y=w1907) -> (x+y=w1908:dbl)
                            n913 = Decrement(x=w1912) -> (x-1=w1905:i32)
                            n914 = Index Array(array=w1904, index=w1905) -> (element=w1902:dbl)
                            n915 = Add(x=w1911, y=w1902) -> (x+y=w1901:dbl)
                            n916 = Decrement(x=w1902) -> (x-1=w1903:dbl)
                            n917 = Build Array (concatenate)(w1913, w1907, w1908, w1908, w1907) -> (w1906:dbl[])
                            n918 = Decrement(x=w1901) -> (x-1=w1900:dbl)
                            n919 = Build Array (concatenate)(w1904, w1903, w1902, w1900, w1901) -> (w1910:dbl[])
                          }
                          frame True {
                          }
                        }
                      }
                    }
                  }
                  n920 = Bundle(w1862, w1861) -> (w1860:cluster{dbl[], dbl[]})  [unwired: 1 in]
                }
                "Pulses chart 2" <- w1854
              }
            }
          }
        }
      }
      event "Process_update": Mouse Down; "Process_show": Value Change {
        n921 = event-data() -> ()  [unwired: 1 in, 4 out]
        n922 = flat-sequence {
          tunnel: w1923 -> [w1930]
          tunnel: [w1929] -> w1925
          tunnel: "Config_Ver_2\\process_library\\" -> [w1926]
          tunnel: [w1926] -> w1919
          tunnel: "Config_Files\\" ("string") -> [w1927]
          tunnel: w1925 -> [w1938]
          tunnel: "Process_show" -> [w1937]
          tunnel: [w1938] -> w1921
          tunnel: [w1936] -> w1920
          tunnel: w1919 -> [w1936]
          tunnel: [w1935] -> w1918
          tunnel: w1921 -> [w1946]
          tunnel: w1920 -> [w1943]
          tunnel: w1918 -> [w1942]
          tunnel: [w1945] -> w1916
          frame #0 {
            # "Open the processes to the show the files"
            n923 = Concatenate Strings(w1927, w1926) -> (w1928:string)
            n924 = String To Path(string=w1928) -> (path=w1933:path)
            n925 = call <vilib>:"Application Directory.vi"() -> ("Application Directory"=w1934:path)
            n926 = Build Path(base path=w1934, name or relative path=w1933) -> (appended path=w1932:path)
            n927 = call <userlib>:"List Directory__ogtk.vi"("error in (no error)"=w1930, "directory path"=w1932) -> ("error out"=w1929:errorcluster, "file names"=w1931:string[])  [unwired: 2 in, 2 out]
            n928 = property on="Process_show" class="Ring (strict)"("Strings []"=w1931) -> ()  [unwired: 2 in, 2 out]
          }
          frame #1 {
            n929 = property on="Process_show" class="Ring (strict)"() -> ("Strings []"=w1939:string[])  [unwired: 2 in, 2 out]
            n930 = Index Array(array=w1939, index=w1937) -> (element=w1935:string)
            n931 = local write "Process name"(w1935) -> ()
          }
          frame #2 {
            n932 = String Length(string=w1942) -> (length=w1944:i32)
            n933 = Concatenate Strings(w1943, w1942) -> (w1940:string)
            n934 = Greater Than 0?(x=w1944) -> (x > 0?=w1941:bool)
            n935 = case shown="False" w1941 {
              tunnel: w1940 -> [_ w1953]
              tunnel: w1946 -> [w1947 w1950]
              tunnel: [w1947 w1949] -> w1945
              frame False {
              }
              frame True {
                n936 = call "Get_Pulse_Seq_DAQ.vi"("error in"=w1950, "Filename (ini)"=w1953) -> ("error out"=w1949:errorcluster, "data"=w1952:T6)  [unwired: 8 in]
                n937 = Cluster To Array(cluster=w1952) -> (array=w1951:cluster{"Timing 0":dbl[]}[])
                n938 = for {
                  tunnel: w1951 -> [w1965] mode=indexing
                  tunnel: [w1954] -> w1948 mode=indexing
                  i -> [w1957]
                  n939 = To Double Precision Float(number=w1957) -> (double precision float=w1961:dbl)
                  n940 = Unbundle By Name(w1965) -> ("Timing 0"=w1964:dbl[])
                  n941 = Initialize Array(0.0 ("element"), 1 ("dimension size")) -> (w1958:dbl[])
                  n942 = Initialize Array(w1961, 1 ("dimension size")) -> (w1962:dbl[])
                  n943 = for {
                    tunnel: w1964 -> [w1967] mode=indexing
                    shift-right: [w1969] -> w1955
                    shift-left: w1962 -> [w1968]
                    shift-right: [w1971] -> w1956
                    shift-left: w1958 -> [w1970]
                    tunnel: w1957 -> [w1966]
                    i -> [w1976]
                    n944 = Quotient & Remainder(x=w1976, y=2) -> (x-y*floor(x/y)=w1974:i32)  [unwired: 1 out]
                    n945 = Equal To 0?(x=w1974) -> (x = 0?=w1973:bool)
                    n946 = Equal To 0?(x=w1967) -> (x = 0?=w1972:bool)
                    n947 = case shown="False" w1973 {
                      tunnel: w1972 -> [_ w1993]
                      tunnel: [w1977 w1992] -> w1971
                      tunnel: w1970 -> [w1979 w1991]
                      tunnel: [w1984 w1990] -> w1969
                      tunnel: w1968 -> [w1985 w1989]
                      tunnel: w1967 -> [w1980 w1988]
                      tunnel: w1966 -> [w1986 w1987]
                      frame False {
                        n948 = Array Size(array=w1979) -> (size(s)=w1983:i32)
                        n949 = Decrement(x=w1983) -> (x-1=w1982:i32)
                        n950 = Index Array(array=w1979, index=w1982) -> (element=w1981:dbl)
                        n951 = Build Array (concatenate)(w1985, w1986) -> (w1984:dbl[])
                        n952 = Add(x=w1980, y=w1981) -> (x+y=w1978:dbl)
                        n953 = Build Array (concatenate)(w1979, w1978) -> (w1977:dbl[])
                      }
                      frame True {
                        n954 = case shown="True" w1993 {
                          tunnel: [w2004 w2009] -> w1992
                          tunnel: w1991 -> [w1998 w2009]
                          tunnel: [w2000 w2008] -> w1990
                          tunnel: w1989 -> [w2007 w2008]
                          tunnel: w1988 -> [w2005 _]
                          tunnel: w1987 -> [w2001 _]
                          frame False {
                            n955 = Array Size(array=w1998) -> (size(s)=w2006:i32)
                            n956 = Add(x=0.5, y=w2001) -> (x+y=w2002:dbl)
                            n957 = Decrement(x=w2006) -> (x-1=w1999:i32)
                            n958 = Index Array(array=w1998, index=w1999) -> (element=w1996:dbl)
                            n959 = Add(x=w2005, y=w1996) -> (x+y=w1995:dbl)
                            n960 = Decrement(x=w1996) -> (x-1=w1997:dbl)
                            n961 = Build Array (concatenate)(w2007, w2001, w2002, w2002, w2001) -> (w2000:dbl[])
                            n962 = Decrement(x=w1995) -> (x-1=w1994:dbl)
                            n963 = Build Array (concatenate)(w1998, w1997, w1996, w1994, w1995) -> (w2004:dbl[])
                          }
                          frame True {
                          }
                        }
                      }
                    }
                  }
                  n964 = Bundle(w1956, w1955) -> (w1954:cluster{dbl[], dbl[]})  [unwired: 1 in]
                }
                "Pulses chart 3" <- w1948
              }
            }
          }
        }
      }
      event "Choose init states": Mouse Down {
        n965 = event-data() -> ()  [unwired: 1 in, 8 out]
        n966 = local read "Initial_state_name"() -> (w2019:string)
        n967 = local read "Config folder"() -> (w2010:string)
        n968 = String Length(string=w2019) -> (length=w2020:i32)
        n969 = Greater Than 0?(x=w2020) -> (x > 0?=w2011:bool)
        n970 = Concatenate Strings(w2010, "\\state_library\\", w2019) -> (w2013:string)
        n971 = Concatenate Strings(w2010, "\\process\\init_states_sets\\") -> (w2017:string)
        n972 = case shown="True" w2011 {
          tunnel: w2021 -> [w2022 w2032]
          tunnel: w2019 -> [_ w2031]
          tunnel: w2017 -> [_ w2030]
          tunnel: [w2022 w2029] -> w2015
          tunnel: w2013 -> [_ w2028]
          frame False {
          }
          frame True {
            n973 = call "Get_Pulse_Seq_DAQ.vi"("error in"=w2032, "Filename (ini)"=w2028) -> ("error out"=w2026:errorcluster, "data"=w2027:T6)  [unwired: 8 in]
            n974 = local read "Sampling data"() -> (w2025:T2)
            n975 = Concatenate Strings(w2030, w2031) -> (w2023:string)
            n976 = call "Set_Pulse_Seq_DAQ.vi"("Time Unit"=T12 {"Time Unit"=enum."MicroSecond"}, "error in"=w2026, "Sampling data"=w2025, "Sequence"=w2027, "Filename (ini)"=w2023) -> ("error out"=w2029:errorcluster)  [unwired: 6 in]
          }
        }
        n977 = call "Read_filename.vi"("error in"=w2015, "Filename (ini)"=w2017) -> ("error out"=w2016:errorcluster, "Strings []"=w2018:string[])  [unwired: 8 in]
        n978 = local write "State_List"(w2018) -> ()
      }
      event "Choose the Process": Mouse Down {
        n979 = event-data() -> ()  [unwired: 1 in, 8 out]
        n980 = local read "Process name"() -> (w2042:string)
        n981 = local read "Config folder"() -> (w2033:string)
        n982 = String Length(string=w2042) -> (length=w2043:i32)
        n983 = Greater Than 0?(x=w2043) -> (x > 0?=w2034:bool)
        n984 = Concatenate Strings(w2033, "\\process_library\\", w2042) -> (w2036:string)
        n985 = Concatenate Strings(w2033, "\\process\\processes_sets\\") -> (w2040:string)
        n986 = case shown="True" w2034 {
          tunnel: w2044 -> [w2045 w2055]
          tunnel: w2042 -> [_ w2054]
          tunnel: w2040 -> [_ w2053]
          tunnel: [w2045 w2052] -> w2038
          tunnel: w2036 -> [_ w2051]
          frame False {
          }
          frame True {
            n987 = call "Get_Pulse_Seq_DAQ.vi"("error in"=w2055, "Filename (ini)"=w2051) -> ("error out"=w2049:errorcluster, "data"=w2050:T6)  [unwired: 8 in]
            n988 = local read "Sampling data"() -> (w2048:T2)
            n989 = Concatenate Strings(w2053, w2054) -> (w2046:string)
            n990 = call "Set_Pulse_Seq_DAQ.vi"("Time Unit"=T12 {"Time Unit"=enum."MicroSecond"}, "error in"=w2049, "Sampling data"=w2048, "Sequence"=w2050, "Filename (ini)"=w2046) -> ("error out"=w2052:errorcluster)  [unwired: 6 in]
          }
        }
        n991 = call "Read_filename.vi"("error in"=w2038, "Filename (ini)"=w2040) -> ("error out"=w2039:errorcluster, "Strings []"=w2041:string[])  [unwired: 8 in]
        n992 = local write "Process_List"(w2041) -> ()
      }
      event "Delete init states": Mouse Down {
        # "Check the name if it's in the State_list, if yes, the name will be deleted, otherwise, return"
        n993 = event-data() -> ()  [unwired: 1 in, 8 out]
        n994 = local read "Initial_state_name"() -> (w2061:string)
        n995 = local read "Config folder"() -> (w2056:string)
        n996 = local read "State_List"() -> (w2063:string[])
        n997 = Concatenate Strings(w2056, "\\process\\init_states_sets\\") -> (w2064:string)
        n998 = for {
          tunnel: w2063 -> [w2076] mode=indexing
          shift-right: [w2072] -> w2060
          shift-left: FALSE -> [w2073]
          tunnel: w2061 -> [w2075]
          n999 = Equal?(x=w2075, y=w2076) -> (x = y?=w2074:bool)
          n1000 = Or(x=w2073, y=w2074) -> (x .or. y?=w2072:bool)
        }
        n1001 = Concatenate Strings(w2064, w2061) -> (w2057:string)
        n1002 = case shown="True" w2060 {
          tunnel: w2059 -> [w2068 w2069]
          tunnel: [w2068 w2071] -> w2058
          tunnel: w2057 -> [_ w2070]
          frame False {
          }
          frame True {
            n1003 = call "Delete_file.vi"("error in"=w2069, "Filename (ini)"=w2070) -> ("error out"=w2071:errorcluster)  [unwired: 9 in]
          }
        }
        n1004 = call "Read_filename.vi"("error in"=w2058, "Filename (ini)"=w2064) -> ("error out"=w2066:errorcluster, "Strings []"=w2067:string[])  [unwired: 8 in]
        n1005 = local write "State_List"(w2067) -> ()
      }
      event "Delete the Process": Mouse Down {
        # "Check the name if it's in the State_list, if yes, the name will be deleted, otherwise, return"
        n1006 = event-data() -> ()  [unwired: 1 in, 8 out]
        n1007 = local read "Process name"() -> (w2082:string)
        n1008 = local read "Config folder"() -> (w2077:string)
        n1009 = local read "Process_List"() -> (w2084:string[])
        n1010 = Concatenate Strings(w2077, "\\process\\processes_sets\\") -> (w2085:string)
        n1011 = for {
          tunnel: w2084 -> [w2097] mode=indexing
          shift-right: [w2093] -> w2081
          shift-left: FALSE -> [w2094]
          tunnel: w2082 -> [w2096]
          n1012 = Equal?(x=w2096, y=w2097) -> (x = y?=w2095:bool)
          n1013 = Or(x=w2094, y=w2095) -> (x .or. y?=w2093:bool)
        }
        n1014 = Concatenate Strings(w2085, w2082) -> (w2078:string)
        n1015 = case shown="True" w2081 {
          tunnel: w2080 -> [w2089 w2090]
          tunnel: [w2089 w2092] -> w2079
          tunnel: w2078 -> [_ w2091]
          frame False {
          }
          frame True {
            n1016 = call "Delete_file.vi"("error in"=w2090, "Filename (ini)"=w2091) -> ("error out"=w2092:errorcluster)  [unwired: 9 in]
          }
        }
        n1017 = call "Read_filename.vi"("error in"=w2079, "Filename (ini)"=w2085) -> ("error out"=w2087:errorcluster, "Strings []"=w2088:string[])  [unwired: 8 in]
        n1018 = local write "Process_List"(w2088) -> ()
      }
      event "Clear All states": Mouse Down {
        n1019 = event-data() -> ()  [unwired: 1 in, 8 out]
        n1020 = local read "Config folder"() -> (w2105:string)
        n1021 = local read "State_List"() -> (w2104:string[])
        n1022 = Concatenate Strings(w2105, "\\process\\init_states_sets\\") -> (w2099:string)
        n1023 = Array Size(array=w2104) -> (size(s)=w2103:i32)
        n1024 = Greater Than 0?(x=w2103) -> (x > 0?=w2102:bool)
        n1025 = flat-sequence {
          tunnel: w2099 -> [w2111]
          tunnel: w2104 -> [w2110]
          tunnel: w2102 -> [w2109]
          tunnel: w2101 -> [w2108]
          tunnel: [w2107] -> w2100
          tunnel: w2100 -> [w2124]
          tunnel: w2099 -> [w2123]
          tunnel: [w2122] -> w2098
          frame #0 {
            n1026 = case shown="False" w2109 {
              tunnel: w2111 -> [_ w2116]
              tunnel: w2110 -> [_ w2115]
              tunnel: w2108 -> [w2112 w2114]
              tunnel: [w2112 w2113] -> w2107
              frame False {
              }
              frame True {
                n1027 = for {
                  tunnel: w2115 -> [w2120] mode=indexing
                  tunnel: w2116 -> [w2121]
                  shift-right: [w2117] -> w2113
                  shift-left: w2114 -> [w2118]
                  n1028 = Concatenate Strings(w2121, w2120) -> (w2119:string)
                  n1029 = call "Delete_file.vi"("error in"=w2118, "Filename (ini)"=w2119) -> ("error out"=w2117:errorcluster)  [unwired: 9 in]
                }
              }
            }
          }
          frame #1 {
            n1030 = call "Read_filename.vi"("error in"=w2124, "Filename (ini)"=w2123) -> ("error out"=w2122:errorcluster, "Strings []"=w2125:string[])  [unwired: 8 in]
            n1031 = local write "State_List"(w2125) -> ()
          }
        }
      }
      event "Clear All processes": Mouse Down {
        n1032 = event-data() -> ()  [unwired: 1 in, 8 out]
        n1033 = local read "Config folder"() -> (w2133:string)
        n1034 = local read "Process_List"() -> (w2132:string[])
        n1035 = Concatenate Strings(w2133, "\\process\\processes_sets\\") -> (w2127:string)
        n1036 = Array Size(array=w2132) -> (size(s)=w2131:i32)
        n1037 = Greater Than 0?(x=w2131) -> (x > 0?=w2130:bool)
        n1038 = flat-sequence {
          tunnel: w2127 -> [w2139]
          tunnel: w2132 -> [w2138]
          tunnel: w2130 -> [w2137]
          tunnel: w2129 -> [w2136]
          tunnel: [w2135] -> w2128
          tunnel: w2128 -> [w2152]
          tunnel: w2127 -> [w2151]
          tunnel: [w2150] -> w2126
          frame #0 {
            n1039 = case shown="True" w2137 {
              tunnel: w2139 -> [_ w2144]
              tunnel: w2138 -> [_ w2143]
              tunnel: w2136 -> [w2140 w2142]
              tunnel: [w2140 w2141] -> w2135
              frame False {
              }
              frame True {
                n1040 = for {
                  tunnel: w2143 -> [w2148] mode=indexing
                  tunnel: w2144 -> [w2149]
                  shift-right: [w2145] -> w2141
                  shift-left: w2142 -> [w2146]
                  n1041 = Concatenate Strings(w2149, w2148) -> (w2147:string)
                  n1042 = call "Delete_file.vi"("error in"=w2146, "Filename (ini)"=w2147) -> ("error out"=w2145:errorcluster)  [unwired: 9 in]
                }
              }
            }
          }
          frame #1 {
            n1043 = call "Read_filename.vi"("error in"=w2152, "Filename (ini)"=w2151) -> ("error out"=w2150:errorcluster, "Strings []"=w2153:string[])  [unwired: 8 in]
            n1044 = local write "Process_List"(w2153) -> ()
          }
        }
      }
      event "Show init state": Mouse Down {
        n1045 = event-data() -> ()  [unwired: 1 in, 8 out]
        n1046 = local read "Config folder"() -> (w2154:string)
        n1047 = Concatenate Strings(w2154, "\\process\\init_states_sets\\") -> (w2158:string)
        n1048 = call "Read_filename.vi"("error in"=w2157, "Filename (ini)"=w2158) -> ("error out"=w2156:errorcluster, "Strings []"=w2155:string[])  [unwired: 8 in]
        n1049 = local write "State_List"(w2155) -> ()
      }
      event "Show Process_List": Mouse Down {
        n1050 = event-data() -> ()  [unwired: 1 in, 8 out]
        n1051 = local read "Config folder"() -> (w2160:string)
        n1052 = Concatenate Strings(w2160, "\\process\\processes_sets\\") -> (w2164:string)
        n1053 = call "Read_filename.vi"("error in"=w2163, "Filename (ini)"=w2164) -> ("error out"=w2162:errorcluster, "Strings []"=w2161:string[])  [unwired: 8 in]
        n1054 = local write "Process_List"(w2161) -> ()
      }
      event "Reset sequence": Mouse Down {
        n1055 = event-data() -> ()  [unwired: 1 in, 8 out]
        n1056 = Wait (ms)(milliseconds to wait=u32 150) -> ()  [unwired: 1 out]
      }
    }
  }
